vi "AcqControl.vi"(3 "Debug Mode?":bool, 4 "Digitizer Settings":T13={"Digitizer delay (us) "=0.0, "rf points per line"=2048, "lines per plane"=128, "Samp Rate (Hz)"=100000000.0, "Additional dig delay (us)"=0.0, "Voltage Scale"=0.4, "Pre-Looks"=0, "Offset delay (us)"=0.0, "bits A/D"=8, "Avg Num"=1, "DigTimeOut"=5.0, "Rel Dig Delay"=0.0, "Dig Ch"=0, "LeCroyCluster"={"LeCroy Channels"=[TRUE, FALSE, FALSE, FALSE], "LC read pt offset"=0.0, "Sweep Avg"=FALSE}, "Main Digitizer"=enum."NI Digitizer", "Dig Config"=enum."Single channel", "Digitizer ID Cluster"={"Acqiris/Alazar/SP ID"=[], "NI Instr Handles"=[], "LeCroy VISA"="", "GaGe Handle"={"Handle"=0, "Sample size"=0, "Resolution"=0, "Offset"=0, "Channels"=0, "Boards"=0}, "ATS Ref"="ATS9350", "Acqiris Address"=["PCI::INSTR0"], "ADQRef"=refnum, "adq_cu_ptr"=refnum}, "Trigger Settings"={"Trig Source"=1, "Trig Coupling"=0, "Trig Slope"=0, "Level (mV)"=1500.0}, "Bulk Acq"=FALSE, "Bulk Start Indexes"=[], "Data Ref RF"=refnum, "NI ID/Channel"=[], "Total Dig CH"=1, "Xtra Ann Trig delay (us)"=10.0, "Fix Z Delay?"=FALSE, "One Way Transmission?"=FALSE, "Data Ref Log"=refnum} {"Trigger Settings"."Trig Slope" items=["Positive", "Negative"]; "Trigger Settings"."Level (mV)" format="%.2f"; "Trigger Settings"."Trig Coupling" items=["DC 1 MOhm", "AC 1 MOhm", "DC 50 Ohm", "AC 50 Ohm"]; "Trigger Settings"."Trig Source" items=["Chan 1", "External"]; "Rel Dig Delay" format="%.2f"; "DigTimeOut" format="%.2f"; "Avg Num" min=1; "Offset delay (us)" format="%.2f"; "Additional dig delay (us)" format="%.2f"; "Digitizer delay (us)" format="%.2f"}, 5 "Motion Settings In":T10={"No Motion?"=FALSE, "Motion System"=enum."NI 735x", "Motion Bd ID"=1, "Motion Profile"="SMAC1", "# Axis"=1, "Reverse Z axis?"=TRUE, "SMAC Axis"=0, "scan pair"=enum."y-(x) scan", "RT fps"=6.0, "Steps per mm"=[1000, 1000, 1000, 1000], "Motor Parameters"={"velocity ct/s"=[10000.0, 10000.0, 10000.0, 50000.0], "accel ct/s^2"=[50000.0, 50000.0, 50000.0, 200000.0]}, "One Way Scan"=FALSE, "Reverse One Way Scan"=FALSE, "Global Position (mm)"=[], "Plane"=0, "Distance between\nscan lines (um)"=0.0, "Distance between\nscan planes (um)"=0.0, "number of scan planes"=1, "Total steps in line"=0, "Xtra plane\ndistance  (um)"=100, "Xtra planes "=1, "Add Axis"=FALSE, "overshoot cts"=200, "BKPT Shift"=0, "Scan Start Time (ms)"=0, "ESP VISA"="GPIB::1::INSTR", "3rd Axis"=1, "GL Ref Out"=refnum, "Galil Address"=""} {"3rd Axis" items=["x", "y", "z", "w"]; "Xtra planes" min=1; "Xtra plane\ndistance  (um)" min=0; "Distance between\nscan planes (um)" format="%.2f"; "Distance between\nscan lines (um)" format="%.2f"; "SMAC Axis" items=["None"=0, "Axis 1"=1, "Axis 2"=2, "Axis 3"=3, "Axis 4"=4, "Axis 5"=5, "Axis 6"=6, "Axis 7"=7, "Axis 8"=8, "Vector Space 1"=17, "Vector Space 2"=18, "Vector Space 3"=19, "Vector Space 4"=20]; "Motion Bd ID" min=1 max=32 step=1}) -> (1 "Digitizer Settings Out":T13={"Digitizer delay (us) "=0.0, "rf points per line"=2048, "lines per plane"=128, "Samp Rate (Hz)"=100000000.0, "Additional dig delay (us)"=0.0, "Voltage Scale"=0.4, "Pre-Looks"=0, "Offset delay (us)"=0.0, "bits A/D"=8, "Avg Num"=1, "DigTimeOut"=5.0, "Rel Dig Delay"=0.0, "Dig Ch"=0, "LeCroyCluster"={"LeCroy Channels"=[TRUE, FALSE, FALSE, FALSE], "LC read pt offset"=0.0, "Sweep Avg"=FALSE}, "Main Digitizer"=enum."NI Digitizer", "Dig Config"=enum."Single channel", "Digitizer ID Cluster"={"Acqiris/Alazar/SP ID"=[], "NI Instr Handles"=[], "LeCroy VISA"="", "GaGe Handle"={"Handle"=0, "Sample size"=0, "Resolution"=0, "Offset"=0, "Channels"=0, "Boards"=0}, "ATS Ref"="ATS9350", "Acqiris Address"=["PCI::INSTR0"], "ADQRef"=refnum, "adq_cu_ptr"=refnum}, "Trigger Settings"={"Trig Source"=1, "Trig Coupling"=0, "Trig Slope"=0, "Level (mV)"=1500.0}, "Bulk Acq"=FALSE, "Bulk Start Indexes"=[], "Data Ref RF"=refnum, "NI ID/Channel"=[], "Total Dig CH"=1, "Xtra Ann Trig delay (us)"=10.0, "Fix Z Delay?"=FALSE, "One Way Transmission?"=FALSE, "Data Ref Log"=refnum} {"Trigger Settings"."Trig Slope" items=["Positive", "Negative"]; "Trigger Settings"."Level (mV)" format="%.2f"; "Trigger Settings"."Trig Coupling" items=["DC 1 MOhm", "AC 1 MOhm", "DC 50 Ohm", "AC 50 Ohm"]; "Trigger Settings"."Trig Source" items=["Chan 1", "External"]; "Rel Dig Delay" format="%.2f"; "DigTimeOut" format="%.2f"; "Avg Num" min=1; "Offset delay (us)" format="%.2f"; "Additional dig delay (us)" format="%.2f"; "Digitizer delay (us)" format="%.2f"}, 2 "Motion Settings Out":T10={"No Motion?"=FALSE, "Motion System"=enum."NI 735x", "Motion Bd ID"=1, "Motion Profile"="SMAC1", "# Axis"=1, "Reverse Z axis?"=TRUE, "SMAC Axis"=0, "scan pair"=enum."y-(x) scan", "RT fps"=6.0, "Steps per mm"=[1000, 1000, 1000, 1000], "Motor Parameters"={"velocity ct/s"=[10000.0, 10000.0, 10000.0, 50000.0], "accel ct/s^2"=[50000.0, 50000.0, 50000.0, 200000.0]}, "One Way Scan"=FALSE, "Reverse One Way Scan"=FALSE, "Global Position (mm)"=[], "Plane"=0, "Distance between\nscan lines (um)"=0.0, "Distance between\nscan planes (um)"=0.0, "number of scan planes"=1, "Total steps in line"=0, "Xtra plane\ndistance  (um)"=100, "Xtra planes "=1, "Add Axis"=FALSE, "overshoot cts"=200, "BKPT Shift"=0, "Scan Start Time (ms)"=0, "ESP VISA"="GPIB::1::INSTR", "3rd Axis"=1, "GL Ref Out"=refnum, "Galil Address"=""} {"3rd Axis" items=["x", "y", "z", "w"]; "Xtra planes" min=1; "Xtra plane\ndistance  (um)" min=0; "Distance between\nscan planes (um)" format="%.2f"; "Distance between\nscan lines (um)" format="%.2f"; "SMAC Axis" items=["None"=0, "Axis 1"=1, "Axis 2"=2, "Axis 3"=3, "Axis 4"=4, "Axis 5"=5, "Axis 6"=6, "Axis 7"=7, "Axis 8"=8, "Vector Space 1"=17, "Vector Space 2"=18, "Vector Space 3"=19, "Vector Space 4"=20]; "Motion Bd ID" min=1 max=32 step=1})   [LabVIEW 2022 SP3]
uses:
  Controls/ScanType2.ctl
  Motion Controllers/-MotionRoutines/ScanAxis.ctl
  ViewData/-ReadEye/ScaleMethod.ctl
  ViewData/-ReadEye/TypeDefs/TypeofMean.ctl
  Digitizers/-DigitizerRoutines/DigitizerSettings.ctl
  Digitizers/-DigitizerRoutines/Digitizer.ctl
  Digitizers/-DigitizerRoutines/DigConfig.ctl
  Digitizers/-DigitizerRoutines/DigitizerID.ctl
  C:/Windows/System32/ADQAPI_dotNet_helper.dll
  Motion Controllers/NI_controller/-NI_MotionRoutines/MotionParameters.ctl
  Motion Controllers/NI_controller/-NI_MotionRoutines/MotionSys.ctl
  Motion Controllers/-MotionRoutines/3rdAxis.ctl
  Annular Array/-AnnularRoutines/TransGeometry.ctl
  Annular Array/-AnnularRoutines/ArrayGeometry.ctl
  Controls/HF_XDCRs.ctl
  TransducerCal/-CalTransducer/HydrophoneSettings.ctl
  TransducerCal/-CalTransducer/Hydros.ctl
  <vilib>/Utility/miscctls.llb/LVRectTypeDef.ctl
  Controls/location.ctl
  <vilib>/Analysis/baseanly.llb/Quick Scale 2D.vi
  Motion Controllers/-MotionRoutines/MotionGlobals.vi
  Switch Modules/SwitchGlobals.vi
  Annular Array/-AnnularRoutines/AnnularArrayGlobal.vi
  Pulsers/PulserGlobals.vi
  Digitizers/-DigitizerRoutines/DigitizerGlobals.vi
  <vilib>/DAQmx/create/channels.llb/DAQmx Create Channel (CO-Pulse Generation-Frequency).vi
  <vilib>/DAQmx/configure/timing.llb/DAQmx Timing (Implicit).vi
  <vilib>/Analysis/NI_AALBase.lvlib
  <vilib>/Platform/NI_3dgraph.lvlib
  <instrlib>/niSwitch/niSwitch.llb/niSwitch Connect Channels (Single).vi
panel:
  out "Length of\nall planes (mm) Temp":dbl=128.0 format="%.2f"
  out "Digitizer delay (us) (Temp)":dbl
  in  "Auto Vz Depth":dbl=0.04 format="%.2f"
  in  "Pulse":bool
  in  "Length of Z \nScan (mm)":dbl=4.0 format="%#_13g"
  in  "Distance between\nZ planes (um)":i32=50
  in  "DBSP2":sgl
  in  "DBSP1":sgl
  out "Scan Size":dbl[](array[numeric])
  in  "Attenuation Scan":bool
  in  "Parameter Selection":u16(ring) items=["Neg Peak (V)", "Pos Peak  (V)", "Peak to Peak  (V)", "RMS  (V)", "Neg Peak Pressure (MPa)", "p.3 (MPa)", "Ipa (W/cm^2)", "Ipa.3 (W/cm^2)", "Ita (W/cm^2)", "Ita.3 (W/cm^2)"]
  out "Scan data":T1 {"Pulse Parameters"."pos peak pressure (MPa)" format="%.2f"; "axis 2 ticks" format="%.2f"; "axis 1 ticks" format="%.2f"; "step size" format="%.2f"; "axis2o" format="%.2f"; "axis1o" format="%.2f"; "scan data" format="%.2f"}
  in  "Pressure Cal Parameters":T2={"Center Freq (MHz)"=0.0, "PRF (kHz)"=1.0, "Pulse window (us)"=0.0, "Hydrophone"=enum."PAL #1048", "booster amp?"=TRUE} {"Pulse window (us)" format="%.2f"; "PRF (kHz)" format="%.2f"; "Center Freq (MHz)" format="%.2f"}
  in  "Plot":enum32{"1-D", "2-D"}(tab)
  out "Hydrophopne Waveform Graph":T4(graph)
  in  "3D Surface":refnum<k7>(container)
  in  "3rd Axis":T5=1 items=["x", "y", "z", "w"]
  in  "Fill":bool
  in  "1-to-1":bool
  in  "Auto Vz?":bool=TRUE
  out "LC read pt offset temp":dbl
  out "rf points per line Temp":i32
  out "Additional dig delay (us) Temp":dbl
  in  "New Sample":bool
  in  "Next Scan":bool
  in  "HF XDCR":T6
  in  "Microscopy Scan Mode":T7(radio)
  in  "Take Webcam pic":bool
  in  "Save Scan Settings":bool
  in  "Load Scan Settings":bool
  in  "Flip Y":bool
  in  "Flip X":bool
  in  "Transpose":bool
  in  "Trans Geometry (mm)":T8={"Transducer"=0, "Geo Focus"=12.0, "a (radius)"=3.0, "# of rings"=5, "kerf space "=0.1, "Center Freq"=12.0} {"Transducer" items=["6D 12R 40 MHz"=0, "10D 31R 20 MHz"=1, "10D 23R 20 MHz"=2, "6D 23R 40 MHz"=3, "4.5D 10.7R 40 MHz"=4, "9D 23.5R 20 MHz"=5, "9D 25.8R 20MHz"=6, "Enter"=99]}
  out "error out":errorcluster
  in  "2nd Channel HZ Offset?":bool
  in  "Read HZ Offset?":bool
  in  "Reverse One \nWay Scan":bool
  in  "Skip Real Time Setup":bool
  in  "VISA session 2":refnum<visa-resource-name>
  out "Cross plane\nlength (mm)":dbl=128.0 format="%.2f"
  in  "Xtra planes":i32=1 min=1
  in  "Xtra plane\ndistance  (um)":i32=100 min=0
  out "File":string
  in  "Filter Prams":T17={"low cutoff"=25, "order"=81, "high cutoff"=55}
  in  "OPTIONS":T18(tab)=enum."Array Other"
  in  "View EYE":bool
  in  "CH2?":bool
  out "RT V":i32
  out "Trig (Hz)":dbl
  in  "Compress":bool
  in  "C MIP":bool
  in  "MIP Thresh":sgl=15.0
  in  "Multi Trig#":i32=1 min=1
  in  "Multi Trig":bool
  in  "Multi Time (us)":sgl=250.0 min=250
  in  "Resp Wait (ms)":u32=400
  in  "Dopp\nGate?":bool
  in  "Add Axis":bool
  in  "Resp Divide":i32=2 min=1
  in  "USB Gate\nPer Sample":bool
  in  "Transfer to FTP":bool
  in  "DAQ Range":cluster{"Max V":dbl, "Min V":dbl}={"Max V"=1.0, "Min V"=-1.0} {"Max V" format="%0.2f"; "Min V" format="%0.2f"}
  in  "LeCroy Channels":bool[](array[boolean])=[TRUE, FALSE, FALSE, FALSE]
  in  "CTR PRF?":bool=TRUE
  in  "Save Temp":bool
  in  "Sweep\nAvg":bool
  in  "c mm/mics":sgl=1.485
  in  "Bulk Acq":bool
  in  "Full Array Scan?":bool
  in  "BKPT Shift":i32
  in  "Xtra delay (us)":dbl=3.0
  in  "Sub Ap Excite?":bool
  in  "RT fps":sgl=12.0 min=0.001 max=30 format="%#_2f"
  in  "Xmt/Rcv":cluster{"XMIT":bool[], "RCV":bool[]}={"XMIT"=[TRUE, TRUE, TRUE, TRUE, TRUE], "RCV"=[TRUE, TRUE, TRUE, TRUE, TRUE]}
  in  "Save TIFF?":bool
  in  "GPU?":bool
  in  "DownFactor":i32=1 min=1
  in  "RCV 1CH":u16(ring) items=["All", "1", "2", "3", "4", "5"]
  in  "Set Spectrometer":bool
  in  "Overshoot":i32=200 min=0 max=10000
  in  "One Way Scan":bool
  in  "TimeOut (s)":sgl=5.0 min=0 format="%_2f"
  in  "scan pair":T12=enum."x-(y) scan"
  out "View path":path
  in  "Type of Mean":T19=enum."No mean"
  in  "Display mode":T20=enum."Log Grey Scale"
  in  "distance?":bool
  in  "ExitSendCmd":bool
  in  "Email":string
  in  "Drive Voltages":sgl[](array[numeric])=[100.0] format="%#_3g"
  in  "Burst Ct":i8[](array[numeric])=[10, 15, 20]
  in  "CA Threshold":i16=15
  in  "Focal Zones":i16=41
  in  "Fix Z Delay?":bool
  out "Estimated Line spacing":dbl=1.0
  in  "Man Cont":bool
  in  "Auto\nScale":bool=TRUE
  out "Waveform Graph":sgl[](graph)
  in  "SetDig":bool
  in  "Synth Foc?":bool
  in  "Avg Num":i32=1 min=-1
  in  "Transducer":u32 min=1 max=5 step=1
  in  "Pre-Looks":i32=50
  in  "Sector Angle":i32(slide)=360 min=0 max=360 step=45 scale=0.0..360.0
  in  "Rot lines per plane":u16(ring)=128 items=["50", "100", "200", "250", "400", "500", "1000"]
  out "Total Pts":bool=TRUE
  in  "Keep?":bool=TRUE
  in  "Show Thumbs":bool
  in  "Erase data":bool
  in  "Save Data":bool
  in  "Type of scan":T21=enum."M scan"
  in  "Therapy Parameters":T22={"Theraputic Freq (MHz)"=0.1, "Time on (s)"=1.0, "Therapy amplitude (mV)"=50.0, "Lines Before"=20, "Lines After"=80} {"Therapy amplitude (mV)" min=10.0 max=1000.0 format="%.2f"; "Time on (s)" format="%.1e"; "Theraputic Freq (MHz)" format="%.3f"}
  in  "Case temp":string
  in  "Case Name":string="Case"
  in  "Case to View":u16(ring) items=["Case"]
  in  "Length of\nall planes (mm)":dbl=128.0 format="%.2f"
  in  "Scan to View":u32
  out "Raw data":dbl[][](graph)
  out "Digitzer Error Message":string
  in  "Set Pulser":bool
  in  "lines per plane":u16=128 min=1
  in  "number of planes":u16=1
  out "Time between\n samples (ms)":dbl=1.0 format="%.3f"
  in  "prf (kHz)":dbl=1.0 min=0.001 format="%.3f"
  in  "start scan":bool
  in  "Distance between\nplanes (um)":sgl=100.0 min=0.1 step=0.1
  in  "Length of\none plane (mm)":dbl=8.0 format="%.2f"
  in  "Distance between\nscan lines (um)":sgl=100.0 min=0.1 step=0.1
  # "© 2000-2022 Weill Cornell"
  # "1-D and 2-D B scan settings"
  # "1-D and 2-D B scan settings"
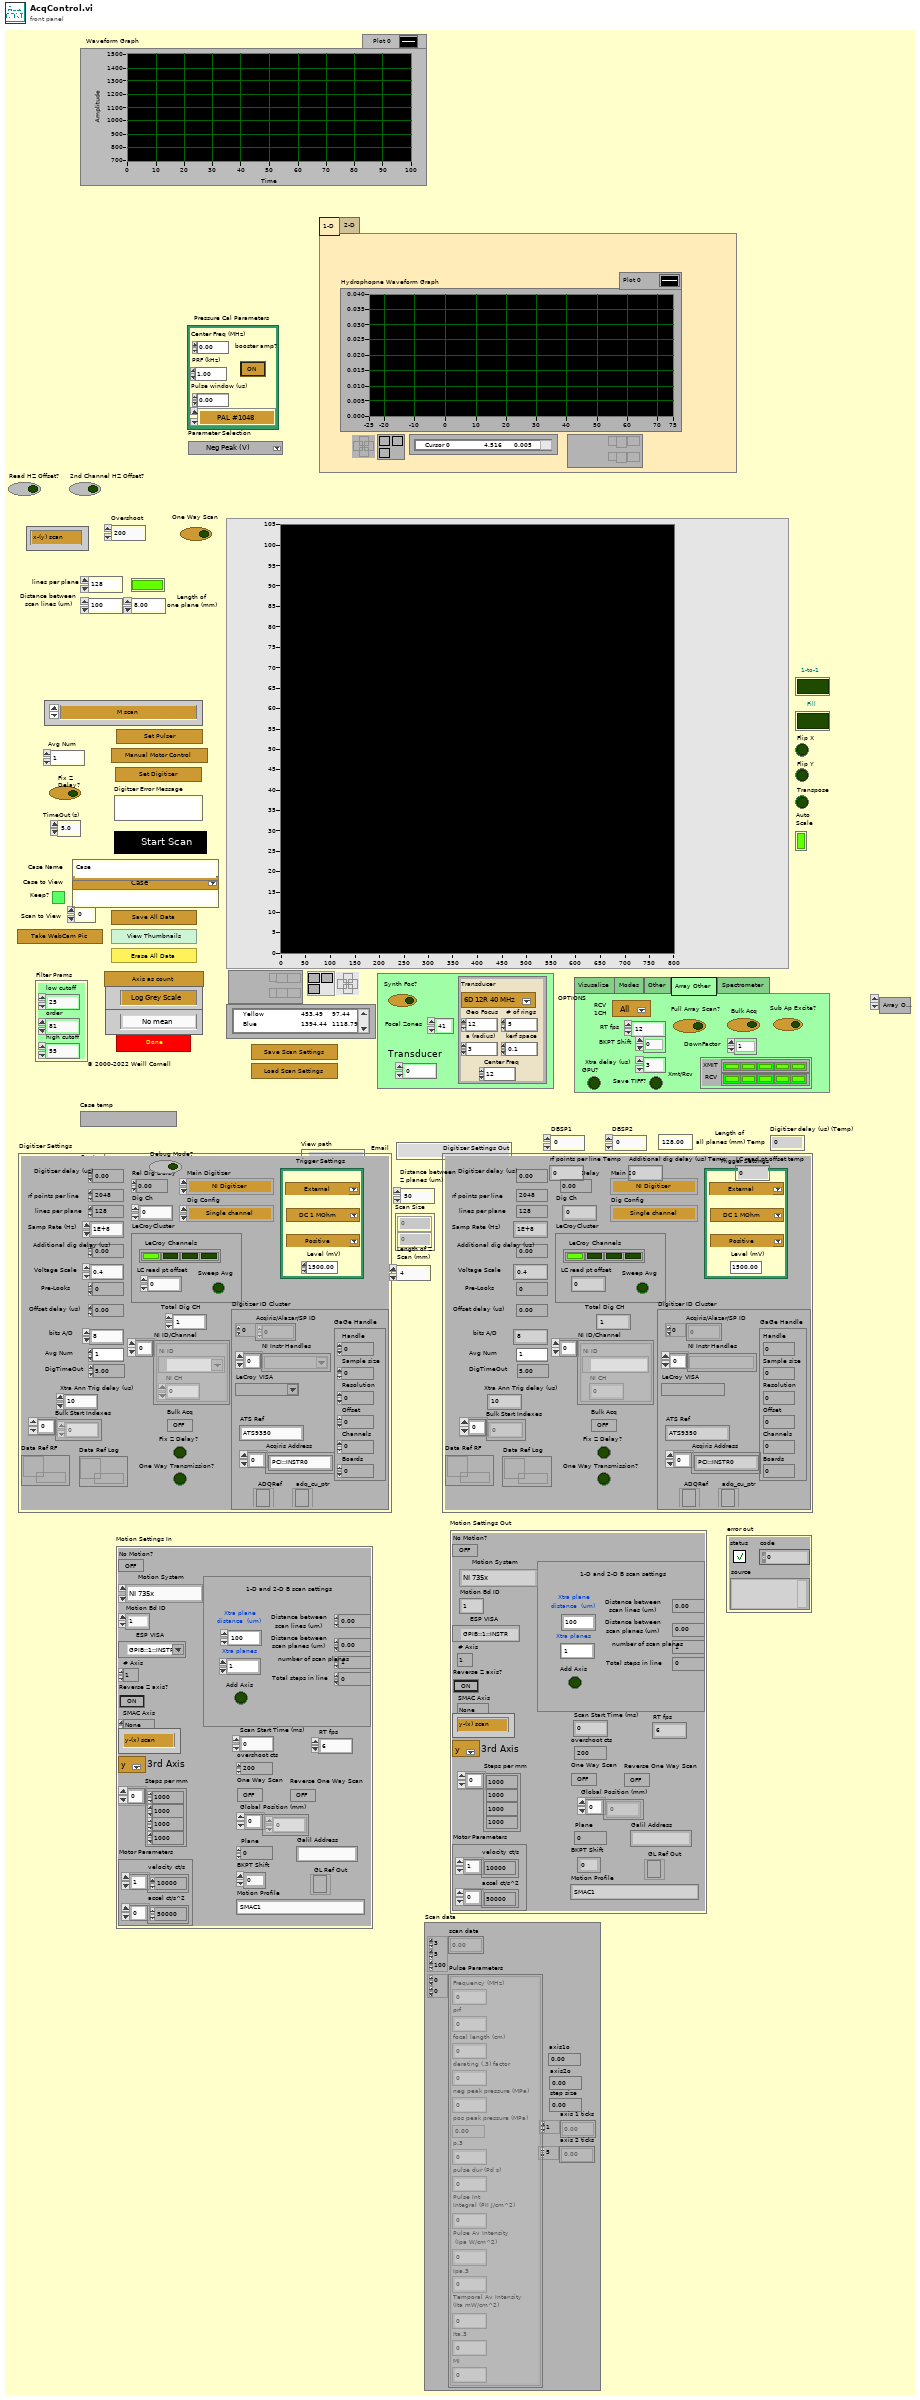
[diagram p1: front panel]
types:
  T1 = cluster{"scan data":dbl[][][], "Pulse Parameters":cluster{"Frequency (MHz)":dbl, "prf":dbl, "focal length (cm)":dbl, "derating (.3) factor":dbl, "neg peak pressure (MPa)":dbl, "pos peak pressure (MPa)":dbl, "p.3":dbl, "pulse dur (Pd s)":dbl, "Pulse Int \nIntegral (PII J/cm^2)":dbl, "Pulse Av Intensity\n (Ipa W/cm^2)":dbl, "Ipa.3":dbl, "Temporal Av Intensity \n(Ita mW/cm^2)":dbl, "Ita.3":dbl, "MI":dbl}[][], "axis1o":dbl, "axis2o":dbl, "step size":dbl, "axis 1 ticks":dbl[], "axis 2 ticks":dbl[]}
  T2 = typedef "HydrophoneSettings.ctl" = cluster{"Center Freq (MHz)":dbl, "PRF (kHz)":dbl, "Pulse window (us)":dbl, "Hydrophone":T3, "booster amp?":bool}
  T3 = typedef "Hydros.ctl" = enum16{"PAL #1048", "PAL #525", "PAL #430a", "PAL #192", "DEAD PAL # 1403", "LOST UHI Onda", "DEAD PAL #1818", "PAL #1974", "DEAD #2266 w/booster", "PAL #2524 w/booster", "PAL FP21-20T", "PAL FP160-13  ", "PAL FP141-20", "PAL FP158-08T"}
  T4 = cluster{"axis1o":dbl, "step size":dbl, "data out":dbl[]}
  T5 = typedef "3rdAxis.ctl" = u16
  T6 = typedef "HF_XDCRs.ctl" = enum16{"250 MHz", "500 MHz"}
  T7 = enum32{"Level X", "Level Y", "Overview Scan", "Detailed Scan", "V-Z Scan"}
  T8 = typedef "TransGeometry.ctl" = cluster{"Transducer":T9, "Geo Focus":dbl, "a (radius)":dbl, "# of rings":i32, "kerf space ":dbl, "Center Freq":dbl}
  T9 = typedef "ArrayGeometry.ctl" = u16
  T10 = typedef "MotionParameters.ctl" = cluster{"No Motion?":bool, "Motion System":T11, "Motion Bd ID":u8, "Motion Profile":string, "# Axis":i8, "Reverse Z axis?":bool, "SMAC Axis":u16, "scan pair":T12, "RT fps":sgl, "Steps per mm":i32[], "Motor Parameters":cluster{"velocity ct/s":dbl[], "accel ct/s^2":dbl[]}, "One Way Scan":bool, "Reverse One Way Scan":bool, "Global Position (mm)":dbl[], "Plane":i32, "Distance between\nscan lines (um)":sgl, "Distance between\nscan planes (um)":sgl, "number of scan planes":i32, "Total steps in line":i32, "Xtra plane\ndistance  (um)":i32, "Xtra planes ":i32, "Add Axis":bool, "overshoot cts":i32, "BKPT Shift":i32, "Scan Start Time (ms)":u32, "ESP VISA":refnum<visa-resource-name>, "3rd Axis":T5, "GL Ref Out":refnum<k7>, "Galil Address":string}
  T11 = typedef "MotionSys.ctl" = enum16{"MM3000", "NI 735x", "Newport ESP", "No Motion Card", "Galil"}
  T12 = typedef "ScanAxis.ctl" = enum16{"y-(x) scan", "x-(y) scan", "z-(x) scan", "z-(y) scan", "y-(z) scan", "x-(z) scan", "w-(x) scan", "w-(y) scan", "w-(z) scan", "x-(w) scan", "y-(w) scan", "z-(w) scan"}
  T13 = typedef "DigitizerSettings.ctl" = cluster{"Digitizer delay (us) ":dbl, "rf points per line":i32, "lines per plane":i32, "Samp Rate (Hz)":dbl, "Additional dig delay (us)":dbl, "Voltage Scale":dbl, "Pre-Looks":i32, "Offset delay (us)":dbl, "bits A/D":i8, "Avg Num":i32, "DigTimeOut":sgl, "Rel Dig Delay":sgl, "Dig Ch":i32, "LeCroyCluster":cluster{"LeCroy Channels":bool[], "LC read pt offset":dbl, "Sweep Avg":bool}, "Main Digitizer":T14, "Dig Config":T15, "Digitizer ID Cluster":T16, "Trigger Settings":cluster{"Trig Source":u16, "Trig Coupling":u16, "Trig Slope":u16, "Level (mV)":dbl}, "Bulk Acq":bool, "Bulk Start Indexes":i32[], "Data Ref RF":refnum<data-value>, "NI ID/Channel":cluster{"NI ID":refnum<k15>, "NI CH":i32}[], "Total Dig CH":i32, "Xtra Ann Trig delay (us)":dbl, "Fix Z Delay?":bool, "One Way Transmission?":bool, "Data Ref Log":refnum<data-value>}
  T14 = typedef "Digitizer.ctl" = enum16{"Acqiris Digitizer", "NI Digitizer", "LeCroy", "GaGe", "AlazarTech", "No Digitizer", "Teledyne"}
  T15 = typedef "DigConfig.ctl" = enum16{"Single channel", "2 Chans w/ 2 Acqiris", "2 Chans w/ 1 Acqiris", "5-CH Pulser New", "5-CH pulser w/ ann array", "5-pass style ann array", "Empty"}
  T16 = typedef "DigitizerID.ctl" = cluster{"Acqiris/Alazar/SP ID":u32[], "NI Instr Handles":refnum<k15>[], "LeCroy VISA":refnum<visa-resource-name>, "GaGe Handle":cluster{"Handle":u32, "Sample size":u32, "Resolution":i32, "Offset":i32, "Channels":u32, "Boards":u32}, "ATS Ref":string, "Acqiris Address":string[], "ADQRef":refnum<k24>, "adq_cu_ptr":refnum<k24>}
  T17 = cluster{"low cutoff":i32, "order":i32, "high cutoff":i32}
  T18 = enum32{"Visusalize", "Modes", "Other", "Array Other", "Spectrometer"}
  T19 = typedef "TypeofMean.ctl" = enum16{"Mean from lines", "Mean just lines", "Poly Mean", "No mean", "Filter"}
  T20 = typedef "ScaleMethod.ctl" = enum16{"Linear Abs Grey", "Log Grey Scale", "Linear Color Scale", "dB Scale", "Verasonics Doppler"}
  T21 = typedef "ScanType2.ctl" = enum16{"Therapy With Scan", "M scan", "M Scan With Therapy Burst", "1-D B Scan", "1-D B Scan With Therapy Burst", "2-D B Scan", "2-D B Scan With Therapy Burst", "Rotational Scan", "1-D B-Scan PRF", "2-D B-Scan PRF", "Real-Time Scan", "Contrast Agents", "1-D w/ Real-Time Set Up", "Dual Transducer", "Acoustic Microscopy", "Hydrophone Scanning"}
  T22 = cluster{"Theraputic Freq (MHz)":dbl, "Time on (s)":dbl, "Therapy amplitude (mV)":dbl, "Lines Before":i16, "Lines After":i16}
  T23 = typedef "LVRectTypeDef.ctl" = cluster{"Left":i16, "Top":i16, "Right":i16, "Bottom":i16}
  T24 = typedef "Dual XDCR Complete Settings.ctl" = cluster{"Scan Size":dbl[], "XDCR Offset":dbl[], "Found Home":bool, "XDCR Settings":T25[]}
  T25 = typedef "XDCRSettings.ctl" = cluster{"Transducer Name":string, "Motion Settings":cluster{"Distance between\nscan lines (um)":sgl, "Distance between\nscan planes (um)":sgl}, "Digitizer Settings":cluster{"RF data Sampling":cluster{"Sampling Rate":dbl, "Ref Delay (ms)":dbl, "rf points per line":i32}, "Time scale per Div":dbl, "Voltage Scale":dbl, "Additional dig delay (ms)":dbl}, "Filter Prams":cluster{"low cutoff":i32, "order":i32, "high cutoff":i32}, "XDCR Focal Length":dbl, "Data Vertical Center":dbl, "Image Vertical Offset":dbl, "Daxsonics Settings":T26, "Panametrics Settings":T27, "JSR Complete":T28, "UT340 Controls":T43}
  T26 = typedef "Dax_Control_Cluster.ctl" = cluster{"Freq (MHz) ":u16, "Voltage (V)":u16, "Gain (dB)":u16}
  T27 = typedef "Pana5900.ctl" = cluster{"ENERGY (uJ)":u16, "DAMPING (Ohm)":u16, "HP FILT (KHz) ":u16, "LP FILT (MHz)":u16, "MODE":u16, "PRF (KHz)":u16, "GAIN (db)":u16, "COARSE ATTENUATION":u16, "FINE ATTENUATION":u16}
  T28 = typedef "JSR Complete.ctl" = cluster{"JSR Pulse Settings":T29, "JSR Receive Settings":T34, "JSR Trigger Settings":T39}
  T29 = typedef "JSR Pulse.ctl" = cluster{"Damping":T30, "Pulse Energy Level":T31, "Pulser Impedance":T32, "Pulser Voltage (V)":T33}
  T30 = typedef "Damping.ctl" = i16
  T31 = typedef "Energy.ctl" = u16
  T32 = typedef "Z.ctl" = u16
  T33 = typedef "Volt.ctl" = i16
  T34 = typedef "JSR Recieve.ctl" = cluster{"Receiver Mode":T35, "High Pass Filter":T36, "Low Pass Filter":T37, "Gain (dB)":T38}
  T35 = typedef "Mode.ctl" = i8
  T36 = typedef "HPF.ctl" = u16
  T37 = typedef "LPF.ctl" = u16
  T38 = typedef "Gain.ctl" = i8
  T39 = typedef "JSR Trigger.ctl" = cluster{"External Trigger Limit":T40, "Trigger Source":T41, "PRF (Hz)":T42}
  T40 = typedef "Trig Limit.ctl" = i8
  T41 = typedef "Trig Source.ctl" = i8
  T42 = typedef "PRF.ctl" = dbl
  T43 = typedef "UTEX Controls.ctl" = cluster{"High Pass On":bool, "High Pass Filter (MHz)":i16, "Low Pass On":bool, "Low Pass Filter (MHz)":i16, "PE Gain (dB)":i16, "Voltage":i16, "Pulse Width (ns)":dbl, "Mode":bool, "PC Gain (dB)":i16, "Trig Source":bool, "Rep Rate (Hz)":i16, "PULSE":bool}
  T44 = typedef "location.ctl" = enum16{"Automatic", "WCM Main", "Hawaii", "Columbia MM3000", "Columbia  NI System", "NYU", "RRI 2", "UHI Allen", "CUMC RT", "Chiba", "Stony Brook", "WCM Microscopy", "WCM Aeoretch", "WCM Optics Lab", "WCM Main 2Axis", "WCM Rotation", "WCM SAM SMAC", "SERI GP"}
  T45 = enum8{"Enabled", "Disabled", "Disabled and Grayed Out"}
  T46 = cluster{"yo":dbl, "dx":dbl, "output array":dbl[]}
  T47 = enum16{"Transducer 1", "Transducer 2", "Dual XDCR", "Exit"}
  T48 = cluster{"File Name":string, "Keep?":bool, "Synth Foc?":bool, "Microscopy Scan Mode":enum32{"Level X", "Level Y", "Overview Scan", "Detailed Scan", "V-Z Scan"}}[]
  T49 = enum16{"Absolute Position", "Relative Position", "Velocity", "Relative to Cap Pos", "Modulus Position", "Absolute Contouring", "Relative Contouring"}
  T50 = typedef "AnnularArray.ctl" = cluster{"Synth Foc?":bool, "Focal Zones":i16, "Switch T/R":i16, "Trans Geometry (mm)":T8, "Sub Ap Excite?":bool, "Full Array Scan?":bool, "Xmt/Rcv":cluster{"XMIT":bool[], "RCV":bool[]}, "PulseSpacing (us)":sgl, "Xmit Ring":i32, "XMIT CHS":u8, "RCV CHS":u8, "GPU?":bool, "Save TIFF?":bool, "downfactor":i32, "RCV 1CH":u16}
  T51 = typedef "SwitchOption.ctl" = enum16{"Cytex", "Pickering", "NI Switch", "No Switch", "Riverside USB"}
  T52 = typedef "EKG_Mode.ctl" = u16
  T53 = typedef "pulser.ctl" = enum16{"Pan 5900", "Daxsonics", "Agilent 33xxx", "UTEX", "JSR", "WMC Mono-Cycle", "No Pulser", "NYU AVTECH", "Tabor W1281A", "Pan 5800", "Unlisted", "Tabor WX2182B"}
  T54 = typedef "eventvkey.ctl" = enum16{"ASCII", "Enter", "Return", "Shift", "Ctrl", "Alt", "Cmd", "Opt", "Caps", "NumLock", "Clear", "Break", "Up", "Down", "Left", "Right", "Insert", "Delete", "Home", "End", "PageUp", "PageDown", "Escape", "Help", "Pause", "ScrollLock", "F1", "F2", "F3", "F4", "F5", "F6", "F7", "F8", "F9", "F10", "F11", "F12", "F13", "F14", "F15", "F16", "F17", "F18", "F19", "F20", "F21", "F22", "F23", "F24", "Play", "VolumeUp", "VolumeDown", "Mute", "Two Byte Char"}
  T55 = typedef "ScanParams.ctl" = cluster{"File Name":string, "Keep?":bool, "Synth Foc?":bool, "Microscopy Scan Mode":enum32{"Level X", "Level Y", "Overview Scan", "Detailed Scan", "V-Z Scan"}}
  T56 = typedef "Bd Id Out" = u8
  T57 = cluster{"lines per plane":refnum<vi>, "Distance between\nscan lines (um)":refnum<vi>, "Length of\none plane (mm)":refnum<vi>, "number of planes":refnum<vi>, "Distance between\nplanes (um)":refnum<vi>, "Length of\nall planes (mm)":refnum<vi>}
  T58 = cluster{"Frequency (MHz)":dbl, "prf":dbl, "focal length (cm)":dbl, "derating (.3) factor":dbl, "neg peak pressure (MPa)":dbl, "pos peak pressure (MPa)":dbl, "p.3":dbl, "pulse dur (Pd s)":dbl, "Pulse Int \nIntegral (PII J/cm^2)":dbl, "Pulse Av Intensity\n (Ipa W/cm^2)":dbl, "Ipa.3":dbl, "Temporal Av Intensity \n(Ita mW/cm^2)":dbl, "Ita.3":dbl, "MI":dbl}[][]
  T59 = typedef "Header.ctl" = cluster{"header info":cluster{"Header":string, "Head length":i16}, "A/D info":cluster{"# rf points per line":u16, "# lines per scan":u16, "sample rate MHz":u16, "# A/D bits":i16, "# bytes per A/D":u16, "TGC Flag":u16, "A/D Type":string}, "Tranducer Info":cluster{"bandwidth":sgl, "center freq":sgl, "start freq":sgl, "ID":i32}, "Scan Info":cluster{"delay":sgl, "pivot distance":sgl, "sector scan angle":sgl, "operator":string, "Scan Mode":string, "location":string}, "Time/Date Info":cluster{"date":string, "time":string}, "RF Info":cluster{"RF file name":string, "RF file att":string, "RF cal file name":string, "RF cal file att":string}, "Patient Info":cluster{"ID":string, "extended ID":string, "age":u16, "sex":string, "previously\nscanned":string, "PSA":sgl, "LOS":u8, "Ethnicty 2":u8, "Race":u8}, "Tissue Type":cluster{"organ":i16, "disease type":i16, "disease location":i16, "IQ_pts":u16, "RcvBuffer":u8, "RcvFrame":u16, "IQBuff":u8, "IQFrame":u16, "IQPage":u8}, "Votage scaling":cluster{"Digitizer (dB)":sgl, "Gain (dB)":sgl, "Atten (dB)":sgl}, "Comment":string, "Misc Info":cluster{"avg num":u16, "c speed":i16, "Div By or SF zones":i16, "XMIT CHS":u8, "RCV CHS":u8, "Xmit angle":sgl}, "Therapy Parameters":cluster{"Theraputic Freq (MHz)":sgl, "Time on (s)":sgl, "Therapy amplitude (mV)":sgl, "Lines Before":u16, "Lines After":u16}, "Scan Settings":cluster{"Energy (uJ or V)":u8, "Damp (Ohm) or Fc":u8, "HP Filt (KHz)":u8, "LP Filt (MHz)":u8, "Gain (db)":u8, "prf (kHz)":sgl, "Distance between\nscan lines (um)":u16, "Distance between\nscan planes (um)":u16, "Scan line gap (um)":sgl, "Scan plane gap (um)":sgl}, "Compression Parameters":cluster{"F1 (MHz)":sgl, "F2 (MHz)":sgl, "% taper":sgl, "duration":sgl}, "Patient Info Xtra":cluster{"First Name":string, "Last Name":string, "Notes":string}, "ROI Box":u16[]}
  T60 = typedef "LVBoundsTypeDef.ctl" = cluster{"Width":u32, "Height":u32}
  T61 = typedef "SpectrometerType.ctl" = u16
  T62 = cluster{"velocity ct/s":dbl[], "accel ct/s^2":dbl[]}
  T63 = cluster{"LeCroy Channels":bool[], "LC read pt offset":dbl, "Sweep Avg":bool}
  T64 = enum16{"Left Button", "Center Button", "Right Button", "Window Close"}
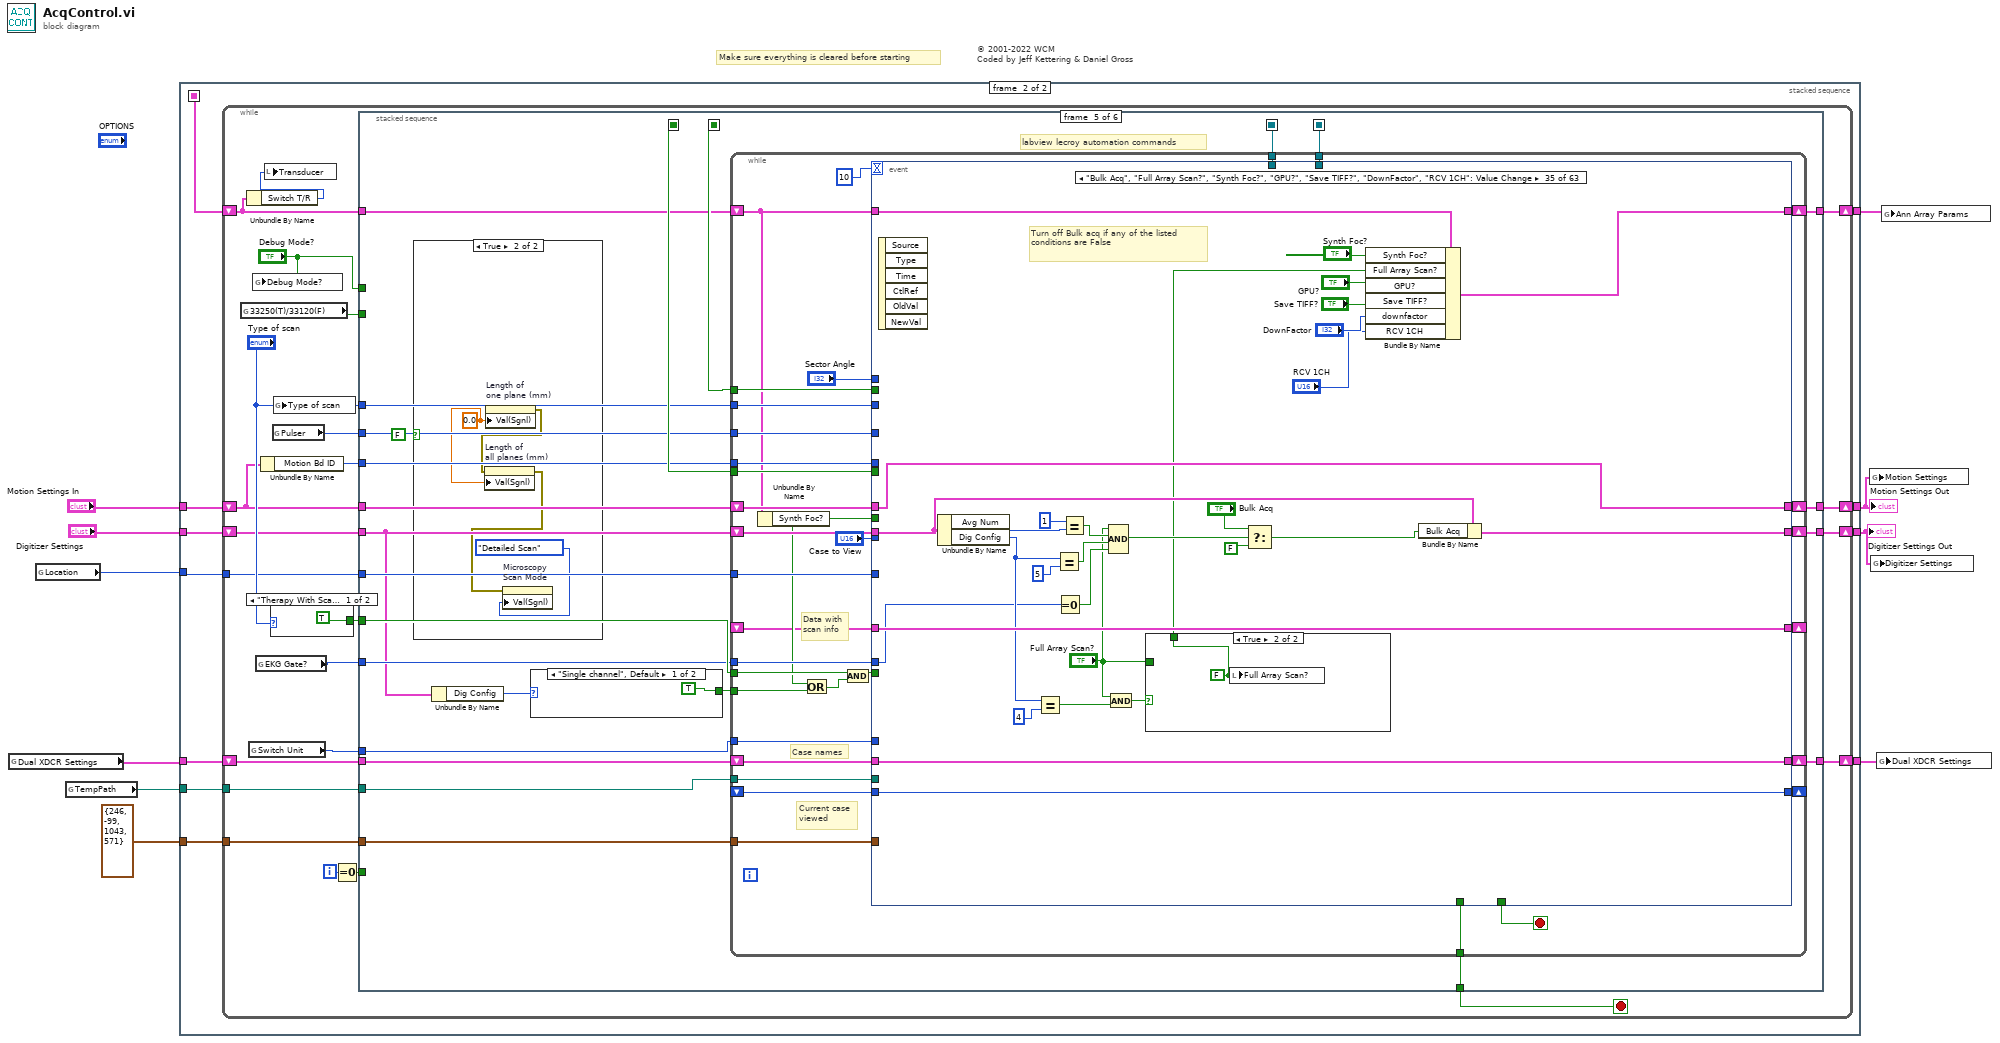
[diagram p0: block diagram]
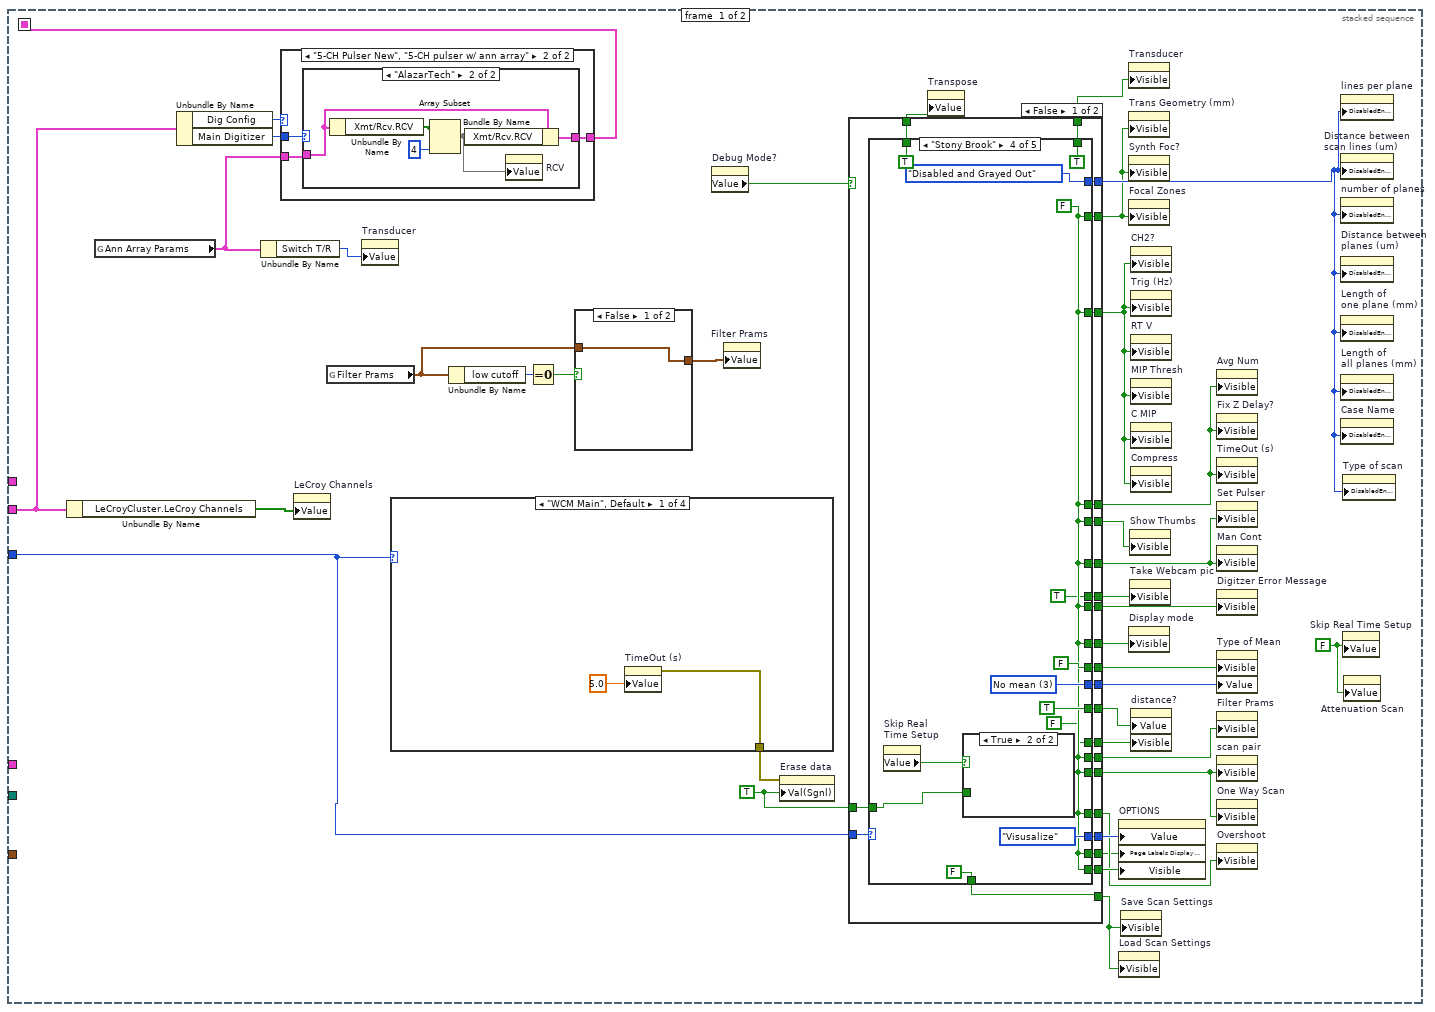
[diagram p2: hidden frame]
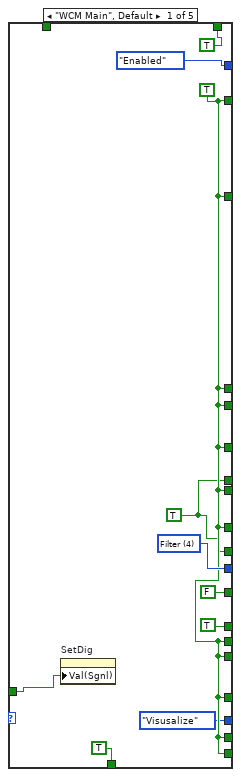
[diagram p5: hidden frame]
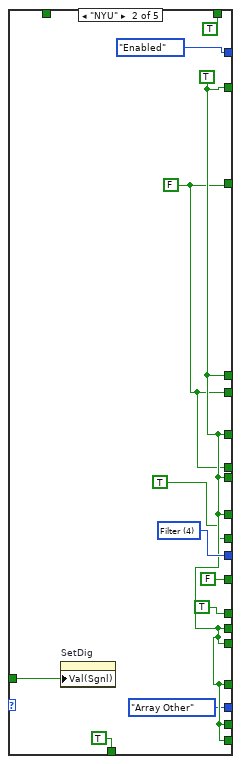
[diagram p6: hidden frame]
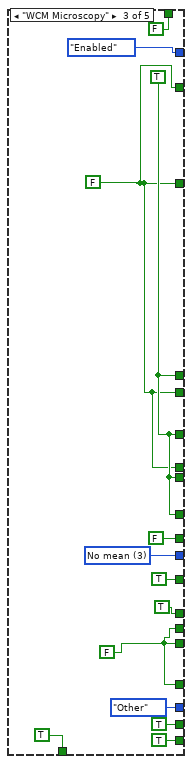
[diagram p7: hidden frame]
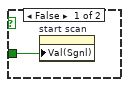
[diagram p8: hidden frame]
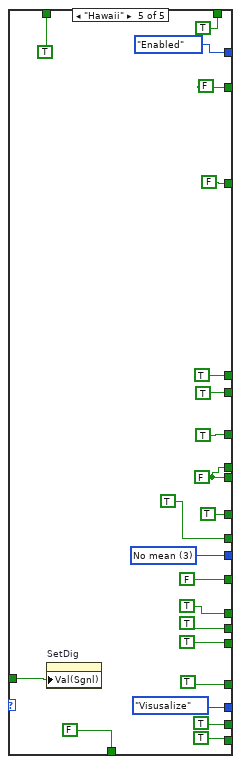
[diagram p9: hidden frame]
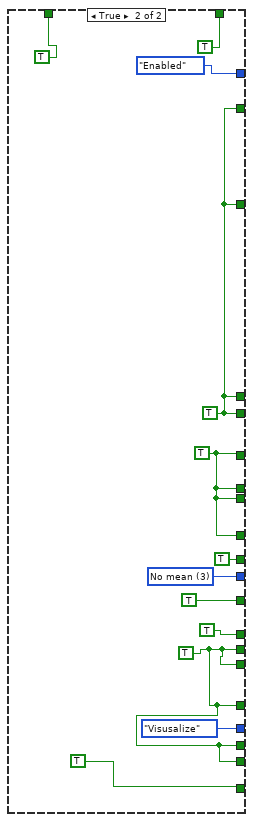
[diagram p10: hidden frame]
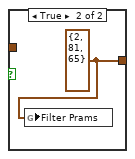
[diagram p11: hidden frame]
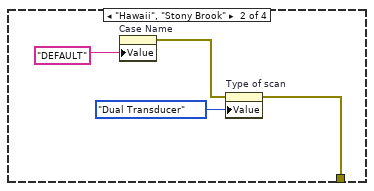
[diagram p12: hidden frame]
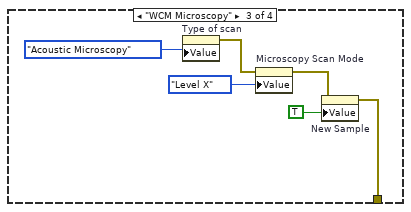
[diagram p13: hidden frame]
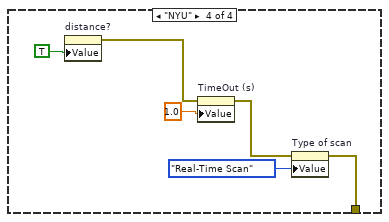
[diagram p14: hidden frame]
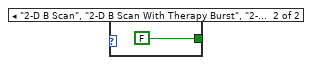
[diagram p15: hidden frame]
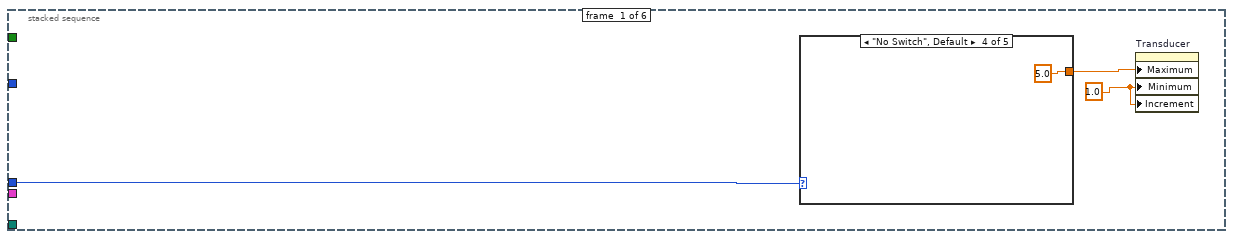
[diagram p16: hidden frame]
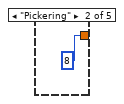
[diagram p18: hidden frame]
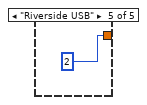
[diagram p20: hidden frame]
diagram:
  # "Make sure everything is cleared before starting"
  # "© 2001-2022 WCM\nCoded by Jeff Kettering & Daniel Gross"
  n1 = global read "SwitchGlobals.vi" "Dual XDCR Settings"() -> (w6:T24)
  n2 = global read "MotionGlobals.vi" "Location"() -> (w7:T44)
  n3 = global read "MotionGlobals.vi" "TempPath"() -> (w10:path)
  n4 = stacked-sequence {
    seq-local: [w11 _] -> [_ w185]
    tunnel: w10 -> [_ w195]
    tunnel: "Digitizer Settings" -> [w13 w194]
    tunnel: "Motion Settings In" -> [_ w193]
    tunnel: w7 -> [w48 w192]
    tunnel: w6 -> [_ w191]
    tunnel: [_ w190] -> w5
    tunnel: [_ w189] -> w4
    tunnel: [_ w188] -> w3
    tunnel: [_ w187] -> w2
    tunnel: T23 {"Left"=246, "Top"=-99, "Right"=1043, "Bottom"=571} ("Plot Area Bounds") -> [_ w186]
    frame #0 {
      w17 = FALSE
      w21 = TRUE ("Value (Signaling)")
      n5 = Unbundle By Name(w13) -> ("LeCroyCluster.LeCroy Channels"=w16:bool[])
      n6 = global read "AnnularArrayGlobal.vi" "Ann Array Params"() -> (w12:T50)
      n7 = Unbundle By Name(w13) -> ("Dig Config"=w15:T15, "Main Digitizer"=w14:T14)
      n8 = Unbundle By Name(w12) -> ("Switch T/R"=w39:i16)
      n9 = case shown="\"5-CH Pulser New\", \"5-CH pulser w/ ann array\"" w15 {
        tunnel: w12 -> [w49 w51]
        tunnel: w14 -> [_ w52]
        tunnel: [w49 w50] -> w11
        frame "Single channel", Default {
        }
        frame "5-CH Pulser New", "5-CH pulser w/ ann array" {
          n10 = case shown="\"AlazarTech\"" w52 {
            tunnel: w51 -> [w53 w56]
            tunnel: [w53 w55] -> w50
            frame "Acqiris Digitizer", Default {
            }
            frame "AlazarTech" {
              n11 = Unbundle By Name(w56) -> ("Xmt/Rcv.RCV"=w58:bool[])
              n12 = Array Subset(array=w58, length=4) -> (w54:bool[])  [unwired: 1 in]
              n13 = Bundle By Name(cluster=w56, "Xmt/Rcv.RCV"=w54) -> (w55:T50)
              n14 = property on="RCV" class="Arr (strict)"("Value"=w54) -> ()  [unwired: 2 in, 2 out]
            }
          }
        }
      }
      n15 = property on="LeCroy Channels" class="Arr (strict)"("Value"=w16) -> ()  [unwired: 2 in, 2 out]
      n16 = global read "MotionGlobals.vi" "Filter Prams"() -> (w40:T17)
      n17 = property on="Transducer" class="DigNum (strict)"("Value"=w39) -> ()  [unwired: 2 in, 2 out]
      n18 = case shown="\"WCM Main\", Default" w48 {
        tunnel: [w167 w171 w174 w183] -> w46
        frame "WCM Main", Default {
          n19 = property on="TimeOut (s)" class="DigNum (strict)"("Value"=sgl 5.0 ("Value (Signaling)")) -> (error out=w167:errorcluster)  [unwired: 2 in, 1 out]
        }
        frame "Hawaii", "Stony Brook" {
          n20 = property on="Case Name" class="Str"("Value"="DEFAULT" ("Case Name")) -> (error out=w169:errorcluster)  [unwired: 2 in, 1 out]
          n21 = property on="Type of scan" class="Enum (strict)"(error in=w169, "Value"=ScanType2."Dual Transducer" ("Value (Signaling)")) -> (error out=w171:errorcluster)  [unwired: 1 in, 1 out]
        }
        frame "WCM Microscopy" {
          n22 = property on="Type of scan" class="Enum (strict)"("Value"=ScanType2."Acoustic Microscopy" ("Type of scan")) -> (error out=w176:errorcluster)  [unwired: 2 in, 1 out]
          n23 = property on="Microscopy Scan Mode" class="RadioBtnsControl (strict)"(error in=w176, "Value"=T7."Level X" ("Value (Signaling)")) -> (error out=w175:errorcluster)  [unwired: 1 in, 1 out]
          n24 = property on="New Sample" class="Bool (strict)"(error in=w175, "Value"=TRUE ("Value (Signaling)")) -> (error out=w174:errorcluster)  [unwired: 1 in, 1 out]
        }
        frame "NYU" {
          n25 = property on="distance?" class="Bool (strict)"("Value"=TRUE ("Value (Signaling)")) -> (error out=w180:errorcluster)  [unwired: 2 in, 1 out]
          n26 = property on="TimeOut (s)" class="DigNum (strict)"(error in=w180, "Value"=sgl 1.0 ("TimeOut (s)")) -> (error out=w179:errorcluster)  [unwired: 1 in, 1 out]
          n27 = property on="Type of scan" class="Enum (strict)"(error in=w179, "Value"=ScanType2."Real-Time Scan" ("Value (Signaling)")) -> (error out=w183:errorcluster)  [unwired: 1 in, 1 out]
        }
      }
      n28 = Unbundle By Name(w40) -> ("low cutoff"=w43:i32)
      n29 = Equal To 0?(x=w43) -> (x = 0?=w42:bool)
      n30 = case shown="False" w42 {
        tunnel: [w165 w166] -> w41
        tunnel: w40 -> [w165 _]
        frame False {
        }
        frame True {
          w166 = T17 {"low cutoff"=2, "order"=81, "high cutoff"=65} ("Filter Prams")
          n31 = global write "MotionGlobals.vi" "Filter Prams"(w166) -> ()
        }
      }
      n32 = property on="Debug Mode?" class="Bool (strict)"() -> ("Value"=w47:bool)  [unwired: 2 in, 2 out]
      n33 = property on="Filter Prams" class="Clust (strict)"("Value"=w41) -> ()  [unwired: 2 in, 2 out]
      n34 = property on="Erase data" class="Bool (strict)"(error in=w46, "Val(Sgnl)"=w21) -> ()  [unwired: 1 in, 2 out]
      n35 = case shown="False" w47 {
        tunnel: w48 -> [w82 _]
        tunnel: [w81 w164] -> w45
        tunnel: [w80 T45."Enabled" ("Disabled")] -> w44
        tunnel: [w79 w160] -> w38
        tunnel: [w78 w160] -> w37
        tunnel: [w77 w160] -> w36
        tunnel: [w76 T18."Visusalize" ("OPTIONS")] -> w35
        tunnel: [w75 w159] -> w18
        tunnel: [w74 w159] -> w34
        tunnel: [w73 TRUE ("Value (Signaling)")] -> w33
        tunnel: [w72 w153] -> w32
        tunnel: [w71 w160] -> w31
        tunnel: [w70 w153] -> w30
        tunnel: [w69 w153] -> w29
        tunnel: [w68 w159] -> w28
        tunnel: [w67 w159] -> w27
        tunnel: [w66 w159] -> w26
        tunnel: [w65 TRUE] -> w25
        tunnel: [w64 TRUE] -> w24
        tunnel: [w63 TRUE ("Value (Signaling)")] -> w23
        tunnel: [w62 TRUE ("Tabs Visible?")] -> w22
        tunnel: w21 -> [w61 _]
        tunnel: [w60 TRUE] -> w20
        tunnel: [w59 w153] -> w19
        frame False {
          n36 = case shown="\"Stony Brook\"" w82 {
            tunnel: [w89 w100 w113 w123 TRUE] -> w69
            tunnel: [FALSE ("Value (Signaling)") FALSE ("Value (Signaling)") TRUE ("Value (Signaling)") TRUE ("Value (Signaling)") FALSE ("Value (Signaling)")] -> w73
            tunnel: [w92 w103 w116 w127 w150] -> w81
            tunnel: [T45."Enabled" ("Disabled") T45."Enabled" ("Disabled") T45."Enabled" ("Disabled") T45."Disabled and Grayed Out" ("Disabled") T45."Enabled" ("Disabled")] -> w80
            tunnel: [w89 w93 w104 w123 FALSE] -> w79
            tunnel: [w89 w100 w104 w123 FALSE] -> w78
            tunnel: [w89 w93 w104 w123 TRUE] -> w77
            tunnel: [T18."Visusalize" ("OPTIONS") T18."Array Other" ("OPTIONS") T18."Other" ("OPTIONS") T18."Visusalize" ("OPTIONS") T18."Visusalize" ("OPTIONS")] -> w76
            tunnel: [w89 w100 TRUE ("Tabs Visible?") w123 TRUE ("Tabs Visible?")] -> w75
            tunnel: [w89 w100 TRUE ("Tabs Visible?") w123 TRUE ("Tabs Visible?")] -> w74
            tunnel: [w89 w100 w113 w123 TRUE] -> w72
            tunnel: [w89 w100 w113 w123 TRUE] -> w71
            tunnel: [w89 w100 w113 w123 w132] -> w70
            tunnel: [w89 w100 w105 w123 TRUE] -> w66
            tunnel: [w89 w100 w105 w123 TRUE] -> w68
            tunnel: [w89 w100 w105 w123 TRUE] -> w67
            tunnel: [w83 TRUE FALSE FALSE TRUE] -> w65
            tunnel: [TRUE TRUE FALSE TRUE TRUE] -> w64
            tunnel: [TRUE ("Value (Signaling)") TRUE ("Value (Signaling)") TRUE ("Value (Signaling)") FALSE ("Value (Signaling)") TRUE ("Value (Signaling)")] -> w63
            tunnel: [TRUE ("Tabs Visible?") TRUE ("Tabs Visible?") TRUE ("Tabs Visible?") FALSE ("Tabs Visible?") FALSE ("Tabs Visible?")] -> w62
            tunnel: w61 -> [w84 w94 _ w119 w131]
            tunnel: [_ _ _ TRUE TRUE] -> w60
            tunnel: [w83 w93 w104 TRUE w132] -> w59
            frame "WCM Main", Default {
              w83 = TRUE
              w92 = u16 4 items=["Mean from lines", "Mean just lines", "Poly Mean", "No mean", "Filter"] ("Type of Mean")
              w89 = TRUE
              n37 = property on="SetDig" class="Bool (strict)"("Val(Sgnl)"=w84) -> ()  [unwired: 2 in, 2 out]
            }
            frame "NYU" {
              w93 = FALSE
              w103 = u16 4 items=["Mean from lines", "Mean just lines", "Poly Mean", "No mean", "Filter"] ("Type of Mean")
              w100 = TRUE
              n38 = property on="SetDig" class="Bool (strict)"("Val(Sgnl)"=w94) -> ()  [unwired: 2 in, 2 out]
            }
            frame "WCM Microscopy" {
              w105 = FALSE
              w104 = FALSE
              w116 = u16 3 items=["Mean from lines", "Mean just lines", "Poly Mean", "No mean", "Filter"] ("Type of Mean")
              w113 = TRUE
            }
            frame "Stony Brook" {
              w127 = u16 3 items=["Mean from lines", "Mean just lines", "Poly Mean", "No mean", "Filter"] ("Type of Mean")
              w123 = FALSE
              n39 = property on="Skip Real\nTime Setup" class="Bool (strict)"() -> ("Value"=w129:bool)  [unwired: 2 in, 2 out]
              n40 = case shown="True" w129 {
                tunnel: w119 -> [w130 _]
                frame False {
                  n41 = property on="start scan" class="Bool (strict)"("Val(Sgnl)"=w130) -> ()  [unwired: 2 in, 2 out]
                }
                frame True {
                }
              }
            }
            frame "Hawaii" {
              w132 = FALSE
              w150 = u16 3 items=["Mean from lines", "Mean just lines", "Poly Mean", "No mean", "Filter"] ("Type of Mean")
              n42 = property on="SetDig" class="Bool (strict)"("Val(Sgnl)"=w131) -> ()  [unwired: 2 in, 2 out]
            }
          }
        }
        frame True {
          w159 = TRUE
          w160 = TRUE
          w164 = u16 3 items=["Mean from lines", "Mean just lines", "Poly Mean", "No mean", "Filter"] ("Type of Mean")
          w153 = TRUE
        }
      }
      n43 = property on="Transpose" class="Bool (strict)"("Value"=w20) -> ()  [unwired: 2 in, 2 out]
      n44 = property on="OPTIONS" class="TabCtl (strict)"("Value"=w35, "Page Labels Display Visible?"=w18, "Visible"=w34) -> ()  [unwired: 2 in, 2 out]
      n45 = property on="Load Scan Settings" class="Bool"("Visible"=w22) -> ()  [unwired: 2 in, 2 out]
      n46 = property on="Save Scan Settings" class="Bool"("Visible"=w22) -> ()  [unwired: 2 in, 2 out]
      n47 = property on="Transducer" class="DigNum (strict)"("Visible"=w24) -> ()  [unwired: 2 in, 2 out]
      n48 = property on="Trans Geometry (mm)" class="Clust (strict)"("Visible"=w37) -> ()  [unwired: 2 in, 2 out]
      n49 = property on="Synth Foc?" class="Bool (strict)"("Visible"=w37) -> ()  [unwired: 2 in, 2 out]
      n50 = property on="Focal Zones" class="DigNum (strict)"("Visible"=w37) -> ()  [unwired: 2 in, 2 out]
      n51 = property on="Display mode" class="Enum (strict)"("Visible"=w32) -> ()  [unwired: 2 in, 2 out]
      n52 = property on="Show Thumbs" class="Bool"("Visible"=w36) -> ()  [unwired: 2 in, 2 out]
      n53 = property on="Take Webcam pic" class="Bool (strict)"("Visible"=w19) -> ()  [unwired: 2 in, 2 out]
      n54 = property on="CH2?" class="Bool (strict)"("Visible"=w38) -> ()  [unwired: 2 in, 2 out]
      n55 = property on="Trig (Hz)" class="DigNum (strict)"("Visible"=w38) -> ()  [unwired: 2 in, 2 out]
      n56 = property on="RT V" class="DigNum (strict)"("Visible"=w38) -> ()  [unwired: 2 in, 2 out]
      n57 = property on="MIP Thresh" class="DigNum (strict)"("Visible"=w38) -> ()  [unwired: 2 in, 2 out]
      n58 = property on="C MIP" class="Bool (strict)"("Visible"=w38) -> ()  [unwired: 2 in, 2 out]
      n59 = property on="Compress" class="Bool (strict)"("Visible"=w38) -> ()  [unwired: 2 in, 2 out]
      n60 = property on="distance?" class="Bool (strict)"("Value"=w33, "Visible"=w23) -> ()  [unwired: 2 in, 2 out]
      n61 = property on="Avg Num" class="DigNum (strict)"("Visible"=w31) -> ()  [unwired: 2 in, 2 out]
      n62 = property on="Fix Z Delay?" class="Bool (strict)"("Visible"=w31) -> ()  [unwired: 2 in, 2 out]
      n63 = property on="TimeOut (s)" class="DigNum (strict)"("Visible"=w31) -> ()  [unwired: 2 in, 2 out]
      n64 = property on="Set Pulser" class="Bool"("Visible"=w29) -> ()  [unwired: 2 in, 2 out]
      n65 = property on="Man Cont" class="Bool"("Visible"=w29) -> ()  [unwired: 2 in, 2 out]
      n66 = property on="Digitzer Error Message" class="Str"("Visible"=w30) -> ()  [unwired: 2 in, 2 out]
      n67 = property on="Type of Mean" class="Enum (strict)"("Visible"=w25, "Value"=w45) -> ()  [unwired: 2 in, 2 out]
      n68 = property on="Filter Prams" class="Clust (strict)"("Visible"=w28) -> ()  [unwired: 2 in, 2 out]
      n69 = property on="scan pair" class="Enum (strict)"("Visible"=w26) -> ()  [unwired: 2 in, 2 out]
      n70 = property on="One Way Scan" class="Bool (strict)"("Visible"=w26) -> ()  [unwired: 2 in, 2 out]
      n71 = property on="Overshoot" class="DigNum (strict)"("Visible"=w27) -> ()  [unwired: 2 in, 2 out]
      n72 = property on="lines per plane" class="DigNum (strict)"("DisabledEnum"=w44) -> ()  [unwired: 2 in, 2 out]
      n73 = property on="Distance between\nscan lines (um)" class="DigNum (strict)"("DisabledEnum"=w44) -> ()  [unwired: 2 in, 2 out]
      n74 = property on="number of planes" class="DigNum (strict)"("DisabledEnum"=w44) -> ()  [unwired: 2 in, 2 out]
      n75 = property on="Distance between\nplanes (um)" class="DigNum (strict)"("DisabledEnum"=w44) -> ()  [unwired: 2 in, 2 out]
      n76 = property on="Length of\none plane (mm)" class="DigNum (strict)"("DisabledEnum"=w44) -> ()  [unwired: 2 in, 2 out]
      n77 = property on="Length of\nall planes (mm)" class="DigNum (strict)"("DisabledEnum"=w44) -> ()  [unwired: 2 in, 2 out]
      n78 = property on="Case Name" class="Str"("DisabledEnum"=w44) -> ()  [unwired: 2 in, 2 out]
      n79 = property on="Type of scan" class="Enum (strict)"("DisabledEnum"=w44) -> ()  [unwired: 2 in, 2 out]
      n80 = property on="Skip Real Time Setup" class="Bool (strict)"("Value"=w17) -> ()  [unwired: 2 in, 2 out]
      n81 = property on="Attenuation Scan" class="Bool (strict)"("Value"=w17) -> ()  [unwired: 2 in, 2 out]
    }
    frame #1 {
      n82 = while {
        tunnel: w195 -> [w214]
        shift-right: [w212] -> w189
        shift-left: w194 -> [w213]
        shift-right: [w209] -> w188
        shift-left: w193 -> [w210]
        tunnel: w192 -> [w205]
        shift-right: [w204] -> w190
        shift-left: w191 -> [w207]
        shift-right: [w201] -> w187
        shift-left: w185 -> [w200]
        tunnel: w186 -> [w198]
        i -> [w208]
        stop <- w216 stop-if-true
        n83 = global read "MotionGlobals.vi" "33250(T)/33120(F)"() -> (w218:bool)
        n84 = Unbundle By Name(w200) -> ("Switch T/R"=w199:i16)
        n85 = global read "SwitchGlobals.vi" "Switch Unit"() -> (w203:T51)
        n86 = global write "MotionGlobals.vi" "Debug Mode?"("Debug Mode?") -> ()
        n87 = global read "MotionGlobals.vi" "EKG Gate?"() -> (w206:T52)
        n88 = Unbundle By Name(w210) -> ("Motion Bd ID"=w211:u8)
        n89 = local write "Transducer"(w199) -> ()
        n90 = case shown="\"Therapy With Scan\", Default" "Type of scan" {
          tunnel: [TRUE FALSE] -> w217
          frame "Therapy With Scan", Default {
          }
          frame "2-D B Scan", "2-D B Scan With Therapy Burst", "2-D B-Scan PRF", "Contrast Agents", "Acoustic Microscopy", "Hydrophone Scanning" {
          }
        }
        n91 = global read "PulserGlobals.vi" "Pulser"() -> (w202:T53)
        n92 = global write "MotionGlobals.vi" "Type of scan"("Type of scan") -> ()
        n93 = Equal To 0?(x=w208) -> (x = 0?=w196:bool)
        n94 = stacked-sequence {
          seq-local: [_ _ w438 _ _ _] -> [_ _ _ _ w514 w2638]
          seq-local: [_ w259 _ _ _ _] -> [_ _ _ _ w515 _]
          seq-local: [_ w260 _ _ _ _] -> [_ _ _ _ w516 _]
          seq-local: [_ _ w439 _ _ _] -> [_ _ _ _ w513 w2637]
          tunnel: "Type of scan" -> [_ w258 _ _ w512 _]
          tunnel: w218 -> [_ _ w436 _ _ w2633]
          tunnel: w205 -> [_ w233 w435 w466 w497 w2634]
          tunnel: w217 -> [_ _ _ _ w511 _]
          tunnel: w211 -> [_ _ _ _ w510 _]
          tunnel: [_ _ _ _ w509 _] -> w216
          tunnel: w214 -> [_ _ _ _ w508 _]
          tunnel: w213 -> [_ w230 _ w469 w492 _]
          tunnel: [_ _ _ _ w507 _] -> w212
          tunnel: w210 -> [_ _ w434 w480 w499 _]
          tunnel: [_ _ _ _ w506 _] -> w209
          tunnel: w196 -> [_ _ _ w464 _ _]
          tunnel: w203 -> [w221 _ _ _ w503 _]
          tunnel: w207 -> [_ w237 _ _ w502 _]
          tunnel: w202 -> [_ _ _ _ w501 _]
          tunnel: w206 -> [_ _ _ _ w500 _]
          tunnel: [_ _ _ _ w498 _] -> w204
          tunnel: w200 -> [_ _ _ _ w496 _]
          tunnel: [_ _ _ _ w495 _] -> w201
          tunnel: w198 -> [_ _ _ _ w494 _]
          tunnel: "Debug Mode?" -> [_ _ _ _ _ _]
          frame #0 {
            w222 = 1.0
            n95 = case shown="\"No Switch\", Default" w221 {
              tunnel: [_ 8 _ 5.0 2] -> w223
              frame "Cytex" {
              }
              frame "Pickering" {
              }
              frame "NI Switch" {
              }
              frame "No Switch", Default {
              }
              frame "Riverside USB" {
              }
            }
            n96 = property on="Transducer" class="DigNum (strict)"("Maximum"=w223, "Minimum"=w222, "Increment"=w222) -> ()  [unwired: 2 in, 2 out]
          }
          frame #1 {
            # "set up which controls are visible on front panel"
            # "Ascan ?"
            # "Therapy?"
            # "Make some initial settings"
            n97 = Unbundle By Name(w230) -> ("Main Digitizer"=w229:T14)
            n98 = Unbundle By Name(w237) -> ("XDCR Offset"=w235:dbl[])
            n99 = Equal?(x=Digitizer."LeCroy", y=w229) -> (x = y?=w231:bool)
            n100 = property on="Pulse" class="Bool (strict)"("Visible"=w231) -> ()  [unwired: 2 in, 2 out]
            n101 = Array Max & Min(array=w235) -> (max value=w236:dbl)  [unwired: 3 out]
            n102 = Search 1D Array(1D array=w235, element=w236) -> (index of element=w234:i32)  [unwired: 1 in]
            n103 = case shown="\"WCM Main\"" w233 {
              tunnel: [i32[] [-1] ("Disabled Items []") i32[] [0, 2, 4, 6, 7, 8, 9, 11, 14] ("Disabled Items []") i32[] [-1] ("Disabled Items []") i32[] [0, 2, 4, 6, 7, 8, 9, 11, 12, 13, 14] ("Disabled Items []") i32[] [-1] ("Disabled Items []") i32[] [0, 2, 4, 6, 7, 11, 12] ("Disabled Items []") i32[] [0, 2, 4, 6, 7, 11, 12] ("Disabled Items []") i32[] [0, 2, 4, 6, 7, 8, 9, 11, 12] ("Disabled Items []") i32[] [0, 2, 4, 6, 7, 8, 9, 11, 12, 13] ("Disabled Items []")] -> w242
              tunnel: [_ _ _ _ _ _ _ _ TRUE ("Visible")] -> w241
              frame "WCM Main" {
              }
              frame "Hawaii" {
                # "HI"
              }
              frame "Columbia MM3000", Default {
              }
              frame "NYU" {
              }
              frame "RRI 2" {
              }
              frame "UHI Allen" {
                # "John's HI ESP300 system."
              }
              frame "CUMC RT" {
                # "John's HI ESP300 system."
              }
              frame "Stony Brook" {
              }
              frame "Chiba" {
                # "Chiba system."
              }
            }
            n104 = case shown="\"1-D B-Scan PRF\"" w258 {
              tunnel: [FALSE FALSE TRUE FALSE TRUE FALSE FALSE FALSE TRUE FALSE FALSE FALSE FALSE TRUE FALSE] -> w259
              tunnel: [TRUE TRUE TRUE FALSE FALSE FALSE FALSE FALSE FALSE FALSE TRUE TRUE FALSE FALSE FALSE] -> w260
              tunnel: [w272 w281 w290 w301 w312 w321 w333 w348 w357 w368 w379 w390 w403 FALSE ("Write Attribute") w425] -> w255
              tunnel: [w272 w281 w290 w299 w310 w321 FALSE ("Write Attribute") w348 w357 w366 w377 w390 w400 w411 w423] -> w239
              tunnel: [w275 w284 w293 w304 w315 w324 w336 w351 w360 w370 FALSE ("Write Attribute") FALSE ("Write Attribute") w406 w417 w428] -> w252
              tunnel: [TRUE FALSE FALSE FALSE FALSE FALSE FALSE FALSE FALSE FALSE FALSE FALSE FALSE FALSE FALSE] -> w257
              tunnel: [FALSE ("Write Attribute") TRUE ("Write Attribute") TRUE ("Write Attribute") TRUE ("Write Attribute") TRUE ("Write Attribute") TRUE ("Write Attribute") TRUE ("Write Attribute") TRUE ("Write Attribute") TRUE ("Write Attribute") FALSE ("Write Attribute") TRUE ("Write Attribute") TRUE ("Write Attribute") TRUE ("Write Attribute") TRUE ("Write Attribute") TRUE ("Write Attribute")] -> w256
              tunnel: [FALSE ("Write Attribute") FALSE ("Write Attribute") FALSE ("Write Attribute") FALSE ("Write Attribute") FALSE ("Write Attribute") FALSE ("Write Attribute") FALSE ("Write Attribute") FALSE ("Write Attribute") FALSE ("Write Attribute") TRUE ("Write Attribute") FALSE ("Write Attribute") FALSE ("Write Attribute") FALSE ("Write Attribute") FALSE ("Write Attribute") FALSE ("Write Attribute")] -> w254
              tunnel: 1 -> [_ _ _ w303 w314 _ _ _ _ _ w381 _ w405 w416 w427]
              tunnel: [w275 w284 w293 w304 w315 w324 w336 w351 w360 w370 TRUE ("Write Attribute") TRUE ("Write Attribute") w406 w417 w428] -> w249
              tunnel: [w273 w282 w291 w300 w311 w322 FALSE ("Write Attribute") w349 w358 w367 TRUE ("Write Attribute") TRUE ("Write Attribute") w401 w412 w424] -> w251
              tunnel: [FALSE ("Write Attribute") FALSE ("Write Attribute") FALSE ("Write Attribute") FALSE ("Write Attribute") FALSE ("Write Attribute") FALSE ("Write Attribute") FALSE ("Write Attribute") FALSE ("Write Attribute") FALSE ("Write Attribute") FALSE ("Write Attribute") FALSE ("Write Attribute") FALSE ("Write Attribute") FALSE ("Write Attribute") TRUE ("Write Attribute") FALSE ("Write Attribute")] -> w243
              tunnel: [w272 w281 w290 w301 w312 w321 w333 w348 w357 w368 w379 w390 w403 FALSE ("Write Attribute") w425] -> w250
              tunnel: [_ _ _ _ _ _ _ w343 _ _ _ _ _ _ _] -> w232
              tunnel: [w273 w282 w291 w300 w311 w322 TRUE w349 w358 w367 FALSE ("Write Attribute") FALSE ("Write Attribute") w401 w412 w424] -> w227
              tunnel: [w272 w281 w290 w299 w310 w321 TRUE ("Write Attribute") w348 w357 w366 w377 w390 w400 w411 w423] -> w238
              tunnel: w234 -> [_ _ _ _ _ _ _ w347 _ _ _ _ _ _ _]
              tunnel: w233 -> [_ _ _ _ _ _ _ w342 _ _ _ _ _ _ _]
              frame "Therapy With Scan" {
                w273 = FALSE ("Write Attribute")
                w272 = FALSE ("Write Attribute")
                w275 = TRUE ("Write Attribute")
                # "Therapy w/scan"
                # "Panel for Ascan"
              }
              frame "M scan", Default {
                w282 = FALSE ("Write Attribute")
                w281 = FALSE ("Write Attribute")
                w284 = TRUE ("Write Attribute")
                # "M Scan"
                # "Panel for Ascan"
              }
              frame "M Scan With Therapy Burst" {
                w291 = FALSE ("Write Attribute")
                w290 = FALSE ("Write Attribute")
                w293 = TRUE ("Write Attribute")
                # "MScan with Ther"
                # "A scan with therapy"
              }
              frame "1-D B Scan" {
                w300 = FALSE ("Write Attribute")
                w301 = FALSE ("Write Attribute")
                w299 = TRUE ("Write Attribute")
                w304 = FALSE ("Write Attribute")
                # "1-D scan"
                # "b scan 1 -D"
                n105 = local write "number of planes"(w303) -> ()
              }
              frame "1-D B Scan With Therapy Burst" {
                w311 = FALSE ("Write Attribute")
                w312 = FALSE ("Write Attribute")
                w310 = TRUE ("Write Attribute")
                w315 = FALSE ("Write Attribute")
                # "1 D scan w/ ther"
                # "B scan 1-D w/ therapy"
                n106 = local write "number of planes"(w314) -> ()
              }
              frame "2-D B Scan", "Hydrophone Scanning" {
                w322 = FALSE ("Write Attribute")
                w321 = TRUE ("Write Attribute")
                w324 = FALSE ("Write Attribute")
                # "2-D scan"
                # "b scan 2-D"
              }
              frame "Acoustic Microscopy" {
                w333 = TRUE ("Write Attribute")
                w336 = FALSE ("Write Attribute")
                # "2-D scan"
                # "b scan 2-D"
              }
              frame "Dual Transducer" {
                w349 = FALSE ("Write Attribute")
                w348 = TRUE ("Write Attribute")
                w351 = FALSE ("Write Attribute")
                # "2-D scan"
                # "b scan 2-D"
                n107 = case shown="0, Default" w347 {
                  frame 0, Default {
                  }
                  frame 1 {
                  }
                }
                n108 = Equal?(x=w342, y=location."Hawaii") -> (x = y?=w345:bool)
                n109 = And(x=TRUE ("Write Attribute"), y=w345) -> (x .and. y?=w343:bool)
              }
              frame "2-D B Scan With Therapy Burst" {
                w358 = FALSE ("Write Attribute")
                w357 = TRUE ("Write Attribute")
                w360 = FALSE ("Write Attribute")
                # "2-D scan w/ ther"
                # "b scan 2-D w/therapy"
              }
              frame "Rotational Scan" {
                w367 = FALSE ("Write Attribute")
                w366 = FALSE ("Write Attribute")
                w368 = TRUE ("Write Attribute")
                w370 = FALSE ("Write Attribute")
                # "Rot scan"
                # "b scan 2-D w/therapy"
              }
              frame "1-D B-Scan PRF" {
                w377 = TRUE ("Write Attribute")
                w379 = FALSE ("Write Attribute")
                # "1-d Swept"
                # "b scan 2-D w/therapy"
                n110 = local write "number of planes"(w381) -> ()
              }
              frame "2-D B-Scan PRF" {
                w390 = TRUE ("Write Attribute")
                # "2-D  swept"
                # "b scan 2-D"
              }
              frame "Real-Time Scan" {
                w401 = FALSE ("Write Attribute")
                w403 = FALSE ("Write Attribute")
                w400 = TRUE ("Write Attribute")
                w406 = FALSE ("Write Attribute")
                # "real-time"
                # "b scan 1 -D"
                n111 = local write "number of planes"(w405) -> ()
              }
              frame "Contrast Agents" {
                w412 = FALSE ("Write Attribute")
                w411 = FALSE ("Write Attribute")
                w417 = TRUE ("Write Attribute")
                # "contrast"
                # "b scan 1 -D"
                n112 = local write "number of planes"(w416) -> ()
              }
              frame "1-D w/ Real-Time Set Up" {
                w424 = FALSE ("Write Attribute")
                w425 = FALSE ("Write Attribute")
                w423 = TRUE ("Write Attribute")
                w428 = FALSE ("Write Attribute")
                # "1-D scan +realtime"
                # "b scan 1 -D"
                n113 = local write "number of planes"(w427) -> ()
              }
            }
            n114 = global read "MotionGlobals.vi" "EKG Gate?"() -> (w247:T52)
            n115 = Not(x=w241) -> (.not. x?=w240:bool)
            n116 = property on="Microscopy Scan Mode" class="RadioBtnsControl (strict)"("Visible"=w227) -> ()  [unwired: 2 in, 2 out]
            n117 = property on="Auto Vz Depth" class="DigNum (strict)"("Visible"=w227) -> ()  [unwired: 2 in, 2 out]
            n118 = property on="HF XDCR" class="Enum (strict)"("Visible"=w227) -> ()  [unwired: 2 in, 2 out]
            n119 = property on="Auto Vz?" class="Bool (strict)"("Visible"=w227, "Val(Sgnl)"=w227) -> ()  [unwired: 2 in, 2 out]
            n120 = property on="RT fps" class="DigNum (strict)"("Visible"=w240) -> ()  [unwired: 2 in, 2 out]
            n121 = property on="Resp Divide" class="DigNum (strict)"("Visible"=w240) -> ()  [unwired: 2 in, 2 out]
            n122 = property on="Type of scan" class="Enum (strict)"("Disabled Items []"=w242) -> ()  [unwired: 2 in, 2 out]
            n123 = Not Equal To 0?(x=w247) -> (x != 0?=w246:bool)
            n124 = property on="Next Scan" class="Bool (strict)"("Visible"=w227) -> ()  [unwired: 2 in, 2 out]
            n125 = property on="New Sample" class="Bool (strict)"("Visible"=w227) -> ()  [unwired: 2 in, 2 out]
            n126 = Not(x=w246) -> (.not. x?=w245:bool)
            n127 = Or(x=w246, y=w249) -> (x .or. y?=w248:bool)
            n128 = And(x=w245, y=w238) -> (x .and. y?=w244:bool)
            n129 = property on="Estimated Line spacing" class="DigNum (strict)"("Visible"=w251) -> ()  [unwired: 2 in, 2 out]
            n130 = property on="prf (kHz)" class="DigNum (strict)"("Visible"=w248) -> ()  [unwired: 2 in, 2 out]
            n131 = property on="lines per plane" class="DigNum (strict)"("Visible"=w256) -> ()  [unwired: 2 in, 2 out]
            n132 = property on="Attenuation Scan" class="Bool (strict)"("Visible"=w232) -> ()  [unwired: 2 in, 2 out]
            n133 = property on="number of planes" class="DigNum (strict)"("Visible"=w250) -> ()  [unwired: 2 in, 2 out]
            n134 = property on="Skip Real Time Setup" class="Bool (strict)"("Visible"=w232) -> ()  [unwired: 2 in, 2 out]
            n135 = property on="Time between\n samples (ms)" class="DigNum (strict)"("Visible"=w252) -> ()  [unwired: 2 in, 2 out]
            n136 = property on="Therapy Parameters" class="Clust (strict)"("Visible"=w257) -> ()  [unwired: 2 in, 2 out]
            n137 = property on="Rot lines per plane" class="Ring (strict)"("Visible"=w254) -> ()  [unwired: 2 in, 2 out]
            n138 = property on="Sector Angle" class="Slide (strict)"("Visible"=w254) -> ()  [unwired: 2 in, 2 out]
            n139 = property on="Distance between\nplanes (um)" class="DigNum (strict)"("Visible"=w255) -> ()  [unwired: 2 in, 2 out]
            n140 = property on="Length of\none plane (mm)" class="DigNum (strict)"("Visible"=w244) -> ()  [unwired: 2 in, 2 out]
            n141 = property on="Drive Voltages" class="Arr (strict)"("Visible"=w243) -> ()  [unwired: 2 in, 2 out]
            n142 = property on="CA Threshold" class="DigNum (strict)"("Visible"=w243) -> ()  [unwired: 2 in, 2 out]
            n143 = property on="Burst Ct" class="Arr (strict)"("Visible"=w243) -> ()  [unwired: 2 in, 2 out]
            n144 = property on="Length of\nall planes (mm)" class="DigNum (strict)"("Visible"=w255) -> ()  [unwired: 2 in, 2 out]
            n145 = property on="Distance between\nscan lines (um)" class="DigNum (strict)"("Visible"=w244) -> ()  [unwired: 2 in, 2 out]
            n146 = case shown="\"WCM Main\", Default" w233 {
              tunnel: w239 -> [w261 _]
              frame "WCM Main", Default {
                n147 = property on="One Way Scan" class="Bool (strict)"("Visible"=w261) -> ()  [unwired: 2 in, 2 out]
                n148 = property on="Overshoot" class="DigNum (strict)"("Visible"=w261) -> ()  [unwired: 2 in, 2 out]
                n149 = property on="scan pair" class="Enum (strict)"("Visible"=w261) -> ()  [unwired: 2 in, 2 out]
              }
              frame "Stony Brook" {
              }
            }
          }
          frame #2 {
            n150 = global read "MotionGlobals.vi" "No GPIB?"() -> (w437:bool)
            n151 = case shown="\"Hawaii\", \"SERI GP\"" w435 {
              tunnel: w434 -> [_ w441]
              frame "WCM Main", Default {
              }
              frame "Hawaii", "SERI GP" {
                n152 = Unbundle By Name(w441) -> ("Motion System"=w440:T11)
                n153 = case shown="\"Galil\"" w440 {
                  tunnel: w441 -> [_ w443 w446]
                  frame "MM3000", Default {
                  }
                  frame "NI 735x" {
                    # "Load PRF program (3)"
                    n154 = Unbundle By Name(w443) -> ("Motion Bd ID"=w442:u8)
                    n155 = call "BrkPtPRF.vi"("Bd ID in"=w442) -> ()  [unwired: 2 in, 2 out]
                  }
                  frame "Galil" {
                    n156 = Unbundle By Name(w446) -> ("GL Ref Out"=w445:refnum<k7>)
                    n157 = call "GL_BrkPtPRF.vi"("GL Ref Out"=w445, "Program Name"="#PRF") -> ()  [unwired: 4 in, 2 out]
                  }
                }
              }
            }
            n158 = case shown="False" w437 {
              tunnel: [w455 "VISA session 2"] -> w439
              tunnel: [w450 "VISA session 2"] -> w438
              tunnel: w436 -> [w453 _]
              tunnel: w435 -> [w452 _]
              frame False {
                # "Set up other HP33120A for \nburst mode."
                n159 = case shown="True" w453 {
                  tunnel: ["TRIG:SOUR EXT;:SOUR:BM:STAT ON" ""] -> w454
                  frame False {
                  }
                  frame True {
                    (unwired) "BURS:STAT ON;:TRIG:SOUR EXT;:BURS:MODE GAT;:OUTP ON"
                  }
                }
                n160 = case shown="\"WCM Main\", Default" w452 {
                  tunnel: ["GPIB::11" ("instrument descripter") "GPIB0::3" ("instrument descripter")] -> w451
                  frame "WCM Main", Default {
                  }
                  frame "Columbia MM3000" {
                  }
                }
                n161 = VISA Open(VISA resource name="GPIB::10") -> (VISA resource name=w448:refnum<visa-resource-name>, error out=w447:errorcluster)  [unwired: 4 in]
                n162 = VISA Open(VISA resource name=w451) -> (VISA resource name=w450:refnum<visa-resource-name>)  [unwired: 4 in, 1 out]
                n163 = VISA Write(VISA resource name=w448, write buffer=w454, error in (no error)=w447) -> (VISA resource name out=w455:refnum<visa-resource-name>)  [unwired: 2 out]
              }
              frame True {
              }
            }
          }
          frame #3 {
            n164 = Unbundle By Name(w480) -> ("scan pair"=w472:T12, "Distance between\nscan lines (um)"=w482:sgl, "Distance between\nscan planes (um)"=w481:sgl)
            n165 = Unbundle By Name(w469) -> ("Dig Config"=w468:T15)
            n166 = Unbundle By Name(w480) -> ("number of scan planes"=w486:i32, "overshoot cts"=w485:i32, "One Way Scan"=w484:bool, "Add Axis"=w478:bool, "Reverse One Way Scan"=w476:bool)
            n167 = Unbundle By Name(w469) -> ("lines per plane"=w488:i32, "Avg Num"=w487:i32)
            n168 = global read "MotionGlobals.vi" "c mm/mics"() -> (w463:sgl)
            n169 = local read "Resp Divide"() -> (w461:i32)
            n170 = local read "Bulk Acq"() -> (w491:bool)
            n171 = local read "prf (kHz)"() -> (w483:dbl)
            n172 = Equal?(x=w468, y=4) -> (x = y?=w474:bool)
            n173 = Equal?(x=w466, y=location."WCM Main") -> (x = y?=w473:bool)
            n174 = Unbundle By Name(w480) -> ("RT fps"=w479:sgl)
            n175 = Compound Arithmetic op=AND(w474, w473, w464) -> (w475:bool)
            n176 = global write "MotionGlobals.vi" "Breath Divide"(w461) -> ()
            n177 = global write "MotionGlobals.vi" "DAQ Range"("DAQ Range") -> ()
            n178 = Select(t=ScanAxis."w-(x) scan", s=w475, f=w472) -> (s? t:f=w471:T12)
            n179 = property on="c mm/mics" class="DigNum (strict)"("Value"=w463) -> ()  [unwired: 2 in, 2 out]
            n180 = property on="Distance between\nscan lines (um)" class="DigNum (strict)"("Value"=w482) -> ()  [unwired: 2 in, 2 out]
            n181 = property on="Distance between\nplanes (um)" class="DigNum (strict)"("Value"=w481) -> ()  [unwired: 2 in, 2 out]
            n182 = property on="number of planes" class="DigNum (strict)"("Val(Sgnl)"=w486) -> ()  [unwired: 2 in, 2 out]
            n183 = property on="Overshoot" class="DigNum (strict)"("Val(Sgnl)"=w485) -> ()  [unwired: 2 in, 2 out]
            n184 = property on="One Way Scan" class="Bool (strict)"("Val(Sgnl)"=w484) -> ()  [unwired: 2 in, 2 out]
            n185 = property on="Add Axis" class="Bool (strict)"("Val(Sgnl)"=w478) -> ()  [unwired: 2 in, 2 out]
            n186 = property on="Reverse One \nWay Scan" class="Bool (strict)"("Value"=w476) -> ()  [unwired: 2 in, 2 out]
            n187 = property on="lines per plane" class="DigNum (strict)"("Val(Sgnl)"=w488) -> ()  [unwired: 2 in, 2 out]
            n188 = property on="RT fps" class="DigNum (strict)"("Value"=w479) -> ()  [unwired: 2 in, 2 out]
            n189 = property on="scan pair" class="Enum (strict)"("Value"=w471) -> ()  [unwired: 2 in, 2 out]
            n190 = property on="Avg Num" class="DigNum (strict)"("Value"=w487) -> ()  [unwired: 2 in, 2 out]
            n191 = property on="Bulk Acq" class="Bool (strict)"("Value"=w491) -> ()  [unwired: 2 in, 2 out]
            n192 = property on="Multi Trig" class="Bool (strict)"("Value"="Multi Trig") -> ()  [unwired: 2 in, 2 out]
            n193 = property on="DAQ Range" class="Clust (strict)"("Value"="DAQ Range") -> ()  [unwired: 2 in, 2 out]
            n194 = property on="Resp Divide" class="DigNum (strict)"("Value"=w461) -> ()  [unwired: 2 in, 2 out]
            n195 = property on="prf (kHz)" class="DigNum (strict)"("Value"=w483) -> ()  [unwired: 2 in, 2 out]
            n196 = property on="USB Gate\nPer Sample" class="Bool (strict)"("Value"="USB Gate\nPer Sample") -> ()  [unwired: 2 in, 2 out]
            n197 = local read "CTR PRF?"() -> (w489:bool)
            n198 = global write "MotionGlobals.vi" "CTR PRF?"(w489) -> ()
          }
          frame #4 {
            # "labview lecroy automation commands"
            n199 = case shown="True" FALSE {
              frame False {
              }
              frame True {
                w517 = 0.0 ("Value (Signaling)")
                n200 = property on="Length of\none plane (mm)" class="DigNum (strict)"("Val(Sgnl)"=w517) -> (error out=w519:errorcluster)  [unwired: 2 in, 1 out]
                n201 = property on="Length of\nall planes (mm)" class="DigNum (strict)"(error in=w519, "Val(Sgnl)"=w517) -> (error out=w520:errorcluster)  [unwired: 1 in, 1 out]
                n202 = property on="Microscopy \nScan Mode" class="RadioBtnsControl (strict)"(error in=w520, "Val(Sgnl)"=T7."Detailed Scan" ("Value (Signaling)")) -> ()  [unwired: 1 in, 2 out]
              }
            }
            n203 = Unbundle By Name(w492) -> ("Dig Config"=w505:T15)
            n204 = case shown="\"Single channel\", Default" w505 {
              tunnel: [TRUE _] -> w504
              frame "Single channel", Default {
              }
              frame "5-CH Pulser New".."5-pass style ann array" {
              }
            }
            n205 = while {
              tunnel: w511 -> [w548]
              shift-left: _ -> [w552]
              shift-right: [w545] -> _
              shift-left: _ -> [w522]
              shift-right: [w551] -> _
              tunnel: w513 -> [w553]
              tunnel: w514 -> [w540]
              tunnel: w512 -> [w541]
              tunnel: w515 -> [w554]
              tunnel: w516 -> [w555]
              tunnel: w504 -> [w546]
              tunnel: w510 -> [w542]
              tunnel: [w527] -> w509
              tunnel: w508 -> [w528]
              shift-right: [w537] -> w507
              shift-left: w492 -> [w538]
              shift-right: [w535] -> w506
              shift-left: w499 -> [w536]
              tunnel: w503 -> [w534]
              tunnel: w501 -> [w532]
              tunnel: w500 -> [w531]
              shift-right: [w530] -> w498
              shift-left: w502 -> [w533]
              tunnel: w497 -> [w529]
              shift-right: [w526] -> w495
              shift-left: w496 -> [w525]
              tunnel: w494 -> [w523]
              stop <- w539 stop-if-true
              # "Current case\nviewed"
              # "Data with\nscan info"
              # "Case names"
              n206 = Unbundle By Name(w525) -> ("Synth Foc?"=w524:bool)
              n207 = Or(x=w524, y=w546) -> (x .or. y?=w547:bool)
              n208 = And(x=w548, y=w547) -> (x .and. y?=w549:bool)
              n209 = event shown="[34] \"Bulk Acq\", \"Full Array Scan?\", \"Synth Foc?\", \"GPU?\", \"Save TIFF?\", \"DownFactor\", \"RCV 1CH\": Value Change" {
                selector: _ -> [_ _ _ _ _ _ _ _ _ _ _ _ _ _ _ _ _ _ _ _ _ _ _ _ _ _ _ _ _ _ _ _ _ _ _ _ _ _ _ _ _ _ _ _ _ _ _ _ _ _ _ _ _ _ _ _ _ _ _ _ _ _ _]
                dyn-events: _ -> [_ _ _ _ _ _ _ _ _ _ _ _ _ _ _ _ _ _ _ _ _ _ _ _ _ _ _ _ _ _ _ _ _ _ _ _ _ _ _ _ _ _ _ _ _ _ _ _ _ _ _ _ _ _ _ _ _ _ _ _ _ _ _]
                timeout: 10 -> [_ _ _ _ _ _ _ _ _ _ _ _ _ _ _ _ _ _ _ _ _ _ _ _ _ _ _ _ _ _ _ _ _ _ _ _ _ _ _ _ _ _ _ _ _ _ _ _ _ _ _ _ _ _ _ _ _ _ _ _ _ _ _]
                tunnel: [w560 w592 w644 w1129 w1149 w1188 w1246 w1280 w1314 w1338 w1361 w1413 w1420 w1423 w1467 w1511 w1518 w1525 w1574 w1599 w1638 w1652 T48 [] ("Array 2") w1683 w1700 w1749 w1826 w1848 w1866 w1871 w1893 w1901 w1909 w1927 w1953 w1971 w1988 w1997 w2006 w2016 w2022 w2032 w2040 w2047 w2056 w2064 w2070 w2079 w2085 w2092 w2099 w2108 w2124 w2125 w2372 w2383 w2405 w2433 w2450 w2459 w2510 w2562 w2604] -> w551
                tunnel: "Case to View" -> [_ _ _ _ _ _ _ _ _ _ _ _ _ _ _ _ _ _ _ _ _ _ _ _ _ _ _ _ _ w1873 _ _ _ _ _ _ _ _ _ _ _ _ _ _ _ _ _ _ _ _ _ _ _ _ _ _ _ _ _ _ _ _ _]
                tunnel: w522 -> [w560 w592 w649 w1129 w1149 w1188 w1246 w1280 w1314 w1338 w1361 w1413 w1420 w1423 w1467 w1511 w1518 w1525 w1574 w1599 w1637 w1652 _ w1683 w1700 w1749 w1826 w1848 w1866 w1874 w1893 w1901 w1909 w1927 w1953 w1971 w1988 w1997 w2006 w2016 w2022 w2032 w2040 w2047 w2056 w2064 w2070 w2079 w2085 w2092 w2099 w2108 w2124 w2125 w2372 w2383 w2405 w2433 w2450 w2459 w2510 w2562 w2605]
                tunnel: w549 -> [_ _ w648 _ _ _ _ _ _ _ _ _ _ _ _ _ _ _ _ _ _ _ _ _ _ _ _ _ _ _ _ _ _ _ _ _ _ _ _ _ _ _ _ _ _ _ _ _ _ _ _ _ _ _ _ _ _ _ _ _ _ _ _]
                tunnel: "Sector Angle" -> [_ _ _ _ _ w1181 _ _ _ _ _ _ _ _ _ _ _ _ _ _ _ _ _ _ _ _ _ _ _ _ _ _ _ _ _ _ _ _ _ _ _ _ _ _ _ _ _ _ _ _ _ _ _ _ _ _ _ _ _ _ _ _ _]
                tunnel: w553 -> [_ _ w645 _ _ _ _ _ _ _ w1363 _ _ _ _ _ _ _ _ _ _ _ _ _ _ _ _ _ _ _ _ _ _ _ _ _ _ _ _ _ _ _ _ _ _ _ _ _ _ _ _ _ _ _ _ _ _ _ _ _ _ _ _]
                tunnel: w540 -> [_ _ _ _ _ _ _ _ _ _ _ _ _ _ _ _ _ _ _ _ _ _ _ _ w1684 _ _ _ _ _ _ _ _ _ _ _ _ _ _ _ _ _ _ _ _ _ _ _ _ _ _ _ _ _ _ _ _ _ _ _ _ _ _]
                tunnel: w555 -> [_ _ _ _ _ w1180 _ _ _ _ _ _ _ _ _ _ _ _ _ _ _ _ _ _ w1702 _ _ _ _ _ _ _ _ _ _ _ _ _ _ _ _ _ _ _ _ _ _ _ _ _ _ _ _ _ _ _ _ _ _ _ _ _ _]
                tunnel: w524 -> [_ _ w652 _ _ _ _ _ _ _ _ _ _ _ _ _ _ _ _ _ _ _ _ _ _ _ _ _ _ _ _ _ _ _ _ _ _ _ _ _ _ _ _ _ _ _ _ _ _ _ _ _ _ _ _ _ _ _ _ _ _ _ _]
                tunnel: w554 -> [_ _ w651 _ _ _ _ _ _ _ w1362 _ _ _ _ _ _ _ _ _ _ _ _ _ w1703 _ _ _ _ _ _ _ _ _ _ _ _ _ _ _ _ _ _ _ _ _ _ _ _ _ _ _ _ _ _ _ _ _ _ _ _ _ _]
                tunnel: w541 -> [_ _ w650 _ _ w1182 w1236 _ _ _ w1342 _ _ _ _ _ _ _ _ w1597 w1634 _ _ _ _ _ _ _ _ _ _ _ _ _ _ _ _ _ _ _ _ _ _ _ _ _ _ _ _ _ _ _ _ w2129 _ _ _ _ _ _ _ w2555 w2603]
                tunnel: w552 -> [w564 w598 w647 w1128 w1148 w1187 w1247 w1281 w1313 w1341 w1360 w1412 w1421 w1429 w1464 w1510 w1517 w1524 w1573 w1598 w1644 w1654 _ w1682 w1701 w1748 w1825 w1847 w1865 w1875 w1894 w1902 w1918 w1928 w1958 w1973 w1987 w1998 w2005 w2017 w2024 w2034 w2042 w2049 w2057 w2065 w2072 w2080 w2087 w2094 w2101 w2109 w2123 w2148 w2379 w2389 w2404 w2432 w2449 w2476 w2515 w2561 w2610]
                tunnel: [w564 w598 w646 w1128 w1148 w1187 w1247 w1281 w1313 w1341 w1360 w1412 w1421 w1429 w1464 w1510 w1517 w1524 w1573 w1598 w1644 w1654 0 w1682 w1701 w1748 w1825 w1847 w1865 w1875 w1894 w1902 w1918 w1928 w1958 w1973 w1987 w1998 w2005 w2017 w2024 w2034 w2042 w2049 w2057 w2065 w2072 w2080 w2087 w2094 w2101 w2109 w2123 w2148 w2379 w2389 w2404 w2432 w2449 w2476 w2515 w2561 w2610] -> w545
                tunnel: w542 -> [_ _ w643 _ _ _ _ _ _ _ w1359 _ _ _ _ _ _ _ _ _ _ _ _ _ _ _ _ _ _ _ _ _ _ _ _ _ _ _ _ _ _ _ _ _ _ _ _ _ _ _ _ _ _ _ _ _ _ _ _ _ _ _ _]
                tunnel: [_ _ _ _ _ _ _ _ _ _ _ _ _ _ _ _ _ _ _ _ _ _ _ _ _ _ _ _ _ _ _ _ _ _ _ _ _ _ _ _ _ TRUE TRUE _ _ _ _ _ _ _ _ _ _ _ _ _ _ _ _ _ _ _ w2600] -> w539
                tunnel: w538 -> [w559 w597 w642 w1118 w1143 w1154 w1241 w1276 w1312 w1337 w1357 w1411 w1419 w1428 w1437 w1509 w1516 w1520 w1572 w1592 w1643 w1648 w1660 w1681 w1694 w1746 w1824 w1846 w1864 w1870 w1888 w1900 w1908 w1926 w1945 w1968 w1986 w1996 w2004 w2013 w2021 w2028 w2039 w2046 w2055 w2063 w2069 w2075 w2084 w2091 w2098 w2107 w2122 w2143 w2376 w2388 w2391 w2431 w2448 w2454 w2513 w2537 w2609]
                tunnel: [w559 w597 w639 w1118 w1142 w1171 w1241 w1276 w1312 w1337 w1346 w1411 w1419 w1428 w1437 w1509 w1516 w1520 w1572 w1592 w1643 w1648 w1660 w1681 w1694 w1745 w1824 w1846 w1864 w1870 w1888 w1899 w1908 w1926 w1944 w1969 w1986 w1996 w2004 w2013 w2021 w2028 w2039 w2046 w2054 w2062 w2069 w2074 w2084 w2091 w2098 w2107 w2122 w2132 w2366 w2388 w2393 w2431 w2448 w2454 w2513 w2535 w2609] -> w537
                tunnel: w536 -> [w558 w596 w636 w1123 w1145 w1151 w1245 w1279 w1311 w1336 w1353 w1410 w1418 w1427 w1443 w1508 w1515 w1523 w1571 w1591 w1642 w1647 w1659 w1680 w1685 w1747 w1820 w1845 w1863 w1869 w1886 w1897 w1907 w1925 w1946 w1965 w1985 w1995 w2003 w2011 w2020 w2027 w2038 w2045 w2052 w2060 w2068 w2078 w2083 w2090 w2097 w2106 w2118 w2147 w2378 w2387 w2390 w2427 w2447 w2460 w2512 w2552 w2608]
                tunnel: [w558 w596 w640 w1123 w1145 w1155 w1242 w1277 w1311 w1335 w1356 w1410 w1418 w1427 w1443 w1508 w1515 w1523 w1571 w1591 w1642 w1647 w1659 w1680 w1685 w1744 w1822 w1845 w1863 w1869 w1884 w1897 w1907 w1924 w1946 w1964 w1985 w1994 w2001 w2011 w2020 w2027 w2038 w2045 w2052 w2060 w2068 w2078 w2083 w2090 w2097 w2105 w2117 w2137 w2371 w2387 w2390 w2427 w2447 w2460 w2512 w2536 w2608] -> w535
                tunnel: w534 -> [_ _ w641 _ _ w1170 w1240 w1275 _ _ _ _ _ _ _ _ _ _ _ _ _ _ _ _ _ w1741 _ w1844 _ _ _ _ _ _ _ _ _ _ _ _ _ _ _ _ _ _ _ _ _ _ _ _ _ _ _ _ _ _ _ _ _ _ _]
                tunnel: w533 -> [w557 w595 w631 w1127 w1147 w1167 w1239 w1274 w1296 w1332 w1343 w1409 w1417 w1426 w1438 w1507 w1514 w1522 w1570 w1590 w1641 w1646 w1658 w1679 w1697 w1742 w1821 w1843 w1862 w1868 w1881 w1896 w1906 w1921 w1938 w1962 w1984 w1993 w2002 w2010 w2019 w2026 w2037 w2044 w2051 w2059 w2067 w2077 w2082 w2089 w2096 w2104 w2121 w2128 w2363 w2386 w2403 w2430 w2446 w2457 w2511 w2517 w2607]
                tunnel: w532 -> [_ _ w632 _ _ _ _ _ _ _ _ _ _ _ _ _ _ _ _ _ _ _ _ _ _ w1736 _ w1841 _ _ _ _ _ _ _ _ _ _ _ _ _ _ _ _ _ _ _ _ _ _ _ _ _ _ _ _ _ _ _ _ _ w2527 _]
                tunnel: w531 -> [_ _ _ _ _ _ _ _ _ _ _ _ _ _ _ _ _ _ _ _ _ _ _ _ _ _ _ _ _ _ _ _ _ _ w1939 _ _ _ _ _ _ _ _ _ _ _ _ _ _ _ _ _ _ _ _ _ _ _ _ _ _ _ _]
                tunnel: [w557 w595 w638 w1127 w1147 w1168 w1238 w1273 w1296 w1332 w1354 w1409 w1417 w1426 w1438 w1507 w1514 w1522 w1570 w1590 w1641 w1646 w1658 w1679 w1697 w1742 w1821 w1842 w1862 w1868 w1881 w1896 w1906 w1921 w1938 w1962 w1984 w1993 w2002 w2010 w2019 w2026 w2037 w2044 w2051 w2059 w2067 w2077 w2082 w2089 w2096 w2104 w2121 w2127 w2362 w2386 w2403 w2430 w2446 w2457 w2511 w2517 w2607] -> w530
                tunnel: w529 -> [_ w591 w637 _ _ _ _ _ _ _ w1351 _ _ _ _ _ _ _ _ _ w1635 _ _ _ w1686 _ w1818 _ _ _ _ _ _ _ _ _ _ _ _ _ _ _ _ _ _ _ _ _ _ _ _ _ _ _ _ _ _ w2426 _ _ _ _ w2599]
                tunnel: w528 -> [_ _ _ _ _ _ _ _ _ _ _ _ _ _ _ _ _ _ _ _ _ _ _ _ _ _ _ _ _ _ _ _ w1904 _ _ _ _ _ _ _ _ _ _ _ _ _ _ _ _ _ _ _ _ _ _ _ _ _ _ w2456 _ _ _]
                tunnel: [_ _ _ _ _ _ _ _ _ _ _ _ _ _ _ _ _ _ _ _ _ _ _ _ _ _ _ _ _ _ _ _ _ _ _ _ _ _ _ _ _ _ _ _ _ _ _ _ _ _ _ _ _ _ _ _ _ _ _ _ _ _ w2600] -> w527
                tunnel: w525 -> [w556 w590 w635 w1126 w1146 w1166 w1237 w1272 w1310 w1330 w1349 w1408 w1416 w1422 w1434 w1506 w1513 w1521 w1569 w1584 w1639 w1645 w1656 w1678 w1695 w1740 w1816 w1840 w1858 w1867 w1880 w1895 w1903 w1920 w1937 w1961 w1983 w1989 w1999 w2007 w2018 w2025 w2036 w2043 w2050 w2058 w2066 w2076 w2081 w2088 w2095 w2103 w2120 w2146 w2377 w2385 w2402 w2429 w2445 w2455 w2509 w2516 w2606]
                tunnel: [w556 w590 w634 w1126 w1146 w1166 w1237 w1272 w1310 w1330 w1348 w1408 w1415 w1422 w1434 w1506 w1513 w1521 w1569 w1584 w1639 w1645 w1656 w1678 w1695 w1738 w1816 w1840 w1856 w1867 w1880 w1895 w1903 w1920 w1936 w1961 w1983 w1989 w1999 w2007 w2018 w2025 w2036 w2043 w2050 w2058 w2066 w2076 w2081 w2088 w2095 w2103 w2120 w2146 w2377 w2385 w2402 w2429 w2445 w2455 w2509 w2516 w2606] -> w526
                tunnel: w523 -> [_ _ _ _ _ _ _ _ _ _ _ _ _ _ _ _ _ w1519 w1568 _ _ _ _ _ _ _ _ _ _ _ _ _ _ _ _ _ _ _ _ _ _ _ _ _ _ _ _ _ _ _ _ _ _ _ _ _ _ _ _ _ _ _ _]
                event Timeout {
                  n210 = event-data() -> ()  [unwired: 3 out]
                  n211 = property class="VI"() -> (reference out=w563:refnum<vi>, error out=w561:errorcluster, "Front Panel.IsFrontmost"=w562:bool)  [unwired: 2 in]
                  n212 = case shown="True" w562 {
                    tunnel: w563 -> [w567 _]
                    tunnel: w561 -> [w565 _]
                    frame False {
                      n213 = property class="VI"(reference=w567, error in=w565, "Front Panel.IsFrontmost"=TRUE) -> ()  [unwired: 2 out]
                    }
                    frame True {
                    }
                  }
                }
                event Key Down {
                  n214 = event-data() -> ("VKey"=w594:T54, "Char"=w593:i16)  [unwired: 1 out]
                  n215 = property on="Scan to View" class="DigNum (strict)"() -> ("Key Focus"=w570:bool)  [unwired: 2 in, 2 out]
                  n216 = property on="Filter Prams" class="Clust (strict)"() -> ("Key Focus"=w575:bool)  [unwired: 2 in, 2 out]
                  n217 = property on="Case to View" class="Ring (strict)"() -> ("Key Focus"=w569:bool)  [unwired: 2 in, 2 out]
                  n218 = property on="Transducer" class="DigNum (strict)"() -> ("Key Focus"=w581:bool)  [unwired: 2 in, 2 out]
                  n219 = property on="OPTIONS" class="TabCtl (strict)"() -> ("Key Focus"=w577:bool)  [unwired: 2 in, 2 out]
                  n220 = property on="TimeOut (s)" class="DigNum (strict)"() -> ("Key Focus"=w568:bool)  [unwired: 2 in, 2 out]
                  n221 = property on="Case Name" class="Str"() -> ("Key Focus"=w589:bool)  [unwired: 2 in, 2 out]
                  n222 = property on="lines per plane" class="DigNum (strict)"() -> ("Key Focus"=w588:bool)  [unwired: 2 in, 2 out]
                  n223 = property on="Trans Geometry (mm)" class="Clust (strict)"() -> ("Key Focus"=w578:bool)  [unwired: 2 in, 2 out]
                  n224 = property on="low cutoff" class="DigNum (strict)"() -> ("Key Focus"=w574:bool)  [unwired: 2 in, 2 out]
                  n225 = property on="Distance between\nscan lines (um)" class="DigNum (strict)"() -> ("Key Focus"=w587:bool)  [unwired: 2 in, 2 out]
                  n226 = property on="Length of\none plane (mm)" class="DigNum (strict)"() -> ("Key Focus"=w586:bool)  [unwired: 2 in, 2 out]
                  n227 = property on="Focal Zones" class="DigNum (strict)"() -> ("Key Focus"=w579:bool)  [unwired: 2 in, 2 out]
                  n228 = property on="order" class="DigNum (strict)"() -> ("Key Focus"=w573:bool)  [unwired: 2 in, 2 out]
                  n229 = property on="high cutoff" class="DigNum (strict)"() -> ("Key Focus"=w572:bool)  [unwired: 2 in, 2 out]
                  n230 = property on="number of planes" class="DigNum (strict)"() -> ("Key Focus"=w585:bool)  [unwired: 2 in, 2 out]
                  n231 = property on="Avg Num" class="DigNum (strict)"() -> ("Key Focus"=w584:bool)  [unwired: 2 in, 2 out]
                  n232 = property on="Overshoot" class="DigNum (strict)"() -> ("Key Focus"=w580:bool)  [unwired: 2 in, 2 out]
                  n233 = property on="Transducer" class="DigNum (strict)"() -> ("Key Focus"=w571:bool)  [unwired: 2 in, 2 out]
                  n234 = property on="Length of\nall planes (mm)" class="DigNum (strict)"() -> ("Key Focus"=w582:bool)  [unwired: 2 in, 2 out]
                  n235 = property on="Distance between\nplanes (um)" class="DigNum (strict)"() -> ("Key Focus"=w583:bool)  [unwired: 2 in, 2 out]
                  n236 = Compound Arithmetic op=OR(w568, w569, w570, w589, w588, w587, w586, w585, w584, w583, w582, w581, w580, w579, w578, w577, w575, w574, w573, w572, w571) -> (w576:bool)
                  n237 = case shown="False" w576 {
                    tunnel: w594 -> [w605 _]
                    tunnel: w593 -> [w602 _]
                    tunnel: w591 -> [w599 _]
                    frame False {
                      n238 = property on="Case to View" class="Ring (strict)"() -> ("Strings []"=w600:string[], "Value"=w603:u16)  [unwired: 2 in, 2 out]
                      n239 = property on="Scan to View" class="DigNum (strict)"() -> ("Value"=w604:u32)  [unwired: 2 in, 2 out]
                      n240 = Array Size(array=w600) -> (size(s)=w601:i32)
                      n241 = case shown="\"Down\"" w605 {
                        tunnel: w604 -> [_ _ _ _ w625 w626]
                        tunnel: w603 -> [_ w616 w621 _ _ _]
                        tunnel: w602 -> [w606 _ _ _ _ _]
                        tunnel: w601 -> [_ w612 w617 _ _ _]
                        tunnel: w599 -> [_ _ _ w622 _ _]
                        frame "ASCII", Default {
                          n242 = case shown="80, 112" w606 {
                            frame Default {
                            }
                            frame 88, 120 {
                              n243 = property on="Raw data" class="IntGraph (strict)"("XScale.ScaleFit"=u8 1 ("X Scale.Scale Fit")) -> ()  [unwired: 2 in, 2 out]
                            }
                            frame 83, 115 {
                              n244 = property on="Save Data" class="Bool (strict)"("Val(Sgnl)"=TRUE ("Value (Signaling)")) -> ()  [unwired: 2 in, 2 out]
                            }
                            frame 80, 112 {
                              n245 = property on="Take Webcam pic" class="Bool (strict)"("Val(Sgnl)"=TRUE ("Value (Signaling)")) -> ()  [unwired: 2 in, 2 out]
                            }
                            frame 89, 121 {
                              n246 = property on="Raw data" class="IntGraph (strict)"("YScale.ScaleFit"=u8 1 ("X Scale.Scale Fit")) -> ()  [unwired: 2 in, 2 out]
                            }
                          }
                        }
                        frame "Left" {
                          n247 = Decrement(x=w612) -> (x-1=w611:i32)
                          n248 = Decrement(x=w616) -> (x-1=w613:u16)
                          n249 = In Range and Coerce(upper limit=w611, x=w613, lower limit=u16 0) -> (coerced(x)=w614:i32)  [unwired: 1 out]
                          n250 = property on="Case to View" class="Ring (strict)"("Val(Sgnl)"=w614) -> ()  [unwired: 2 in, 2 out]
                        }
                        frame "Right" {
                          n251 = Increment(x=w621) -> (x+1=w620:u16)
                          n252 = In Range and Coerce(upper limit=w617, x=w620, lower limit=u16 0) -> (coerced(x)=w619:i32)  [unwired: 1 out]
                          n253 = property on="Case to View" class="Ring (strict)"("Val(Sgnl)"=w619) -> ()  [unwired: 2 in, 2 out]
                        }
                        frame "Enter" {
                          n254 = case shown="\"Automatic\", Default" w622 {
                            frame "Automatic", Default {
                            }
                            frame "Stony Brook" {
                              n255 = property on="start scan" class="Bool (strict)"("Val(Sgnl)"=TRUE ("Value (Signaling)")) -> ()  [unwired: 2 in, 2 out]
                            }
                          }
                        }
                        frame "Up" {
                          n256 = Increment(x=w625) -> (x+1=w624:u32)
                          n257 = property on="Scan to View" class="DigNum (strict)"("Val(Sgnl)"=w624) -> ()  [unwired: 2 in, 2 out]
                        }
                        frame "Down" {
                          n258 = case shown="Default" w626 {
                            selector: w626 -> [w628 w629]
                            tunnel: [w628 w630] -> w627
                            frame 0 {
                            }
                            frame Default {
                              n259 = Decrement(x=w629) -> (x-1=w630:u32)
                            }
                          }
                          n260 = property on="Scan to View" class="DigNum (strict)"("Val(Sgnl)"=w627) -> ()  [unwired: 2 in, 2 out]
                        }
                      }
                    }
                    frame True {
                    }
                  }
                }
                event "start scan": Value Change {
                  n261 = event-data() -> ()  [unwired: 2 out]
                  n262 = stacked-sequence {
                    seq-local: [_ _ w732 _ _ _] -> [_ _ _ _ w1075 _]
                    seq-local: [_ _ w733 _ _ _] -> [_ _ _ _ w1074 _]
                    seq-local: [_ _ w734 _ _ _] -> [_ _ _ w1058 _ _]
                    seq-local: [_ w711 _ _ _ _] -> [_ _ w731 _ _ _]
                    seq-local: [_ _ w730 _ _ _] -> [_ _ _ w1054 _ _]
                    seq-local: [w662 _ _ _ _ _] -> [_ _ _ w1049 _ _]
                    tunnel: w652 -> [_ _ w726 _ _ _]
                    tunnel: w651 -> [_ _ w751 _ _ _]
                    tunnel: w650 -> [w657 _ w750 w1052 _ _]
                    tunnel: w649 -> [w663 _ _ _ _ _]
                    tunnel: w648 -> [_ _ w749 _ _ _]
                    tunnel: w647 -> [_ _ w748 _ _ _]
                    tunnel: [_ _ w747 _ _ _] -> w646
                    tunnel: w645 -> [_ _ w746 _ _ _]
                    tunnel: [_ _ _ w1057 _ _] -> w644
                    tunnel: w643 -> [_ _ _ _ _ _]
                    tunnel: w642 -> [_ _ w745 _ _ _]
                    tunnel: w641 -> [_ _ w744 _ _ _]
                    tunnel: [_ _ w732 _ _ _] -> w640
                    tunnel: [_ _ w733 _ _ _] -> w639
                    tunnel: [_ _ w718 _ _ _] -> w638
                    tunnel: w637 -> [w656 _ w725 _ _ _]
                    tunnel: w636 -> [w655 _ w728 _ _ _]
                    tunnel: w635 -> [_ _ w724 _ _ _]
                    tunnel: [_ _ w723 _ _ _] -> w634
                    tunnel: w632 -> [_ _ w722 _ _ _]
                    tunnel: w631 -> [_ _ w719 _ _ _]
                    frame #0 {
                      n263 = global write "DigitizerGlobals.vi" "2nd Channel HZ Offset?"("2nd Channel HZ Offset?") -> ()
                      n264 = global write "DigitizerGlobals.vi" "Read HZ Offset?"("Read HZ Offset?") -> ()
                      n265 = global write "MotionGlobals.vi" "Preview Configed?"(FALSE ("Popped Up Before?")) -> ()
                      n266 = global write "MotionGlobals.vi" "Limit Warned?"(FALSE ("Popped Up Before?")) -> ()
                      n267 = case shown="\"M scan\", Default" w657 {
                        selector: w657 -> [_ w681 _]
                        tunnel: w663 -> [w678 w683 w705]
                        tunnel: [w678 w682 w705] -> w662
                        tunnel: w655 -> [w677 w680 w703]
                        tunnel: w656 -> [_ w679 w702]
                        tunnel: [w677 w680 w701] -> w653
                        frame "M scan", Default {
                        }
                        frame "Dual Transducer" {
                          n268 = Index Array(array=w683) -> (element=w685:T55)  [unwired: 1 in]
                          n269 = Unbundle By Name(w685) -> ("Keep?"=w684:bool)
                          n270 = case shown="True" w684 {
                            tunnel: w683 -> [w686 w690]
                            tunnel: [w686 w689] -> w682
                            tunnel: w681 -> [_ w688]
                            tunnel: w679 -> [_ w687]
                            frame False {
                            }
                            frame True {
                              n271 = Two Button Dialog(message="Unsaved Data Exists", 1:"Continue" ("F button name (\"Cancel\")"), 2:"Save Now" ("T button name (\"OK\")")) -> (T button?=w691:bool)
                              n272 = case shown="True" w691 {
                                tunnel: w690 -> [w695 w698]
                                tunnel: [w695 w696] -> w689
                                tunnel: w688 -> [_ w700]
                                tunnel: w687 -> [_ w699]
                                frame False {
                                }
                                frame True {
                                n273 = control-ref of="Erase data"() -> (w697:refnum<vi>)
                                n274 = call "SaveDataAcqCont.vi"("Boolean in"=w697, "Array in"=w698, "Location"=w699, "Type of scan"=w700) -> ("Array out"=w696:T55[])  [unwired: 6 in, 1 out]
                                }
                              }
                            }
                          }
                        }
                        frame "Acoustic Microscopy" {
                          n275 = property on="Pulse" class="Bool (strict)"() -> ("Value"=w704:bool)  [unwired: 2 in, 2 out]
                          n276 = case shown="True" w704 {
                            tunnel: w703 -> [w706 w710]
                            tunnel: w702 -> [_ w709]
                            tunnel: [w706 w708] -> w701
                            frame False {
                            }
                            frame True {
                              n277 = call "PRF_Off.vi"("Location"=w709, "Motion Settings In"=w710) -> ("Motion Settings Out"=w708:T10)  [unwired: 9 in]
                              n278 = Wait (ms)(milliseconds to wait=u32 500) -> ()  [unwired: 1 out]
                            }
                          }
                        }
                      }
                      n279 = Unbundle By Name(w653) -> ("Motion System"=w659:T11)
                      n280 = case shown="\"Galil\"" w659 {
                        tunnel: w653 -> [_ w664 _]
                        frame "MM3000", Default {
                        }
                        frame "NI 735x" {
                          n281 = disable-structure shown="Disabled" {
                            disable-tunnel: w664 -> [w666 _]
                            frame Disabled {
                              n282 = Unbundle By Name(w666) -> ("Motion Bd ID"=w665:u8)
                              n283 = while {
                                tunnel: w665 -> [w675]
                                i -> [w668]
                                stop <- w671 stop-if-true
                                n284 = call <vilib>:"Flush Return Data Buffer.flx"("Board ID"=w675) -> ("error out"=w674:errorcluster, "Bd ID Out"=w676:T56)  [unwired: 6 in]
                                n285 = call <vilib>:"Clear Faults.vi"("error in (no error)"=w674, "board in"=w676) -> ("error out"=w673:errorcluster)  [unwired: 8 in, 1 out]
                                "error out" <- w673
                                n286 = Unbundle(w673) -> ("status"=w672:bool)  [unwired: 2 out]
                                n287 = Not(x=w672) -> (.not. x?=w669:bool)
                                n288 = Greater?(x=w668, y=5 ("x")) -> (0:w670:bool)
                                n289 = Or(x=w669, y=w670) -> (x .or. y?=w671:bool)
                              }
                            }
                            frame Enabled {
                            }
                          }
                        }
                        frame "Galil" {
                        }
                      }
                    }
                    frame #1 {
                      n290 = control-ref of="lines per plane"() -> (w717:refnum<vi>)
                      n291 = control-ref of="Distance between\nscan lines (um)"() -> (w716:refnum<vi>)
                      n292 = control-ref of="Length of\none plane (mm)"() -> (w715:refnum<vi>)
                      n293 = control-ref of="number of planes"() -> (w714:refnum<vi>)
                      n294 = control-ref of="Distance between\nplanes (um)"() -> (w713:refnum<vi>)
                      n295 = control-ref of="Length of\nall planes (mm)"() -> (w712:refnum<vi>)
                      n296 = Bundle("lines per plane"=w717, "Distance between\nscan lines (um)"=w716, "Length of\none plane (mm)"=w715, "number of planes"=w714, "Distance between\nplanes (um)"=w713, "Length of\nall planes (mm)"=w712) -> (w711:T57)  [unwired: 1 in]
                    }
                    frame #2 {
                      # "take data, move motors etc."
                      n297 = control-ref of="Case temp"() -> (w739:refnum<vi>)
                      n298 = call "MotionProfileChange.vi"("Motion Mode"=enum16{"Move Mode", "Scan Mode"}."Scan Mode", "Location"=w725, "Motion Settings In in"=w728) -> ("Motion Settings In out"=w729:T10)  [unwired: 8 in]
                      n299 = case shown="\"M scan\", Default" w750 {
                        selector: w750 -> [w752 w773 w801 w865 w903 w999 w1007]
                        tunnel: w751 -> [_ w794 _ _ _ _ w1031]
                        tunnel: [w768 w793 _ w888 w924 _ w1030] -> w743
                        tunnel: [w765 w787 w805 w883 w921 w1003 w1024] -> w734
                        tunnel: w746 -> [w769 _ _ _ _ _ _]
                        tunnel: w726 -> [_ _ _ _ _ _ _]
                        tunnel: "Resp Divide" -> [_ w791 _ _ _ _ w1028]
                        tunnel: "Email" -> [_ w790 _ _ _ _ w1027]
                        tunnel: w745 -> [w767 w789 w826 w892 w928 w1005 w1022]
                        tunnel: [w767 w789 w804 w889 w925 w1005 w1026] -> w733
                        tunnel: w729 -> [w766 w788 w825 w893 w927 w1004 w1025]
                        tunnel: [w766 w788 w808 w890 w922 w1004 w1023] -> w732
                        tunnel: w744 -> [_ _ _ _ w923 _ _]
                        tunnel: "Add Axis" -> [w759 w780 w821 w872 w920 w1000 w1016]
                        tunnel: w739 -> [w762 w783 w822 w870 w914 w993 w1018]
                        tunnel: w749 -> [w761 w782 w823 w871 w919 w998 w1017]
                        tunnel: "Case temp" -> [w757 w779 w819 w866 w918 w995 w1015]
                        tunnel: w748 -> [w763 w784 w820 w869 w916 w997 w1019]
                        tunnel: [w758 w785 w824 w868 w915 w996 w1020] -> w747
                        tunnel: "Case Name" -> [w760 w781 w799 w875 w917 w1001 w1012]
                        tunnel: [w756 w778 w818 w867 w912 w994 w1014] -> w737
                        tunnel: "Skip Real Time Setup" -> [_ _ _ _ w911 _ _]
                        tunnel: w731 -> [_ _ _ _ w908 _ _]
                        tunnel: [w755 w777 w806 w882 w907 w992 w1013] -> w730
                        tunnel: w725 -> [_ _ w816 _ _ _ _]
                        tunnel: w724 -> [w754 w775 w811 w877 w900 w991 w1009]
                        tunnel: [w754 w775 w802 w877 w904 w989 w1008] -> w723
                        tunnel: w722 -> [_ _ _ _ w902 _ _]
                        tunnel: variant ("Value") -> [_ _ _ w863 _ _ _]
                        tunnel: T46 {"yo"=0.0, "dx"=0.0, "output array"=[]} ("Waveform Graph") -> [_ _ _ w864 _ _ _]
                        tunnel: w719 -> [w753 w772 w800 w862 w897 w988 w1006]
                        tunnel: [w753 w772 w800 w862 w896 w988 w1006] -> w718
                        frame "Therapy With Scan" {
                          # "Fire therapy in middle of A scan"
                          n300 = call "FileNameGenerator.vi"("Type of scan"=w752, "Case temp"=w757, "Add Axis"=w759, "Current Plane in"=w763, "String in"=w762, "Boolean"=w761, "Case Name in"=w760) -> ("Current Plane out"=w758:i32, "Root Case Name"=w756:string, "Case Name out"=w764:string)  [unwired: 2 in]
                          n301 = call "Therapy&Scan.vi"("VISA session in"=w769, "File Name In"=w764, "Motion Settings"=w766, "Therapy Parameters"="Therapy Parameters", "Digitizer Settings"=w767) -> ("Error Message"=w768:string, "Scan Params"=w771:T55)  [unwired: 3 in, 2 out]
                          n302 = Build Array(w771) -> (w765:T55[])
                          n303 = Build Array(w764) -> (w755:string[])
                        }
                        frame "M scan", Default {
                          n304 = Unbundle By Name(w775) -> ("Full Array Scan?"=w776:bool)
                          n305 = case shown="\"Acoustic Microscopy\"" w773 {
                            tunnel: [T7."Level X" ("Value") w796] -> w774
                            frame "Therapy With Scan", Default {
                            }
                            frame "Acoustic Microscopy" {
                              n306 = property on="Microscopy Scan Mode" class="RadioBtnsControl (strict)"() -> ("Value"=w796:T7)  [unwired: 2 in, 2 out]
                            }
                          }
                          n307 = call "FileNameGenerator.vi"("Type of scan"=w773, "Case temp"=w779, "Add Axis"=w780, "Current Plane in"=w784, "String in"=w783, "Boolean"=w782, "Case Name in"=w781) -> ("Current Plane out"=w785:i32, "Root Case Name"=w778:string, "Case Name out"=w786:string)  [unwired: 2 in]
                          n308 = call "DigData.vi"("Type of scan"=w773, "Digitizer Settings"=w789, "File Name In"=w786, "Therapy (T)"=w794, "Ann Array Params"=w775, "Motion Settings In"=w788, "recipient"=w790, "Microscopy Scan Mode"=w774, "Breath Divide"=w791) -> ("Scan Params"=w792:T55, "Error Message"=w793:string)  [unwired: 6 in, 11 out]
                          n309 = Build Array(w786) -> (w777:string[])
                          n310 = case shown="False" w776 {
                            frame False {
                            }
                            frame True {
                              n311 = property on="Transducer" class="DigNum (strict)"("Val(Sgnl)"=u32 1 ("Value (Signaling)")) -> ()  [unwired: 2 in, 2 out]
                            }
                          }
                          n312 = Build Array(w792) -> (w787:T55[])
                        }
                        frame "Real-Time Scan" {
                          # "Real time scan"
                          n313 = Unbundle By Name(w811) -> ("Synth Foc?"=w812:bool)
                          n314 = Equal?(x=w816, y=location."NYU") -> (x = y?=w814:bool)
                          n315 = Or(x=w812, y=w814) -> (x .or. y?=w813:bool)
                          n316 = case shown="True" w813 {
                            tunnel: w826 -> [w851 w861]
                            tunnel: [w850 w858] -> w809
                            tunnel: w825 -> [w849 w860]
                            tunnel: [w842 w859] -> w798
                            tunnel: w799 -> [w848 w857]
                            tunnel: [w847 w857] -> w817
                            tunnel: w811 -> [w846 w856]
                            tunnel: [w843 w854] -> w803
                            tunnel: [w845 T47."Exit" ("Dual XDCR Mode")] -> w810
                            tunnel: w801 -> [w844 _]
                            frame False {
                              n317 = call "RealTimeSingle.vi"("Digitizer Settings"=w851, "File Name"=w848, "Motion Settings"=w849, "Type of scan"=w844, "Ann Array Params"=w846, "return to start"=TRUE) -> ("Ann Array Params Out"=w843:T50, "Dual XDCR Mode"=w845:T47, "Digitizer Settings Out"=w850:T13, "File Name Out"=w847:string, "Motion Settings Out"=w842:T10)  [unwired: 7 in, 2 out]
                            }
                            frame True {
                              n318 = call "Real Time_Master.vi"("File Name"=w857, "Ann Array Params"=w856, "Motion Settings"=w860, "Digitizer Settings"=w861) -> ("Ann Array\nParams Out"=w854:T50, "Motion Settings Out"=w859:T10, "Digitizer Settings Out"=w858:T13)  [unwired: 5 in]
                              n319 = Unbundle By Name(w854) -> ("Trans Geometry (mm)"=w853:T8)
                              n320 = local write "Trans Geometry (mm)"(w853) -> ()
                            }
                          }
                          n321 = call "FileNameGenerator.vi"("Type of scan"=w801, "Case temp"=w819, "Add Axis"=w821, "Current Plane in"=w820, "String in"=w822, "Boolean"=w823, "Case Name in"=w817) -> ("Current Plane out"=w824:i32, "Root Case Name"=w818:string, "Case Name out"=w807:string)  [unwired: 2 in]
                          n322 = case shown="\"Exit\", Default" w810 {
                            selector: w810 -> [w836 _]
                            tunnel: w798 -> [w835 w838]
                            tunnel: w809 -> [w834 w839]
                            tunnel: [w833 w838] -> w808
                            tunnel: w807 -> [w832 w841]
                            tunnel: [w831 w840] -> w806
                            tunnel: [w830 _] -> w805
                            tunnel: [w829 w839] -> w804
                            tunnel: w803 -> [w828 w837]
                            tunnel: [w827 w837] -> w802
                            frame "Transducer 1" {
                              n323 = call "Dual XDCR Scan.vi"("Digitizer Settings In"=w834, "Dual XDCR Mode"=w836, "Motion Settings In"=w835, "Ann Array Params"=w828, "Case Name"=w832) -> ("Ann Array Params"=w827:T50, "Case Names"=w831:string[], "Digitizer Settings"=w829:T13, "Motion Settings"=w833:T10, "Scan Params Array"=w830:T55[])  [unwired: 8 in, 2 out]
                            }
                            frame "Exit", Default {
                              n324 = Build Array(w841) -> (w840:string[])
                            }
                          }
                        }
                        frame "Hydrophone Scanning" {
                          w878 = u16 3 items=["Therapy With Scan", "M scan", "M Scan With Therapy Burst", "1-D B Scan", "1-D B Scan With Therapy Burst", "2-D B Scan", "2-D B Scan With Therapy Burst", "Rotational Scan", "1-D B-Scan PRF", "2-D B-Scan PRF", "Real-Time Scan", "Contrast Agents", "1-D w/ Real-Time Set Up", "Amplifier blah blah"] ("Type of scan")
                          w879 = u16 5 items=["Therapy With Scan", "M scan", "M Scan With Therapy Burst", "1-D B Scan", "1-D B Scan With Therapy Burst", "2-D B Scan", "2-D B Scan With Therapy Burst", "Rotational Scan", "1-D B-Scan PRF", "2-D B-Scan PRF", "Real-Time Scan", "Contrast Agents", "1-D w/ Real-Time Set Up", "Amplifier blah blah"] ("Type of scan")
                          n325 = property on="Hydrophopne Waveform Graph" class="WFGraph (strict)"("Value"=w864) -> ()  [unwired: 2 in, 2 out]
                          n326 = property on="3D Surface" class="AXCont"("Value"=w863) -> ()  [unwired: 2 in, 2 out]
                          n327 = property on="Length of\none plane (mm)" class="DigNum (strict)"() -> ("Value"=w887:dbl)  [unwired: 2 in, 2 out]
                          n328 = property on="Length of\nall planes (mm)" class="DigNum (strict)"() -> ("Value"=w881:dbl)  [unwired: 2 in, 2 out]
                          n329 = property on="number of planes" class="DigNum (strict)"() -> ("Value"=w886:u16)  [unwired: 2 in, 2 out]
                          n330 = call "FileNameGenerator.vi"("Type of scan"=w865, "Case temp"=w866, "Add Axis"=w872, "Current Plane in"=w869, "String in"=w870, "Boolean"=w871, "Case Name in"=w875) -> ("Current Plane out"=w868:i32, "Root Case Name"=w867:string, "Case Name out"=w874:string)  [unwired: 2 in]
                          n331 = flat-sequence {
                            tunnel: w876 -> [w894]
                            frame #0 {
                              "Scan data" <- w894
                            }
                            frame #1 {
                              n332 = property on="Parameter Selection" class="Ring (strict)"() -> ("Value"=w895:u16)  [unwired: 2 in, 2 out]
                              n333 = property on="Parameter Selection" class="Ring (strict)"("Val(Sgnl)"=w895) -> ()  [unwired: 2 in, 2 out]
                            }
                          }
                          n334 = Not Equal To 0?(x=w881) -> (x != 0?=w880:bool)
                          n335 = Select(t=w879, s=w880, f=w878) -> (s? t:f=w873:u16)
                          n336 = call "RapidScan.vi"("File Name?"=w874, "Scan Length (mm)"=w887, "Scan Len (mm) Ax2"=w881, "Number of pts\nAx 2"=w886, "Pressure Cal Parameters"="Pressure Cal Parameters", "Type of scan"=w873, "Therapy"=FALSE, "Digitizer Settings"=w892, "Motion Settings"=w893) -> ("Scan data"=w876:T1, "Digitizer Settings Out"=w889:T13, "Scan Params"=w884:T55, "Motion Settings Out"=w890:T10, "Error Message"=w888:string)  [unwired: 6 in]
                          n337 = property on="Plot" class="TabCtl (strict)"("Val(Sgnl)"=w873) -> ()  [unwired: 2 in, 2 out]
                          n338 = Build Array(w884) -> (w883:T55[])
                          n339 = Build Array(w874) -> (w882:string[])
                        }
                        frame "Dual Transducer" {
                          n340 = Unbundle By Name(w900) -> ("Switch T/R"=w899:i16)
                          n341 = property on="Attenuation Scan" class="Bool (strict)"() -> ("Value"=w901:bool)  [unwired: 2 in, 2 out]
                          n342 = Decrement(x=w899) -> (x-1=w898:i16)
                          n343 = case shown="True" w911 {
                            tunnel: w928 -> [w941 w953]
                            tunnel: w927 -> [w940 w950]
                            tunnel: [w939 w952] -> w926
                            tunnel: [w938 w951] -> w909
                            tunnel: w917 -> [w936 w949]
                            tunnel: [w933 w948] -> w906
                            tunnel: [w935 w954] -> w913
                            tunnel: [w934 w947] -> w905
                            tunnel: w900 -> [w932 w947]
                            tunnel: w903 -> [w931 _]
                            tunnel: w902 -> [_ w946]
                            tunnel: w901 -> [_ w945]
                            tunnel: w898 -> [_ w944]
                            tunnel: w897 -> [w930 w943]
                            tunnel: [w929 w942] -> w896
                            frame False {
                              n344 = call "RealTimeSingle.vi"("Digitizer Settings"=w941, "File Name"=w936, "Motion Settings"=w940, "Type of scan"=w931, "Ann Array Params"=w932, "return to start"=TRUE, "Dual XDCR Settings"=w930) -> ("Dual XDCR Settings Out"=w929:T24, "Ann Array Params Out"=w934:T50, "Dual XDCR Mode"=w935:T47, "Digitizer Settings Out"=w939:T13, "File Name Out"=w933:string, "Motion Settings Out"=w938:T10)  [unwired: 6 in, 1 out]
                              n345 = property on="Case Name" class="Str"("Value"=w933) -> ()  [unwired: 2 in, 2 out]
                            }
                            frame True {
                              n346 = case shown="False" w945 {
                                tunnel: [w965 w969] -> w954
                                tunnel: w953 -> [w964 w971]
                                tunnel: [w963 w971] -> w952
                                tunnel: [w962 w970] -> w951
                                tunnel: w950 -> [w961 w970]
                                tunnel: w949 -> [w960 w972]
                                tunnel: [w959 w972] -> w948
                                tunnel: w946 -> [w958 _]
                                tunnel: w944 -> [w957 w968]
                                tunnel: w943 -> [w956 w966]
                                tunnel: [w955 w966] -> w942
                                frame False {
                                n347 = call "DualXDCRFastSetup.vi"("Dual XDCR Settings"=w956, "Pulser"=w958, "Switch T/R In"=w957, "Motion Settings in"=w961, "File Name In"=w960, "Digitizer Settings in"=w964) -> ("Dual XDCR Mode Out"=w965:T47, "System Motion Settings"=w962:T10, "File Name Out"=w959:string, "System Digitizer Settings"=w963:T13, "Dual XDCR Settings Out"=w955:T24)  [unwired: 1 in]
                                }
                                frame True {
                                n348 = call "DualXDCRUserPrompt.vi"("Dual XDCR Settings"=w966, "Current XDCR"=w968, "Auto Dual?"=FALSE) -> ("Dual XDCR Mode"=w969:T47)  [unwired: 7 in, 1 out]
                                }
                              }
                            }
                          }
                          n349 = case shown="Default" w913 {
                            tunnel: [w973 w984] -> w910
                            tunnel: w920 -> [_ w983]
                            tunnel: w919 -> [_ w982]
                            tunnel: w918 -> [_ w977]
                            tunnel: w916 -> [w974 w981]
                            tunnel: [w974 w980] -> w915
                            tunnel: w906 -> [w973 w976]
                            tunnel: w903 -> [_ w979]
                            tunnel: w914 -> [_ w978]
                            tunnel: [w973 w975] -> w912
                            frame "Exit" {
                            }
                            frame Default {
                              n350 = call "FileNameGenerator.vi"("Type of scan"=w979, "Case temp"=w977, "Add Axis"=w983, "Current Plane in"=w981, "String in"=w978, "Boolean"=w982, "Case Name in"=w976) -> ("Current Plane out"=w980:i32, "Root Case Name"=w975:string, "Case Name out"=w984:string)  [unwired: 2 in]
                            }
                          }
                          n351 = call "Dual XDCR Scan.vi"("Digitizer Settings In"=w926, "Dual XDCR Mode"=w913, "Motion Settings In"=w909, "Switch Unit"=w923, "Ann Array Params"=w905, "Case Name"=w910, "Scan Parameters  Cluster"=w908, "Dual XDCR Settings"=w896) -> ("Ann Array Params"=w904:T50, "Case Names"=w907:string[], "Digitizer Settings"=w925:T13, "Error Message"=w924:string, "Motion Settings"=w922:T10, "Scan Params Array"=w921:T55[])  [unwired: 5 in, 1 out]
                        }
                        frame "Contrast Agents" {
                          n352 = Bundle By Name(cluster=w991, "Focal Zones"="CA Threshold") -> (w989:T50)
                          n353 = call "FileNameGenerator.vi"("Type of scan"=w999, "Case temp"=w995, "Add Axis"=w1000, "Current Plane in"=w997, "String in"=w993, "Boolean"=w998, "Case Name in"=w1001) -> ("Current Plane out"=w996:i32, "Root Case Name"=w994:string, "Case Name out"=w1002:string)  [unwired: 2 in]
                          n354 = call "Contrast.vi"("Burst Ct"="Burst Ct", "CA Threshold"="CA Threshold", "File Name In"=w1002, "Voltage Steps"="Drive Voltages", "Motion Settings"=w1004, "Digitizer Settings"=w1005) -> ("Scan Params"=w987:T55)  [unwired: 1 in, 4 out]
                          n355 = Build Array(w987) -> (w1003:T55[])
                          n356 = Build Array(w1002) -> (w992:string[])
                        }
                        frame "1-D w/ Real-Time Set Up" {
                          n357 = Unbundle By Name(w1009) -> ("Synth Foc?"=w1010:bool)
                          n358 = case shown="False" w1010 {
                            tunnel: w1022 -> [w1040 w1048]
                            tunnel: [w1039 w1047] -> w1026
                            tunnel: w1025 -> [w1038 w1046]
                            tunnel: [w1037 w1045] -> w1023
                            tunnel: w1012 -> [w1036 w1044]
                            tunnel: [w1035 w1044] -> w1011
                            tunnel: w1009 -> [w1034 w1043]
                            tunnel: [w1033 w1042] -> w1008
                            tunnel: w1007 -> [w1032 _]
                            frame False {
                              n359 = call "RealTimeSingle.vi"("Digitizer Settings"=w1040, "File Name"=w1036, "Motion Settings"=w1038, "Type of scan"=w1032, "Ann Array Params"=w1034, "return to start"=TRUE) -> ("Ann Array Params Out"=w1033:T50, "Digitizer Settings Out"=w1039:T13, "File Name Out"=w1035:string, "Motion Settings Out"=w1037:T10)  [unwired: 7 in, 3 out]
                            }
                            frame True {
                              n360 = call "Real Time_Master.vi"("File Name"=w1044, "Ann Array Params"=w1043, "Motion Settings"=w1046, "Digitizer Settings"=w1048) -> ("Ann Array\nParams Out"=w1042:T50, "Motion Settings Out"=w1045:T10, "Digitizer Settings Out"=w1047:T13)  [unwired: 5 in]
                            }
                          }
                          n361 = call "FileNameGenerator.vi"("Type of scan"=w1007, "Case temp"=w1015, "Add Axis"=w1016, "Current Plane in"=w1019, "String in"=w1018, "Boolean"=w1017, "Case Name in"=w1011) -> ("Current Plane out"=w1020:i32, "Root Case Name"=w1014:string, "Case Name out"=w1021:string)  [unwired: 2 in]
                          n362 = Build Array(w1021) -> (w1013:string[])
                          n363 = call "DigData.vi"("Type of scan"=w1007, "Digitizer Settings"=w1026, "File Name In"=w1021, "Therapy (T)"=w1031, "Ann Array Params"=w1008, "Motion Settings In"=w1023, "recipient"=w1027, "Breath Divide"=w1028) -> ("Scan Params"=w1029:T55, "Error Message"=w1030:string)  [unwired: 7 in, 11 out]
                          n364 = Build Array(w1029) -> (w1024:T55[])
                        }
                      }
                      "Digitzer Error Message" <- w743
                      n365 = property on="Case Name" class="Str"("Value"=w737) -> ()  [unwired: 2 in, 2 out]
                    }
                    frame #3 {
                      # "Update parameters that may have changed. Changs would be in the real time style parts"
                      n366 = Array Size(array=w1049) -> (size(s)=w1051:i32)
                      n367 = case shown="\"Therapy With Scan\", Default" w1052 {
                        tunnel: w1058 -> [w1064 w1067 _]
                        tunnel: w1049 -> [w1063 w1071 w1073]
                        tunnel: [w1062 w1070 w1073] -> w1057
                        tunnel: [w1061 w1066 w1072] -> w1050
                        tunnel: w1051 -> [w1061 w1065 w1072]
                        frame "Therapy With Scan", Default {
                          n368 = Build Array (concatenate)(w1063, w1064) -> (w1062:T55[])
                        }
                        frame "Dual Transducer" {
                          n369 = Array Size(array=w1067) -> (size(s)=w1069:i32)
                          n370 = Decrement(x=w1069) -> (x-1=w1068:i32)
                          n371 = Build Array (concatenate)(w1071, w1067) -> (w1070:T55[])
                          n372 = Add(x=w1068, y=w1065) -> (x+y=w1066:i32)
                        }
                        frame "Real-Time Scan" {
                        }
                      }
                      n373 = local read "distance?"() -> (w1060:bool)
                      n374 = property on="Case to View" class="Ring (strict)"() -> ("Strings []"=w1056:string[])  [unwired: 2 in, 2 out]
                      n375 = property on="distance?" class="Bool (strict)"("Value (Signaling)"=w1060) -> ()  [unwired: 2 in, 2 out]
                      n376 = property on="start scan" class="Bool (strict)"("Value"=FALSE ("start scan")) -> ()  [unwired: 2 in, 2 out]
                      n377 = call "CheckForEmpty.vi"("Strings [] in"=w1056) -> ("Strings [] out"=w1055:string[])  [unwired: 10 in]
                      n378 = Build Array (concatenate)(w1055, w1054) -> (w1053:string[])
                      n379 = property on="Case to View" class="Ring (strict)"("Strings []"=w1053, "Val(Sgnl)"=w1050) -> ()  [unwired: 2 in, 2 out]
                    }
                    frame #4 {
                      # "Update parameters that may have changed. Changs would be in the real time style parts"
                      n380 = Unbundle By Name(w1075) -> ("RT fps"=w1081:sgl, "BKPT Shift"=w1080:i32, "overshoot cts"=w1079:i32, "Distance between\nscan lines (um)"=w1076:sgl, "number of scan planes"=w1078:i32, "Distance between\nscan planes (um)"=w1077:sgl)
                      n381 = flat-sequence {
                        tunnel: w1074 -> [w1083]
                        tunnel: w1076 -> [_]
                        frame #0 {
                          n382 = Unbundle By Name(w1083) -> ("lines per plane"=w1082:i32)
                          n383 = property on="lines per plane" class="DigNum (strict)"("Val(Sgnl)"=w1082) -> ()  [unwired: 2 in, 2 out]
                        }
                      }
                      n384 = property on="Distance between\nscan lines (um)" class="DigNum (strict)"("Value"=w1076) -> ()  [unwired: 2 in, 2 out]
                      n385 = property on="number of planes" class="DigNum (strict)"("Value"=w1078) -> ()  [unwired: 2 in, 2 out]
                      n386 = local write "RT fps"(w1081) -> ()
                      n387 = local write "BKPT Shift"(w1080) -> ()
                      n388 = local write "Overshoot"(w1079) -> ()
                      n389 = property on="Distance between\nplanes (um)" class="DigNum (strict)"("Val(Sgnl)"=w1077) -> ()  [unwired: 2 in, 2 out]
                    }
                    frame #5 {
                      n390 = property on="Microscopy Scan Mode" class="RadioBtnsControl (strict)"() -> ("Value"=w1091:T7)  [unwired: 2 in, 2 out]
                      n391 = property on="Type of scan" class="Enum (strict)"() -> ("Value"=w1090:T21)  [unwired: 2 in, 2 out]
                      n392 = property on="Auto Vz?" class="Bool (strict)"() -> ("Value"=w1085:bool)  [unwired: 2 in, 2 out]
                      n393 = Equal?(x=w1091, y=T7."Detailed Scan") -> (x = y?=w1087:bool)
                      n394 = Equal?(x=w1090, y=ScanType2."Acoustic Microscopy") -> (x = y?=w1086:bool)
                      n395 = Compound Arithmetic op=AND(w1085, w1087, w1086) -> (w1084:bool)
                      n396 = case shown="True" w1084 {
                        frame False {
                        }
                        frame True {
                          n397 = property on="Microscopy\nScan Mode" class="RadioBtnsControl (strict)"("Val(Sgnl)"=T7."V-Z Scan" ("Value (Signaling)")) -> (error out=w1093:errorcluster)  [unwired: 2 in, 1 out]
                          n398 = while {
                            tunnel: [w1115] -> _
                            tunnel: w1093 -> [w1098]
                            tunnel: [w1096] -> w1092
                            stop <- w1097 continue-if-true
                            w1104 = 5.0 ("Time Target (s)")
                            n399 = call "Elapsed Time"("Time Target (s)"=w1104) -> ("Elapsed Time (s)"=w1103:dbl, "Time has Elapsed"=w1107:bool)  [unwired: 11 in, 6 out]
                            n400 = Subtract(x=w1104, y=w1103) -> (x-y=w1102:dbl)
                            n401 = Number To Decimal String(number=w1102) -> (decimal integer string=w1101:string)  [unwired: 1 in]
                            n402 = Concatenate Strings("Vz-Scan will start in " ("Message"), w1101, " seconds" ("string")) -> (w1106:string)
                            n403 = call "Message Popup.vi"("error in"=w1098, "Message"=w1106) -> ("error out"=w1112:errorcluster, "Cancel Button out"=w1096:bool, "OK Button out"=w1099:bool)  [unwired: 7 in]
                            n404 = Compound Arithmetic op=OR(w1107, w1099, w1096) -> (w1100:bool)
                            n405 = Open VI Reference(vi path=path "Message Popup.vi", error in (no error)=w1112) -> (vi reference=w1110:refnum<vi>, error out=w1111:errorcluster)  [unwired: 4 in]
                            n406 = Not(x=w1100) -> (.not. x?=w1097:bool)
                            n407 = property class="VI"(reference=w1110, error in=w1111, "Front Panel.Open"=w1097, "Front Panel.IsFrontmost"=w1097) -> (reference out=w1108:refnum<vi>, error out=w1109:errorcluster)
                            n408 = Close Reference(reference=w1108, error in (no error)=w1109) -> (error out=w1115:errorcluster)
                          }
                          n409 = case shown="False" w1092 {
                            frame False {
                              n410 = property on="start scan" class="Bool (strict)"("Val(Sgnl)"=TRUE ("Value (Signaling)")) -> ()  [unwired: 2 in, 2 out]
                            }
                            frame True {
                            }
                          }
                        }
                      }
                    }
                  }
                  n411 = Unbundle By Name(w634) -> ("Switch T/R"=w633:i16)
                  n412 = property on="Transducer" class="DigNum (strict)"("Value"=w633) -> ()  [unwired: 2 in, 2 out]
                }
                event "Parameter Selection": Value Change {
                  n413 = event-data() -> ()  [unwired: 7 out]
                  n414 = property on="Scan data" class="Clust (strict)"() -> ("Value"=w1117:T1)  [unwired: 2 in, 2 out]
                  n415 = property on="Pressure Cal Parameters" class="Clust (strict)"() -> ("Value"=w1120:T2)  [unwired: 2 in, 2 out]
                  n416 = Unbundle By Name(w1117) -> ("scan data"=w1119:dbl[][][])
                  n417 = call "CalcPulsePrams.vi"("Digitizer Settings"=w1118, "Array"=w1119, "Pressure Cal Parameters"=w1120) -> ("Data"=w1121:T58)  [unwired: 8 in]
                  n418 = Bundle By Name(cluster=w1117, "Pulse Parameters"=w1121) -> (w1116:T1)
                  n419 = call "ChoosePram.vi"("Parameter Selection"="Parameter Selection", "Scan data"=w1116) -> ("data out"=w1124:dbl[][])  [unwired: 2 in, 7 out]
                  n420 = case shown="\"2-D\"" "Plot" {
                    tunnel: w1116 -> [w1135 w1141]
                    tunnel: w1124 -> [w1134 w1137]
                    frame "1-D", Default {
                      n421 = Unbundle By Name(w1135) -> ("axis1o"=w1131:dbl, "step size"=w1130:dbl)
                      n422 = Index Array(array=w1134, index (col)=0 ("Index")) -> (element=w1136:dbl[])  [unwired: 1 in]
                      n423 = Bundle("axis1o"=w1131, "step size"=w1130, "data out"=w1136) -> (→"Hydrophopne Waveform Graph":T4)  [unwired: 1 out]
                    }
                    frame "2-D" {
                      n424 = Unbundle By Name(w1141) -> ("axis 1 ticks"=w1139:dbl[], "axis 2 ticks"=w1138:dbl[])
                      n425 = call <vilib>:"3D Surface.vi"("z matrix"=w1137, "y vector"=w1138, "x vector"=w1139, "3D graph"="3D Surface") -> ()  [unwired: 1 in, 7 out]
                    }
                  }
                }
                event "Fix Z Delay?": Value Change {
                  n426 = event-data() -> ("NewVal"=w1144:bool)  [unwired: 1 out]
                  n427 = Bundle By Name(cluster=w1143, "Fix Z Delay?"=w1144) -> (w1142:T13)
                }
                event "Rot lines per plane", "Pre-Looks", "Distance between\nscan lines (um)", "lines per plane": Value Change {
                  # "Update scan propeties"
                  # "Make sure prf case updates"
                  # "This is micrometers"
                  n428 = event-data() -> ()  [unwired: 2 out]
                  n429 = Unbundle By Name(w1154) -> ("Avg Num"=w1153:i32)
                  n430 = case shown="\"Acoustic Microscopy\"" w1182 {
                    tunnel: [w1205 w1208 w1223 w1230] -> _
                    tunnel: "lines per plane" -> [w1205 _ w1221 _]
                    tunnel: [TRUE TRUE TRUE w1229] -> w1172
                    tunnel: [w1204 w1210 w1220 w1231] -> w1157
                    tunnel: "Distance between\nscan lines (um)" -> [w1204 w1210 w1220 _]
                    tunnel: w1181 -> [_ _ _ w1227]
                    tunnel: [w1205 w1208 w1221 w1230] -> w1176
                    tunnel: [w1203 w1214 w1217 w1228] -> w1174
                    tunnel: w1154 -> [w1203 w1214 w1218 w1228]
                    frame "Therapy With Scan", Default {
                    }
                    frame "Acoustic Microscopy" {
                      n431 = To Double Precision Float(number=w1210) -> (double precision float=w1211:dbl)
                      n432 = property on="Length of\none plane (mm)" class="DigNum (strict)"() -> ("Value"=w1209:dbl)  [unwired: 2 in, 2 out]
                      n433 = expression code="x*1e-3"(w1211) -> (w1212:dbl)
                      n434 = Divide(x=w1209, y=w1212) -> (x/y=w1213:dbl)
                      n435 = Round To Nearest(number=w1213) -> (nearest integer value=w1207:dbl)
                      n436 = call "Force Odd or Even.vi"("input"=w1207) -> ("output"=w1208:i32)  [unwired: 1 in]
                      n437 = property on="lines per plane" class="DigNum (strict)"("Value"=w1208) -> ()  [unwired: 2 in, 2 out]
                    }
                    frame "M Scan With Therapy Burst" {
                      # "Account for pre-look lines that get thrown out when computing total points captured. Default is up to 50 pre-looks before extra data is deleted."
                      n438 = global read "PulserGlobals.vi" "Divide prf by"() -> (w1216:i32)
                      n439 = Less?(x=w1216, y="Pre-Looks") -> (x < y?=w1226:bool)
                      n440 = Bundle By Name(cluster=w1218, "Pre-Looks"="Pre-Looks") -> (w1217:T13)
                      n441 = Subtract(x=w1216, y="Pre-Looks") -> (x-y=w1225:i32)
                      n442 = Add(x=w1221, y=w1225) -> (x+y=w1224:i32)
                      n443 = Select(t=w1221, s=w1226, f=w1224) -> (s? t:f=w1223:i32)
                    }
                    frame "Rotational Scan" {
                      n444 = call "RotStageParams.vi"("Rot lines per plane"="Rot lines per plane", "Sector Angle"=w1227) -> ("Valid combo"=w1229:bool, "Number of scan lines"=w1230:i32, "distance between scans"=w1231:i32)
                    }
                  }
                  n445 = local read "Bulk Acq"() -> (w1173:bool)
                  n446 = Bundle By Name(cluster=w1151, "scan pair"="scan pair") -> (w1150:T10)
                  n447 = property on="Bulk Acq" class="Bool (strict)"("Val(Sgnl)"=w1173) -> ()  [unwired: 2 in, 2 out]
                  n448 = local read "prf (kHz)"() -> (w1179:dbl)
                  n449 = Decrement(x=w1176) -> (x-1=w1156:i32)
                  n450 = property on="prf (kHz)" class="DigNum (strict)"("Val(Sgnl)"=w1179) -> ()  [unwired: 2 in, 2 out]
                  n451 = Bundle By Name(cluster=w1174, "lines per plane"=w1176) -> (w1171:T13)
                  n452 = Multiply(x=w1157, y=w1156) -> (x*y=w1185:sgl)
                  n453 = Divide(x=w1185, y=1000 ("x")) -> (x/y=w1165:sgl)
                  n454 = Select(t=1, s=w1180, f=w1185) -> (s? t:f=w1158:sgl)
                  n455 = case shown="1" w1153 {
                    tunnel: w1150 -> [w1190 w1197 w1202]
                    tunnel: w1158 -> [w1194 w1200 _]
                    tunnel: w1157 -> [w1192 w1199 _]
                    tunnel: [w1191 w1201 w1202] -> w1155
                    frame 0, Default {
                      n456 = call "OvershootCalc.vi"("Motion Settings In in"=w1190, "Num of trigs to overshoot (2.5)"=sgl 2.0 ("value"), "Distance between\nscan lines (um)"=w1192, "rmax overshoot"=sgl 200.0, "Total Length of Scan (mm)"=w1194) -> ("Overshoot Count"=w1195:sgl, "Motion Settings out"=w1191:T10)  [unwired: 2 out]
                      n457 = property on="Overshoot" class="DigNum (strict)"("Value"=w1195) -> ()  [unwired: 2 in, 2 out]
                    }
                    frame 1 {
                      n458 = Unbundle By Name(w1197) -> ("overshoot cts"=w1196:i32)
                      n459 = call "OvershootCalc.vi"("Motion Settings In in"=w1197, "Num of trigs to overshoot (2.5)"=sgl 0.0, "Distance between\nscan lines (um)"=w1199, "rmax overshoot"=w1196, "Total Length of Scan (mm)"=w1200) -> ("Motion Settings out"=w1201:T10)  [unwired: 3 out]
                    }
                    frame -1 {
                    }
                  }
                  n460 = property on="Length of\none plane (mm)" class="DigNum (strict)"("Value"=w1165) -> ()  [unwired: 2 in, 2 out]
                  n461 = local read "Multi Trig"() -> (w1178:bool)
                  n462 = call "CheckTotalSamples.vi"("Digitizer Settings"=w1171, "Multi Trig"=w1178, "Multi Trig#"="Multi Trig#", "Valid combo"=w1172, "Bulk Acq"=w1173) -> ("Total Pts"=→"Total Pts":bool)  [unwired: 10 in]
                  n463 = call "GetScanAxis.vi"("scan pair"="scan pair") -> ("Axis 1"=w1161:i32, "Axis 2"=w1160:i32, "Axis 3"=w1159:i32)  [unwired: 1 in]
                  n464 = local read "Transducer"() -> (w1169:u32)
                  n465 = Build Array(w1161, w1160) -> (w1164:i32[])
                  n466 = Decrement(x=w1164) -> (x-1=w1163:i32[])
                  n467 = property on="3rd Axis" class="Ring (strict)"("Value"=w1159, "Disabled Items []"=w1163) -> ()  [unwired: 2 in, 2 out]
                  n468 = call "UpdateDualXDCRSettings.vi"("Digitizer Settings in"=w1171, "Motion Settings in"=w1155, "Switch T/R"=w1169, "Dual XDCR Settings In"=w1167, "Switch Unit"=w1170) -> ("Dual XDCR Settings"=w1168:T24)  [unwired: 3 in]
                }
                event "Distance between\nplanes (um)": Value Change {
                  n469 = event-data() -> ()  [unwired: 5 out]
                  n470 = property on="Attenuation Scan" class="Bool (strict)"() -> ("Value"=w1234:bool)  [unwired: 2 in, 2 out]
                  n471 = case shown="True" w1234 {
                    tunnel: "Distance between\nplanes (um)" -> [_ w1248]
                    frame False {
                    }
                    frame True {
                      n472 = property on="Distance between\nZ planes (um)" class="DigNum (strict)"("Value"=w1248) -> ()  [unwired: 2 in, 2 out]
                    }
                  }
                  n473 = case shown="\"Acoustic Microscopy\"" w1236 {
                    tunnel: "Distance between\nplanes (um)" -> [w1252 w1259]
                    tunnel: "number of planes" -> [_ w1257]
                    tunnel: [w1249 w1257] -> w1235
                    frame "Acoustic Microscopy" {
                      n474 = To Double Precision Float(number=w1252) -> (double precision float=w1254:dbl)
                      n475 = expression code="x*1e-3"(w1254) -> (w1255:dbl)
                      n476 = property on="Length of\nall planes (mm)" class="DigNum (strict)"() -> ("Value"=w1251:dbl)  [unwired: 2 in, 2 out]
                      n477 = Divide(x=w1251, y=w1255) -> (x/y=w1256:dbl)
                      n478 = Round To Nearest(number=w1256) -> (nearest integer value=w1253:dbl)
                      n479 = Increment(x=w1253) -> (x+1=w1250:dbl)
                      n480 = call "Force Odd or Even.vi"("input"=w1250) -> ("output"=w1249:i32)  [unwired: 1 in]
                      n481 = property on="number of planes" class="DigNum (strict)"("Value"=w1249) -> ()  [unwired: 2 in, 2 out]
                    }
                    frame "M scan", Default {
                      n482 = Decrement(x=w1257) -> (x-1=w1261:u16)
                      n483 = Multiply(x=w1261, y=w1259) -> (x*y=w1260:sgl)
                      n484 = Divide(x=w1260, y=1000 ("x")) -> (x/y=w1258:sgl)
                      n485 = property on="Length of\nall planes (mm)" class="DigNum (strict)"("Value"=w1258) -> ()  [unwired: 2 in, 2 out]
                    }
                  }
                  n486 = local read "Transducer"() -> (w1243:u32)
                  n487 = Bundle By Name(cluster=w1245, "Distance between\nscan planes (um)"="Distance between\nplanes (um)", "number of scan planes"=w1235) -> (w1242:T10)
                  n488 = call "UpdateDualXDCRSettings.vi"("Digitizer Settings in"=w1241, "Motion Settings in"=w1242, "Switch T/R"=w1243, "Dual XDCR Settings In"=w1239, "Switch Unit"=w1240) -> ("Dual XDCR Settings"=w1238:T24)  [unwired: 3 in]
                }
                event "number of planes": Value Change {
                  n489 = event-data() -> ()  [unwired: 5 out]
                  n490 = property on="Microscopy Scan Mode" class="RadioBtnsControl (strict)"() -> ("Value"=w1269:T7)  [unwired: 2 in, 2 out]
                  n491 = property on="Type of scan" class="Enum (strict)"() -> ("Value"=w1266:T21)  [unwired: 2 in, 2 out]
                  n492 = property on="number of planes" class="DigNum (strict)"() -> ("Value"=w1270:u16)  [unwired: 2 in, 2 out]
                  n493 = Equal?(x=w1269, y=T7."Overview Scan") -> (x = y?=w1268:bool)
                  n494 = Equal?(x=w1266, y=ScanType2."Acoustic Microscopy") -> (x = y?=w1265:bool)
                  n495 = And(x=w1268, y=w1265) -> (x .and. y?=w1263:bool)
                  n496 = case shown="True" w1263 {
                    tunnel: [w1283 w1288] -> w1271
                    tunnel: w1270 -> [w1282 w1293]
                    frame False {
                      n497 = property on="Distance between\nplanes (um)" class="DigNum (strict)"() -> ("Value"=w1283:sgl)  [unwired: 2 in, 2 out]
                      n498 = Decrement(x=w1282) -> (x-1=w1286:u16)
                      n499 = Multiply(x=w1286, y=w1283) -> (x*y=w1285:sgl)
                      n500 = Divide(x=w1285, y=1000 ("x")) -> (x/y=w1284:sgl)
                      n501 = property on="Length of\nall planes (mm)" class="DigNum (strict)"("Value"=w1284) -> ()  [unwired: 2 in, 2 out]
                    }
                    frame True {
                      n502 = property on="Length of\nall planes (mm)" class="DigNum (strict)"() -> ("Value"=w1292:dbl)  [unwired: 2 in, 2 out]
                      n503 = Decrement(x=w1293) -> (x-1=w1289:u16)
                      n504 = Multiply(x=w1292, y=1000 ("x")) -> (x*y=w1290:dbl)
                      n505 = Divide(x=w1290, y=w1289) -> (x/y=w1288:dbl)
                      n506 = property on="Distance between\nplanes (um)" class="DigNum (strict)"("Value"=w1288) -> ()  [unwired: 2 in, 2 out]
                    }
                  }
                  n507 = local read "Transducer"() -> (w1278:u32)
                  n508 = Bundle By Name(cluster=w1279, "Distance between\nscan planes (um)"=w1271, "number of scan planes"=w1270) -> (w1277:T10)
                  n509 = call "UpdateDualXDCRSettings.vi"("Digitizer Settings in"=w1276, "Motion Settings in"=w1277, "Switch T/R"=w1278, "Dual XDCR Settings In"=w1274, "Switch Unit"=w1275) -> ("Dual XDCR Settings"=w1273:T24)  [unwired: 3 in]
                }
                event "Length of\none plane (mm)", "Length of\nall planes (mm)": Value Change {
                  n510 = event-data() -> ()  [unwired: 5 out]
                  n511 = property on="Microscopy Scan Mode" class="RadioBtnsControl (strict)"() -> ("Value"=w1305:T7)  [unwired: 2 in, 2 out]
                  n512 = property on="Type of scan" class="Enum (strict)"() -> ("Value"=w1301:T21)  [unwired: 2 in, 2 out]
                  n513 = Equal?(x=w1305, y=T7."Overview Scan") -> (x = y?=w1304:bool)
                  n514 = Equal?(x=w1301, y=ScanType2."Acoustic Microscopy") -> (x = y?=w1300:bool)
                  n515 = property on="Attenuation Scan" class="Bool (strict)"() -> ("Value"=w1295:bool)  [unwired: 2 in, 2 out]
                  n516 = And(x=w1304, y=w1300) -> (x .and. y?=w1302:bool)
                  n517 = case shown="True" w1302 {
                    tunnel: "Length of\nall planes (mm)" -> [w1321 w1328]
                    frame False {
                      n518 = property on="Distance between\nplanes (um)" class="DigNum (strict)"() -> ("Value"=w1320:sgl)  [unwired: 2 in, 2 out]
                      n519 = To Double Precision Float(number=w1320) -> (double precision float=w1318:dbl)
                      n520 = expression code="x*1e-3"(w1318) -> (w1319:dbl)
                      n521 = Divide(x=w1321, y=w1319) -> (x/y=w1322:dbl)
                      n522 = Round To Nearest(number=w1322) -> (nearest integer value=w1323:dbl)
                      n523 = Increment(x=w1323) -> (x+1=w1317:dbl)
                      n524 = call "Force Odd or Even.vi"("input"=w1317) -> ("output"=w1316:i32)  [unwired: 1 in]
                      n525 = property on="number of planes" class="DigNum (strict)"("Val(Sgnl)"=w1316) -> ()  [unwired: 2 in, 2 out]
                    }
                    frame True {
                      n526 = property on="number of planes" class="DigNum (strict)"() -> ("Value"=w1324:u16)  [unwired: 2 in, 2 out]
                      n527 = To Double Precision Float(number=w1328) -> (double precision float=w1329:dbl)
                      n528 = expression code="x*1e3"(w1329) -> (w1327:dbl)
                      n529 = Decrement(x=w1324) -> (x-1=w1326:u16)
                      n530 = Divide(x=w1327, y=w1326) -> (x/y=w1325:dbl)
                      n531 = property on="Distance between\nplanes (um)" class="DigNum (strict)"("Val(Sgnl)"=w1325) -> ()  [unwired: 2 in, 2 out]
                    }
                  }
                  n532 = property on="Distance between\nscan lines (um)" class="DigNum (strict)"() -> ("Value"=w1306:sgl)  [unwired: 2 in, 2 out]
                  n533 = case shown="True" w1295 {
                    tunnel: "Length of\nall planes (mm)" -> [_ w1315]
                    frame False {
                    }
                    frame True {
                      n534 = property on="Length of Z \nScan (mm)" class="DigNum (strict)"("Val(Sgnl)"=w1315) -> ()  [unwired: 2 in, 2 out]
                    }
                  }
                  n535 = expression code="x*1e-3"(w1306) -> (w1307:sgl)
                  n536 = Divide(x="Length of\none plane (mm)", y=w1307) -> (x/y=w1309:dbl)
                  n537 = Round To Nearest(number=w1309) -> (nearest integer value=w1298:dbl)
                  n538 = call "Force Odd or Even.vi"("input"=w1298) -> ("output"=w1297:i32)  [unwired: 1 in]
                  n539 = property on="lines per plane" class="DigNum (strict)"("Val(Sgnl)"=w1297) -> ()  [unwired: 2 in, 2 out]
                }
                event "Xtra plane\ndistance  (um)", "Xtra planes": Value Change {
                  n540 = event-data() -> ()  [unwired: 6 out]
                  n541 = Decrement(x="Xtra planes") -> (x-1=w1340:i32)
                  n542 = Compound Arithmetic op=MULTIPLY(w1340, "Xtra plane\ndistance  (um)", sgl 0.001 ("value")) -> (→"Cross plane\nlength (mm)":sgl)
                  n543 = Bundle By Name(cluster=w1336, "Xtra planes"="Xtra planes", "Xtra plane\ndistance  (um)"="Xtra plane\ndistance  (um)") -> (w1335:T10)
                }
                event "SetDig": Value Change {
                  # "Need to use DC 1 M Ohm\nfor ttl pulses coming from switch box.\nFor some reason"
                  n544 = event-data() -> ()  [unwired: 3 out]
                  n545 = flat-sequence {
                    tunnel: w1363 -> [w1376]
                    tunnel: w1362 -> [w1375]
                    tunnel: w1359 -> [w1374]
                    tunnel: w1357 -> [w1370]
                    tunnel: [w1373] -> w1346
                    tunnel: w1352 -> [w1372]
                    tunnel: [w1371] -> w1355
                    tunnel: w1349 -> [w1368]
                    tunnel: [w1367] -> w1348
                    tunnel: [w1367] -> w1347
                    tunnel: [w1366] -> w1344
                    tunnel: w1343 -> [w1365]
                    tunnel: w1342 -> [w1364]
                    tunnel: w1355 -> [w1405]
                    tunnel: [w1402] -> w1356
                    tunnel: [w1400] -> w1354
                    tunnel: w1347 -> [w1404]
                    tunnel: w1344 -> [w1400]
                    frame #0 {
                      n546 = Unbundle By Name(w1370) -> ("Main Digitizer"=w1369:T14)
                      n547 = case shown="\"Acqiris Digitizer\", Default" w1369 {
                        tunnel: w1376 -> [w1387 _ _]
                        tunnel: w1375 -> [w1386 w1395 _]
                        tunnel: w1374 -> [_ _ _]
                        tunnel: w1370 -> [w1385 w1394 w1398]
                        tunnel: [w1383 w1393 w1398] -> w1373
                        tunnel: w1372 -> [w1384 w1392 w1399]
                        tunnel: [w1381 w1391 w1399] -> w1371
                        tunnel: w1368 -> [w1382 w1389 w1397]
                        tunnel: [w1380 w1388 w1397] -> w1367
                        tunnel: [w1379 w1390 w1396] -> w1366
                        tunnel: w1365 -> [w1378 w1390 w1396]
                        tunnel: w1364 -> [w1377 _ _]
                        frame "Acqiris Digitizer", Default {
                          n548 = call "SetUpDigi.vi"("Digitizer Settings"=w1385, "Motion Settings In"=w1384, "Ann Array Params"=w1382, "Type of scan"=w1377, "Therapy VISA session"=w1387, "Therapy (T)"=w1386, "Dual XDCR Settings"=w1378) -> ("Dual XDCR Settings Out"=w1379:T24, "Digitizer Settings Out"=w1383:T13, "Motion Settings Out"=w1381:T10, "Ann Array Params out"=w1380:T50)  [unwired: 6 in, 3 out]
                        }
                        frame "LeCroy" {
                          n549 = call "SetUpLeCroy.vi"("Therapy (T)"=w1395, "Ann Array Params"=w1389, "Motion Settings In"=w1392, "Digitizer Settings"=w1394) -> ("Motion Settings Out"=w1391:T10, "Ann Array Params out"=w1388:T50, "Digitizer Settings Out"=w1393:T13)  [unwired: 3 in, 2 out]
                        }
                        frame "No Digitizer" {
                        }
                      }
                    }
                    frame #1 {
                      n550 = Unbundle By Name(w1404) -> ("Switch T/R"=w1403:i16)
                      n551 = call "FindLocation.vi"("Motion Settings"=w1405) -> ("Motion Settings Out"=w1402:T10)  [unwired: 2 in, 3 out]
                      n552 = Unbundle By Name(w1402) -> ("Distance between\nscan lines (um)"=w1401:sgl)
                      n553 = local read "CTR PRF?"() -> (w1406:bool)
                      n554 = property on="Distance between\nscan lines (um)" class="DigNum (strict)"("Val(Sgnl)"=w1401) -> ()  [unwired: 2 in, 2 out]
                      n555 = local write "Transducer"(w1403) -> ()
                      n556 = property on="CTR PRF?" class="Bool (strict)"("Val(Sgnl)"=w1406) -> ()  [unwired: 2 in, 2 out]
                    }
                  }
                  n557 = call "MotionProfileChange.vi"("Motion Mode"=enum16{"Move Mode", "Scan Mode"}."Move Mode", "Location"=w1351, "Motion Settings In in"=w1353) -> ("Motion Settings In out"=w1352:T10)  [unwired: 8 in]
                  n558 = Unbundle By Name(w1346) -> ("lines per plane"=w1345:i32)
                  n559 = local write "SetDig"(FALSE ("SetDig")) -> ()
                  n560 = property on="lines per plane" class="DigNum (strict)"("Val(Sgnl)"=w1345) -> ()  [unwired: 2 in, 2 out]
                }
                event "Take Webcam pic": Value Change {
                  n561 = event-data() -> ()  [unwired: 4 out]
                  n562 = property on="Take Webcam pic" class="Bool (strict)"("Value"=FALSE ("Take Webcam pic")) -> ()  [unwired: 2 in, 2 out]
                  n563 = call "LymphNodeSimpleSnap.vi"() -> ()  [unwired: 12 in]
                }
                event "Sub Ap Excite?": Value Change {
                  n564 = event-data() -> ("NewVal"=w1414:bool)  [unwired: 2 out]
                  n565 = Bundle By Name(cluster=w1416, "Sub Ap Excite?"=w1414) -> (w1415:T50)
                }
                event "Transfer to FTP": Value Change {
                  n566 = event-data() -> ()  [unwired: 7 out]
                  n567 = global read "MotionGlobals.vi" "Root Save Path"() -> (w1425:path)
                  n568 = Move(source path=w1425, 10:path "ftp:/ftp.rri-usa.org/biomed/suny/Data" ("target path (use dialog)")) -> ()  [unwired: 3 in, 3 out]
                }
                event "Case to View", "Scan to View", "CH2?", "Filter Prams", "Transpose": Value Change {
                  # "view data selected case and scan number. If case is saved, choose header specs and then save data in .eye files. For 2-D scan, need to modify file name before saving."
                  # "Display plot"
                  # "Display file if new scan to view"
                  n569 = event-data() -> ()  [unwired: 2 out]
                  n570 = Unbundle By Name(w1443) -> ("Add Axis"=w1441:bool, "number of scan planes"=w1442:i32)
                  n571 = Unbundle By Name(w1434) -> ("Full Array Scan?"=w1433:bool)
                  n572 = Unbundle By Name(w1437) -> ("Dig Config"=w1444:T15, "Total Dig CH"=w1435:i32)
                  n573 = local read "Case to View"() -> (w1465:u16)
                  n574 = Index Array(array=w1467, index=w1465) -> (element=w1460:T55)
                  n575 = Unbundle By Name(w1460) -> ("File Name"=w1451:string, "Keep?"=w1468:bool, "Synth Foc?"=w1452:bool)
                  n576 = case shown="False" "CH2?" {
                    tunnel: w1451 -> [w1472 w1474]
                    tunnel: [w1472 w1473] -> w1450
                    frame False {
                    }
                    frame True {
                      n577 = Concatenate Strings("CH2", w1474) -> (w1473:string)
                    }
                  }
                  n578 = local write "Keep?"(w1468) -> ()
                  n579 = call "ScanNumToFilePath.vi"("# Elements"=w1435, "Additional Axis?"=w1441, "Dig Config"=w1444, "Full Array Scan?"=w1433, "Scan to View"="Scan to View", "number of scan planes"=w1442, "Synth App?"=w1452, "Root File Name"=w1450) -> ("error out"=w1455:errorcluster, "appended path"=w1448:path)  [unwired: 1 in, 1 out]
                  "View path" <- w1448
                  n580 = property on="distance?" class="Bool (strict)"("Value (Signaling)"="distance?") -> ()  [unwired: 2 in, 2 out]
                  n581 = case shown="No Error" w1455 {
                    tunnel: [w1478 _] -> w1456
                    tunnel: w1448 -> [w1477 _]
                    tunnel: [w1476 _] -> w1440
                    frame No Error {
                      n582 = call "ReadEyeFileFast.vi"("new file path"=w1477) -> ("2-D data array"=w1478:sgl[][], "Header In"=w1476:T59)  [unwired: 2 in, 15 out]
                    }
                    frame Error {
                    }
                  }
                  n583 = Strip Path(path=w1448) -> (name=→"File":string)  [unwired: 1 out]
                  n584 = Unbundle By Name(w1440) -> ("A/D info.# A/D bits"=w1430:i16, "A/D info.sample rate MHz"=w1439:u16)
                  n585 = call "SubMean.vi"("Bit Depth"=w1430, "Scan Data In"=w1456, "Samp Rate (MHz)"=w1439, "Filter Prams"="Filter Prams", "Type of Mean"="Type of Mean") -> ("Array"=w1458:dbl[][], "Filter Params"=w1436:T17)  [unwired: 1 in, 1 out]
                  n586 = global write "MotionGlobals.vi" "Filter Prams"(w1436) -> ()
                  n587 = property on="Filter Prams" class="Clust (strict)"("Value"=w1436) -> ()  [unwired: 2 in, 2 out]
                  n588 = case shown="True" "Compress" {
                    tunnel: w1458 -> [w1480 w1487]
                    tunnel: [w1480 w1483] -> w1454
                    tunnel: w1437 -> [_ w1482]
                    tunnel: w1440 -> [_ _]
                    tunnel: [w1479 w1481] -> w1431
                    tunnel: w1430 -> [w1479 _]
                    frame False {
                    }
                    frame True {
                      w1481 = 16
                      n589 = call "ChirpComp.vi"("Digitizer Settings"=w1482, "Data In"=w1487) -> ("Data Out"=w1486:dbl[][])  [unwired: 9 out]
                      n590 = call-poly <vilib>:"Quick Scale.vi"("X"=w1486) -> ("Yij=Xij/Max|X|"=w1485:dbl[][])  [unwired: 2 out]
                      n591 = expression code="2.0**(x-1)"(w1481) -> (w1484:i32)
                      n592 = Multiply(x=w1485, y=w1484) -> (x*y=w1483:dbl[][])
                    }
                  }
                  n593 = case shown="True" w1452 {
                    tunnel: w1456 -> [_ w1491]
                    frame False {
                    }
                    frame True {
                      n594 = for {
                        tunnel: w1491 -> [w1495] mode=indexing
                        tunnel: [w1494] -> w1492 mode=indexing
                        n595 = Absolute Value(x=w1495) -> (abs(x)=w1493:sgl[])
                        n596 = Array Max & Min(array=w1493) -> (max value=w1494:sgl)  [unwired: 3 out]
                      }
                      "Waveform Graph" <- w1492
                    }
                  }
                  n597 = case shown="True" "Auto\nScale" {
                    tunnel: w1431 -> [_ w1489]
                    tunnel: "Display mode" -> [_ w1488]
                    frame False {
                    }
                    frame True {
                      n598 = call "SetScale.vi"("# A/D bits"=w1489, "Display mode"=w1488) -> ("Array"=w1490:cluster{dbl, u32}[])
                      n599 = property on="Raw data" class="IntGraph (strict)"("Z Scale.Marker Values[]"=w1490) -> ()  [unwired: 2 in, 2 out]
                    }
                  }
                  n600 = case shown="\"Log Grey Scale\"" "Display mode" {
                    tunnel: w1454 -> [w1497 w1500 w1501 w1504]
                    tunnel: [w1496 w1499 w1501 w1503] -> w1463
                    tunnel: w1431 -> [_ w1498 _ w1502]
                    frame "Linear Abs Grey", Default {
                      n601 = Absolute Value(x=w1497) -> (abs(x)=w1496:dbl[][])
                    }
                    frame "Log Grey Scale" {
                      n602 = call "LogScaleImage.vi"("A/D bits"=w1498, "input array"=w1500) -> ("log scale image"=w1499:dbl[][])  [unwired: 1 out]
                    }
                    frame "Linear Color Scale" {
                    }
                    frame "dB Scale" {
                      n603 = call "dBScale.vi"("Bit Depth"=w1502, "Data In"=w1504) -> ("Data Out"=w1503:dbl[][])  [unwired: 3 in]
                    }
                  }
                  n604 = case shown="False" "Transpose" {
                    tunnel: w1463 -> [w1470 w1471]
                    tunnel: [w1469 w1471] -> w1453
                    frame False {
                      n605 = Transpose 2D Array(2D array=w1470) -> (transposed array=w1469:dbl[][])
                    }
                    frame True {
                    }
                  }
                  "Raw data" <- w1453
                }
                event "Flip X": Value Change {
                  n606 = event-data() -> ()  [unwired: 4 out]
                  n607 = property on="Raw data" class="IntGraph (strict)"("XScale.Flipped"="Flip X") -> ()  [unwired: 2 in, 2 out]
                }
                event "Flip Y": Value Change {
                  n608 = event-data() -> ()  [unwired: 4 out]
                  n609 = property on="Raw data" class="IntGraph (strict)"("YScale.Flipped"="Flip Y") -> ()  [unwired: 2 in, 2 out]
                }
                event "1-to-1": Value Change {
                  n610 = event-data() -> ()  [unwired: 7 out]
                  n611 = stacked-sequence {
                    tunnel: w1520 -> [_ w1533]
                    tunnel: w1519 -> [w1528 _]
                    frame #0 {
                      w1529 = u8 1 ("Y Scale.Scale Fit")
                      n612 = property on="distance?" class="Bool (strict)"() -> ("Value"=w1526:bool)  [unwired: 2 in, 2 out]
                      n613 = case shown="False" w1526 {
                        tunnel: [w1532 _] -> w1527
                        frame False {
                          n614 = Wait (ms)(milliseconds to wait=u32 25) -> ()  [unwired: 1 out]
                          n615 = property on="distance?" class="Bool (strict)"("Val(Sgnl)"=TRUE ("Value (Signaling)")) -> (error out=w1532:errorcluster)  [unwired: 2 in, 1 out]
                        }
                        frame True {
                        }
                      }
                      n616 = property on="Raw data" class="IntGraph (strict)"(error in=w1527, "Plot Bounds"=w1528, "YScale.ScaleFit"=w1529, "XScale.ScaleFit"=w1529) -> ()  [unwired: 1 in, 2 out]
                    }
                    frame #1 {
                      n617 = Unbundle By Name(w1533) -> ("lines per plane"=w1538:i32, "rf points per line"=w1537:i32)
                      n618 = property on="Raw data" class="IntGraph (strict)"() -> ("X Scale.Offset and Multiplier:Multiplier"=w1553:dbl, "Y Scale.Offset and Multiplier:Multiplier"=w1552:dbl, "Plot Bounds"=w1541:T23, "Plot Area Size"=w1540:T60)  [unwired: 2 in, 2 out]
                      n619 = property on="Transpose" class="Bool (strict)"() -> ("Value"=w1539:bool)  [unwired: 2 in, 2 out]
                      n620 = Not(x=w1539) -> (.not. x?=w1534:bool)
                      n621 = Swap Values(12:w1538, 13:w1534, 14:w1537) -> (1:w1536:i32, 3:w1535:i32)
                      n622 = Multiply(x=w1536, y=w1553) -> (x*y=w1551:dbl)
                      n623 = Multiply(x=w1552, y=w1535) -> (x*y=w1550:dbl)
                      n624 = Unbundle(w1540) -> ("Width"=w1545:u32, "Height"=w1543:u32)
                      n625 = Divide(x=w1545, y=w1551) -> (x/y=w1549:dbl)
                      n626 = Divide(x=w1543, y=w1550) -> (x/y=w1548:dbl)
                      n627 = Divide(x=w1549, y=w1548) -> (x/y=w1544:dbl)
                      n628 = Greater?(x=w1544, y=1.0) -> (0:w1547:bool)
                      n629 = case shown="True" w1547 {
                        tunnel: w1545 -> [_ w1567]
                        tunnel: w1544 -> [w1560 w1566]
                        tunnel: w1543 -> [w1559 _]
                        tunnel: w1541 -> [w1554 w1565]
                        tunnel: [w1555 w1561] -> w1542
                        frame False {
                          n630 = Unbundle By Name(w1554) -> ("Top"=w1558:i16)
                          n631 = Multiply(x=w1559, y=w1560) -> (x*y=w1556:dbl)
                          n632 = Add(x=w1558, y=w1556) -> (x+y=w1557:dbl)
                          n633 = Bundle By Name(cluster=w1554, "Bottom"=w1557) -> (w1555:T23)
                        }
                        frame True {
                          n634 = Unbundle By Name(w1565) -> ("Left"=w1563:i16)
                          n635 = Divide(x=w1567, y=w1566) -> (x/y=w1564:dbl)
                          n636 = Add(x=w1563, y=w1564) -> (x+y=w1562:dbl)
                          n637 = Bundle By Name(cluster=w1565, "Right"=w1562) -> (w1561:T23)
                        }
                      }
                      n638 = property on="Raw data" class="IntGraph (strict)"("Plot Bounds"=w1542) -> ()  [unwired: 2 in, 2 out]
                    }
                  }
                }
                event "Fill": Value Change {
                  n639 = event-data() -> ()  [unwired: 7 out]
                  n640 = property on="Raw data" class="IntGraph (strict)"("Plot Bounds"=w1568) -> ()  [unwired: 2 in, 2 out]
                }
                event "distance?": Value Change {
                  n641 = event-data() -> ("NewVal"=w1600:bool)  [unwired: 1 out]
                  n642 = local read "View path"() -> (w1596:path)
                  n643 = File/Directory Info(path=w1596) -> (path out=w1595:path, error out=w1593:errorcluster)  [unwired: 1 in, 5 out]
                  n644 = case shown="No Error" w1593 {
                    tunnel: w1595 -> [w1609 _]
                    tunnel: [w1611 _] -> w1594
                    frame No Error {
                      n645 = call "ReadHeadFast.vi"("new file path"=w1609) -> ("refnum out"=w1610:refnum<file>, "Header In"=w1611:T59)  [unwired: 7 in, 2 out]
                      n646 = Close File(refnum=w1610) -> ()  [unwired: 1 in, 2 out]
                    }
                    frame Error {
                    }
                  }
                  n647 = case shown="True" w1600 {
                    tunnel: [w1612 w1616] -> w1589
                    tunnel: [w1613 w1632] -> w1588
                    tunnel: [w1613 w1628] -> w1587
                    tunnel: w1597 -> [_ w1626]
                    tunnel: [w1612 w1622] -> w1586
                    tunnel: w1594 -> [_ w1615]
                    frame False {
                      w1613 = 1
                      w1612 = 0
                    }
                    frame True {
                      n648 = Unbundle By Name(w1615) -> ("A/D info.sample rate MHz"=w1619:u16, "A/D info.# lines per scan"=w1620:u16)
                      n649 = Unbundle By Name(w1615) -> ("Scan Info.delay"=w1616:sgl, "Misc Info.c speed"=w1614:i16)
                      n650 = Unbundle By Name(w1615) -> ("Scan Settings.Distance between\nscan lines (um)"=w1621:u16)
                      n651 = To Double Precision Float(number=w1614) -> (double precision float=w1618:dbl)
                      n652 = Greater Or Equal?(x=w1626, y=3) -> (x >= y?=w1630:bool)
                      n653 = Divide(x=w1620, y=-2) -> (x/y=w1623:dbl)
                      n654 = Multiply(x=0.001, y=w1621) -> (x*y=w1624:dbl)
                      n655 = expression code="x/2000"(w1618) -> (w1617:dbl)
                      n656 = Reciprocal(x=w1619) -> (1/x=w1633:dbl)
                      n657 = Select(t=w1624, s=w1630, f=1) -> (s? t:f=w1628:dbl)
                      n658 = Multiply(x=w1624, y=w1623) -> (x*y=w1622:dbl)
                      n659 = Multiply(x=w1617, y=w1633) -> (x*y=w1632:dbl)
                    }
                  }
                  n660 = local read "Transpose"() -> (w1575:bool)
                  n661 = Build Array(w1589, w1588, w1587, w1586) -> (w1585:dbl[])
                  n662 = Index Array(array=w1585) -> (element #1=w1583:dbl, element #2=w1582:dbl, element #3=w1580:dbl, element #4=w1581:dbl)  [unwired: 4 in]
                  n663 = case shown="False" w1575 {
                    tunnel: [w1604 w1607] -> w1576
                    tunnel: w1583 -> [w1604 w1608]
                    tunnel: [w1603 w1605] -> w1577
                    tunnel: w1582 -> [w1603 w1606]
                    tunnel: [w1602 w1608] -> w1579
                    tunnel: w1581 -> [w1602 w1607]
                    tunnel: [w1601 w1606] -> w1578
                    tunnel: w1580 -> [w1601 w1605]
                    frame False {
                    }
                    frame True {
                    }
                  }
                  n664 = property on="Raw data" class="IntGraph (strict)"("X Scale.Offset and Multiplier:Offset"=w1576, "X Scale.Offset and Multiplier:Multiplier"=w1577, "Y Scale.Offset and Multiplier:Multiplier"=w1578, "Y Scale.Offset and Multiplier:Offset"=w1579) -> ()  [unwired: 2 in, 2 out]
                }
                event "Save Data": Value Change {
                  n665 = event-data() -> ()  [unwired: 2 out]
                  n666 = control-ref of="Erase data"() -> (w1636:refnum<vi>)
                  n667 = property on="Save Data" class="Bool (strict)"("Value"=FALSE ("Save Data")) -> ()  [unwired: 2 in, 2 out]
                  n668 = call "SaveDataAcqCont.vi"("Boolean in"=w1636, "Array in"=w1637, "Location"=w1635, "Type of scan"=w1634) -> ("Array out"=w1638:T55[])  [unwired: 6 in, 1 out]
                }
                event "Show Thumbs": Value Change {
                  w1650 = i16 90 ("pixels in y")
                  w1651 = i16 100 ("pixels in x")
                  # "Thumbnails are generated each time this is called. It is not at all efficient than computing as data is acquired."
                  n669 = event-data() -> ()  [unwired: 2 out]
                  n670 = call "Thumbnails.vi"("Digitizer Settings"=w1648, "pixels in y"=w1650, "pixels in x"=w1651) -> ("Thumbs out"=w1653:picture[])  [unwired: 2 in, 6 out]
                  n671 = call "ShowThumbs.vi"("pixels in y"=w1650, "pixels in x"=w1651, "columns in display"=i16 5, "Thumbnails In"=w1653) -> ()  [unwired: 3 out]
                }
                event "Erase data": Value Change {
                  w1664 = FALSE  # Data taken?
                  # "Delete local temp files"
                  # "Erase All Data"
                  n672 = event-data() -> ()  [unwired: 2 out]
                  n673 = global read "MotionGlobals.vi" "TempPath"() -> (w1657:path)
                  n674 = List Folder(path=w1657) -> (path out=w1662:path, filenames=w1661:string[], error out=w1663:errorcluster)  [unwired: 1 in, 3 out]
                  n675 = local write "Raw data"(sgl[][] [] ("Raw data")) -> ()
                  n676 = case shown="No Error" w1663 {
                    tunnel: w1662 -> [w1669 _]
                    tunnel: w1661 -> [w1668 _]
                    frame No Error {
                      n677 = for {
                        tunnel: w1669 -> [w1671]
                        tunnel: w1668 -> [w1670] mode=indexing
                        n678 = Build Path(base path=w1671, name or relative path=w1670) -> (appended path=w1672:path)
                        n679 = Delete(path (use dialog)=w1672) -> ()  [unwired: 1 in, 6 out]
                      }
                    }
                    frame Error {
                    }
                  }
                  n680 = local write "Erase data"(w1664) -> ()
                  n681 = local write "Keep?"(w1664) -> ()
                  n682 = property on="Case\nto View" class="Ring (strict)"("Strings []"=string[] [] ("Array Constant")) -> ()  [unwired: 2 in, 2 out]
                }
                event "View EYE": Value Change {
                  n683 = event-data() -> ()  [unwired: 7 out]
                  n684 = global read "MotionGlobals.vi" "SavePath"() -> (w1677:path)
                  n685 = List Folder(path=w1677, pattern="*.eye") -> (filenames=w1674:string[])  [unwired: 1 in, 4 out]
                  n686 = Index Array(array=w1674) -> (element=w1673:string)  [unwired: 1 in]
                  n687 = Build Path(base path=w1677, name or relative path=w1673) -> (appended path=w1675:path)
                  n688 = call "ViewEye.vi"("new file path"=w1675) -> ()  [unwired: 5 in]
                }
                event "prf (kHz)": Value Change {
                  # "Set up counters for one of two configurations. Select true or false manually. Will likely use external PRF version. Internal PRF uses slightly different wiring. External PRF gets set up in SetUpDigi.vi. Would be nice to use internal PRF if we get a timing board. Just need to make sure PRF ouput can be turned off so it won't interfere with a pulse train coming from the motor."
                  n689 = event-data() -> ()  [unwired: 3 out]
                  n690 = global write "PulserGlobals.vi" "prf (kHz)"("prf (kHz)") -> ()
                  n691 = Reciprocal(x="prf (kHz)") -> (1/x=w1699:dbl)
                  "Time between\n samples (ms)" <- w1699
                  n692 = case shown="False" "CTR PRF?" {
                    tunnel: w1702 -> [_ w1721]
                    tunnel: w1703 -> [_ w1720]
                    tunnel: "prf (kHz)" -> [w1707 w1719]
                    tunnel: w1684 -> [w1706 _]
                    tunnel: w1686 -> [w1705 _]
                    tunnel: w1685 -> [w1704 _]
                    frame False {
                      n693 = case shown="\"WCM Main\", Default" w1705 {
                        tunnel: w1707 -> [w1708 w1715]
                        tunnel: w1706 -> [_ w1714]
                        tunnel: w1704 -> [w1710 _]
                        frame "SERI GP" {
                          n694 = Unbundle By Name(w1710) -> ("GL Ref Out"=w1712:refnum<k7>)
                          n695 = Reciprocal(x=w1708) -> (1/x=w1709:dbl)
                          n696 = call "GL_BrkPtPRF.vi"("GL Ref Out"=w1712, "Program Name"="#PRF", "PRF (1 ms)"=w1709) -> ()  [unwired: 3 in, 2 out]
                        }
                        frame "WCM Main", Default {
                          # "These commands only valid if using a HP 33120A"
                          n697 = global read "MotionGlobals.vi" "No GPIB?"() -> (w1713:bool)
                          n698 = case shown="False" w1713 {
                            tunnel: w1715 -> [w1717 _]
                            tunnel: w1714 -> [w1716 _]
                            frame False {
                              n699 = call "33120PRF.vi"("VISA session in"=w1716, "Prf (kHz)"=w1717) -> ()  [unwired: 1 in, 6 out]
                            }
                            frame True {
                            }
                          }
                        }
                      }
                    }
                    frame True {
                      n700 = case shown="True" TRUE {
                        tunnel: w1721 -> [_ w1724]
                        tunnel: w1720 -> [_ w1723]
                        tunnel: w1719 -> [_ w1722]
                        frame False {
                        }
                        frame True {
                          # "Original method of generating PRF. Source 0 is prf and source 1 is divide down. This is left in just in case there is a need to revert to it."
                          n701 = case shown="True" w1724 {
                            tunnel: w1723 -> [w1727 _]
                            tunnel: w1722 -> [w1725 w1728]
                            frame False {
                              # "set up counters for B scan prf derives from\nencoder pulses"
                              # "Set up to count DC motor pulses"
                              n702 = call "IntPRFCount.vi"("prf (kHz)"=w1725, "prf (f)/motor (t)"=TRUE ("prf (t)/count (f)"), "therapy divide by (T)"=w1727) -> ()  [unwired: 1 in, 12 out]
                            }
                            frame True {
                              w1733 = 10123 items=["Finite Samples"=10178, "Continuous Samples"=10123, "Hardware Timed Single Point"=12522] ("sample mode")
                              # "Change freq for prf originating from counters."
                              n703 = expression code="x*1000"(w1728) -> (w1734:dbl)
                              n704 = call-poly <vilib>:"DAQmx Create Virtual Channel.vi"("frequency"=w1734, "duty cycle"=0.2, "counter"=tag "Dev1/ctr1") -> ("task out"=w1731:refnum<k21>, "error out"=w1732:errorcluster)  [unwired: 6 in, 5 out]
                              n705 = call-poly <vilib>:"DAQmx Timing.vi"("task/channels in"=w1731, "sample mode"=w1733, "error in"=w1732) -> ("task out"=w1729:refnum<k21>)  [unwired: 11 in, 1 out]
                              n706 = global write "MotionGlobals.vi" "DAQmx Task 1"(w1729) -> ()
                            }
                          }
                        }
                      }
                    }
                  }
                  n707 = Unbundle By Name(w1685) -> ("scan pair"=w1698:T12)
                  n708 = call "GetScanAxis.vi"("scan pair"=w1698) -> ("Axis 1"=w1691:i32)  [unwired: 1 in, 2 out]
                  n709 = Unbundle By Name(w1685) -> ("Motor Parameters.velocity ct/s"=w1693:dbl[])
                  n710 = Index Array(array=w1693, index=w1691) -> (element=w1692:dbl)
                  n711 = call "Find_Count_Step_Interval.vi"("Motion Settings In"=w1685, "Axis"=w1691) -> ("Steps per mm"=w1689:i32)  [unwired: 8 in, 1 out]
                  n712 = Multiply(x=w1692, y=w1699) -> (x*y=w1690:dbl)
                  n713 = Divide(x=w1690, y=w1689) -> (x/y=→"Estimated Line spacing":dbl)
                }
                event "Transducer": Value Change {
                  n714 = event-data() -> ("OldVal"=w1737:u32, "NewVal"=w1739:u32)  [unwired: 1 out]
                  n715 = Not Equal?(x=w1737, y=w1739) -> (x != y?=w1743:bool)
                  n716 = case shown="\"NI Switch\"" w1741 {
                    tunnel: w1739 -> [w1752 w1755 w1759 _ w1776]
                    tunnel: w1747 -> [w1750 w1753 w1757 w1771 w1790]
                    tunnel: w1746 -> [w1751 w1754 w1758 w1772 w1789]
                    tunnel: [w1751 w1754 w1758 w1772 w1783] -> w1745
                    tunnel: [w1750 w1753 w1757 w1771 w1788] -> w1744
                    tunnel: w1743 -> [_ _ _ _ w1785]
                    tunnel: w1742 -> [_ _ _ _ w1774]
                    tunnel: w1736 -> [_ _ _ _ w1773]
                    frame "Cytex" {
                      n717 = call "Cytex.vi"("Xmit Ring"=w1752) -> ()  [unwired: 2 in, 3 out]
                    }
                    frame "Pickering" {
                      n718 = disable-structure shown="Disabled" {
                        disable-tunnel: w1755 -> [w1756 _]
                        frame Disabled {
                          n719 = call "PickeringBlank.vi"("Xmit Ring"=w1756) -> ()  [unwired: 5 out]
                        }
                        frame Enabled {
                        }
                      }
                    }
                    frame "NI Switch" {
                      n720 = disable-structure shown="Disabled" {
                        disable-tunnel: w1759 -> [w1760 _]
                        frame Disabled {
                          n721 = Decrement(x=w1760) -> (x-1=w1770:u32)
                          n722 = Number To Decimal String(number=w1770) -> (decimal integer string=w1769:string)  [unwired: 1 in]
                          n723 = global read "MotionGlobals.vi" "NI Switch"() -> (w1763:refnum<k15>)
                          n724 = Concatenate Strings("ch", w1769) -> (w1761:string)
                          n725 = call <instrlib>:"niSwitch Disconnect All Channels.vi"("instrument handle"=w1763) -> ("error out"=w1765:errorcluster, "instrument handle out"=w1764:refnum<k15>)  [unwired: 9 in]
                          n726 = call-poly <instrlib>:"niSwitch Connect Channels.vi"("error in (no error)"=w1765, "channel 2"="com0", "channel 1"=w1761, "instrument handle"=w1764) -> ("error out"=w1766:errorcluster, "instrument handle out"=w1767:refnum<k15>)  [unwired: 6 in]
                          n727 = call <instrlib>:"niSwitch Wait For Debounce.vi"("error in (no error)"=w1766, "instrument handle"=w1767) -> ()  [unwired: 8 in, 2 out]
                        }
                        frame Enabled {
                        }
                      }
                    }
                    frame "No Switch", Default {
                    }
                    frame "Riverside USB" {
                      n728 = Equal?(x=u32 1, y=w1776) -> (x = y?=w1780:bool)
                      n729 = Equal?(x=u32 2, y=w1776) -> (x = y?=w1779:bool)
                      n730 = Or(x=w1779, y=w1780) -> (x .or. y?=w1775:bool)
                      n731 = Compound Arithmetic op=AND(w1785, w1775) -> (w1781:bool)
                      n732 = case shown="True" w1781 {
                        tunnel: w1790 -> [w1792 w1805]
                        tunnel: w1776 -> [_ w1808]
                        tunnel: w1789 -> [w1791 w1807]
                        tunnel: [w1791 w1806] -> w1783
                        tunnel: [w1792 w1802] -> w1788
                        tunnel: w1774 -> [_ w1801]
                        tunnel: w1773 -> [_ w1793]
                        frame False {
                        }
                        frame True {
                          n733 = Unbundle By Name(w1801) -> ("XDCR Offset"=w1795:dbl[])
                          n734 = control-ref of="Filter Prams"() -> (w1797:refnum<vi>)
                          n735 = call "ChooseDualXDCRSettings.vi"("Digitizer Settings in"=w1807, "Switch T/R"=w1808, "Pulser"=w1793, "Motion Settings in"=w1805, "Dual XDCR Settings"=w1801, "Setup Time\nParameters (F)"=FALSE ("Setup Time\nParameters (F)"), "Filter Parameters Ref"=w1797) -> ("Digitizer Settings"=w1806:T13, "Change Polarity"=w1803:i32, "Motion Settings"=w1804:T10)  [unwired: 18 in]
                          n736 = Array Size(array=w1795) -> (size(s)=w1796:i32)
                          n737 = Not Equal To 0?(x=w1796) -> (x != 0?=w1794:bool)
                          n738 = case shown="True" w1794 {
                            tunnel: w1804 -> [w1809 w1815]
                            tunnel: w1803 -> [_ w1814]
                            tunnel: [w1809 w1813] -> w1802
                            tunnel: T49."Relative Position" ("Position Mode (Absolute)") -> [_ w1812]
                            tunnel: TRUE ("Find Location") -> [_ w1811]
                            tunnel: w1795 -> [_ w1810]
                            frame False {
                            }
                            frame True {
                              n739 = call "MultiAxisMove.vi"("Find Location"=w1811, "Position Mode (Rel)"=w1812, "Distance to move (mm)"=w1810, "Move Polarity"=w1814, "Motion Settings"=w1815) -> ("Motion Settings Out"=w1813:T10)  [unwired: 4 in, 2 out]
                            }
                          }
                        }
                      }
                      n740 = Unbundle By Name(w1788) -> ("number of scan planes"=w1784:i32, "Distance between\nscan lines (um)"=w1787:sgl, "Distance between\nscan planes (um)"=w1786:sgl)
                      n741 = Unbundle By Name(w1783) -> ("lines per plane"=w1782:i32)
                      n742 = property on="number of planes" class="DigNum (strict)"("Value"=w1784) -> ()  [unwired: 2 in, 2 out]
                      n743 = property on="Distance between\nscan lines (um)" class="DigNum (strict)"("Val(Sgnl)"=w1787) -> ()  [unwired: 2 in, 2 out]
                      n744 = property on="Distance between\nplanes (um)" class="DigNum (strict)"("Val(Sgnl)"=w1786) -> ()  [unwired: 2 in, 2 out]
                      n745 = property on="lines per plane" class="DigNum (strict)"("Value"=w1782) -> ()  [unwired: 2 in, 2 out]
                    }
                  }
                  n746 = Bundle By Name(cluster=w1740, "Switch T/R"=w1739) -> (w1738:T50)
                }
                event "Man Cont": Value Change {
                  n747 = event-data() -> ()  [unwired: 2 out]
                  n748 = call "MotionProfileChange.vi"("Motion Mode"=enum16{"Move Mode", "Scan Mode"}."Move Mode", "Location"=w1818, "Motion Settings In in"=w1820) -> ("Motion Settings In out"=w1819:T10)  [unwired: 8 in]
                  n749 = Unbundle By Name(w1819) -> ("Motion System"=w1823:T11)
                  n750 = case shown="\"NI 735x\", Default" w1823 {
                    tunnel: w1819 -> [w1828 w1834 w1837 w1838]
                    tunnel: [w1827 w1833 w1836 w1838] -> w1822
                    frame "NI 735x", Default {
                      n751 = disable-structure shown="Enabled" {
                        disable-tunnel: w1828 -> [w1830 w1832]
                        disable-tunnel: [w1829 w1832] -> w1827
                        frame Disabled {
                          n752 = call "NI_controller.VI"("Motion Settings"=w1830, "Initialize"=FALSE) -> ("Motion Settings Out"=w1829:T10)  [unwired: 3 in, 1 out]
                        }
                        frame Enabled {
                        }
                      }
                    }
                    frame "Galil" {
                      n753 = call "GL_controller.VI"("Motion Settings"=w1834, "Initialize"=FALSE) -> ("Motion Settings Out"=w1833:T10)  [unwired: 3 in, 1 out]
                    }
                    frame "Newport ESP" {
                      n754 = call "ESPControl.vi"("Motion Settings"=w1837) -> ("Motion Settings Out"=w1836:T10)  [unwired: 4 in, 1 out]
                    }
                    frame "MM3000", "No Motion Card" {
                    }
                  }
                }
                event "Set Pulser": Value Change {
                  n755 = event-data() -> ()  [unwired: 2 out]
                  n756 = Unbundle By Name(w1840) -> ("Switch T/R"=w1839:i16)
                  n757 = flat-sequence {
                    tunnel: w1841 -> [w1849]
                    tunnel: w1846 -> [w1855]
                    tunnel: w1845 -> [w1854]
                    tunnel: w1844 -> [w1853]
                    tunnel: w1843 -> [w1852]
                    tunnel: [w1851] -> w1842
                    tunnel: w1839 -> [w1850]
                    frame #0 {
                      n758 = call "SetAllPulsersGUI.vi"("Pulser"=w1849) -> ()  [unwired: 11 in]
                    }
                    frame #1 {
                      n759 = call "UpdateDualXDCRSettings.vi"("Digitizer Settings in"=w1855, "Motion Settings in"=w1854, "Switch T/R"=w1850, "Dual XDCR Settings In"=w1852, "Switch Unit"=w1853) -> ("Dual XDCR Settings"=w1851:T24)  [unwired: 3 in]
                    }
                  }
                }
                event "Focal Zones", "Xmt/Rcv": Value Change {
                  n760 = event-data() -> ()  [unwired: 7 out]
                  n761 = call "F-Zones.vi"("Trans Geometry (mm)"="Trans Geometry (mm)") -> ("Trans Geometry (mm) out"=w1859:T8)  [unwired: 7 in, 3 out]
                  n762 = Bundle By Name(cluster=w1858, "Focal Zones"="Focal Zones", "Trans Geometry (mm)"=w1859, "Xmt/Rcv"="Xmt/Rcv") -> (w1856:T50)
                  n763 = local write "Trans Geometry (mm)"(w1859) -> ()
                }
                event "Keep?": Value Change {
                  # "Update whether to save file"
                  n764 = event-data() -> ("NewVal"=w1872:bool)  [unwired: 1 out]
                  n765 = in-place {
                    in-place-border: w1872 -> [w1877]
                    n766 = in-place-array #1(w1874, w1873) -> (w1878:T55)
                    n767 = in-place {
                      in-place-border: w1877 -> [w1879]
                      n768 = in-place-cluster #2(w1878) -> ()  [unwired: 1 out]
                      n769 = in-place-cluster #2("Keep?"=w1879) -> (w1876:T55)
                    }
                    n770 = in-place-array #1(w1876) -> (w1871:T55[])  [unwired: 1 out]
                  }
                }
                event "RT fps": Value Change {
                  n771 = event-data() -> ("NewVal"=w1885:sgl)  [unwired: 1 out]
                  n772 = Bundle By Name(cluster=w1886, "RT fps"=w1885) -> (w1884:T10)
                  n773 = Unbundle By Name(w1884) -> ("overshoot cts"=w1887:i32, "Total steps in line"=w1883:i32, "Distance between\nscan lines (um)"=w1882:sgl)
                  n774 = expression code="x*2"(w1887) -> (w1892:i32)
                  n775 = Add(x=w1892, y=w1883) -> (x+y=w1891:i32)
                  n776 = call "CalcVandA.vi"("distance"=w1891, "fps"=w1885) -> ("Velocity"=w1890:dbl)  [unwired: 2 out]
                  "RT V" <- w1890
                  n777 = Divide(x=w1890, y=w1882) -> (x/y=→"Trig (Hz)":dbl)
                }
                event "TimeOut (s)": Value Change {
                  n778 = event-data() -> ("NewVal"=w1898:sgl)  [unwired: 1 out]
                  n779 = Bundle By Name(cluster=w1900, "DigTimeOut"=w1898) -> (w1899:T13)
                }
                event "Case Name": Value Change {
                  (unwired) "*"
                  # "Pull all named files"
                  n780 = event-data() -> ("NewVal"=w1917:string)  [unwired: 1 out]
                  n781 = global read "MotionGlobals.vi" "SavePath"() -> (w1905:path)
                  n782 = Concatenate Strings(w1917, "00*") -> (w1916:string)
                  n783 = List Folder(path=w1904, pattern=w1916) -> (filenames=w1914:string[])  [unwired: 1 in, 4 out]
                  n784 = List Folder(path=w1905, pattern=w1916) -> (filenames=w1915:string[])  [unwired: 1 in, 4 out]
                  n785 = Array Size(array=w1914) -> (size(s)=w1912:i32)
                  n786 = Array Size(array=w1915) -> (size(s)=w1913:i32)
                  n787 = Add(x=w1913, y=w1912) -> (x+y=w1911:i32)
                  n788 = case shown="1, Default" w1911 {
                    frame 0 {
                    }
                    frame 1, Default {
                      n789 = One Button Dialog(message="File has been used already. Select a new file name.") -> ()  [unwired: 1 in, 1 out]
                    }
                  }
                }
                event "Overshoot", "BKPT Shift": Value Change {
                  n790 = event-data() -> ()  [unwired: 2 out]
                  n791 = Bundle By Name(cluster=w1925, "overshoot cts"="Overshoot", "BKPT Shift"="BKPT Shift") -> (w1924:T10)
                }
                event "Bulk Acq", "Full Array Scan?", "Synth Foc?", "GPU?", "Save TIFF?", "DownFactor", "RCV 1CH": Value Change {
                  # "Turn off Bulk acq if any of the listed conditions are False"
                  n792 = event-data() -> ()  [unwired: 7 out]
                  n793 = Unbundle By Name(w1945) -> ("Avg Num"=w1948:i32, "Dig Config"=w1947:T15)
                  n794 = Equal?(x=w1947, y=4) -> (x = y?=w1950:bool)
                  n795 = Equal?(x=w1947, y=5) -> (x = y?=w1955:bool)
                  n796 = Equal To 0?(x=w1939) -> (x = 0?=w1952:bool)
                  n797 = Equal?(x=1, y=w1948) -> (x = y?=w1954:bool)
                  n798 = Compound Arithmetic op=AND("Full Array Scan?", w1954, w1955, w1952) -> (w1943:bool)
                  n799 = Compound Arithmetic op=AND("Full Array Scan?", w1950) -> (w1949:bool)
                  n800 = case shown="True" w1949 {
                    tunnel: [w1959 w1960] -> w1933
                    tunnel: "Full Array Scan?" -> [w1959 _]
                    frame False {
                    }
                    frame True {
                      w1960 = FALSE ("Full Array Scan?")
                      n801 = local write "Full Array Scan?"(w1960) -> ()
                    }
                  }
                  n802 = Select(t="Bulk Acq", s=w1943, f=FALSE) -> (s? t:f=w1940:bool)
                  n803 = Bundle By Name(cluster=w1937, "Synth Foc?"="Synth Foc?", "Full Array Scan?"=w1933, "GPU?"="GPU?", "Save TIFF?"="Save TIFF?", "downfactor"="DownFactor", "RCV 1CH"="RCV 1CH") -> (w1936:T50)
                  n804 = Bundle By Name(cluster=w1945, "Bulk Acq"=w1940) -> (w1944:T13)
                }
                event "Avg Num": Value Change {
                  n805 = event-data() -> ("NewVal"=w1966:i32, "OldVal"=w1972:i32)  [unwired: 1 out]
                  n806 = Unbundle By Name(w1968) -> ("lines per plane"=w1967:i32)
                  n807 = case shown="-1..1" w1966 {
                    tunnel: [0 ("Overshoot") w1975] -> w1963
                    frame 2, Default {
                    }
                    frame -1..1 {
                      n808 = local read "Overshoot"() -> (w1975:i32)
                    }
                  }
                  n809 = case shown="0" w1966 {
                    selector: w1966 -> [_ w1981]
                    tunnel: [w1976 w1981] -> w1970
                    tunnel: w1972 -> [w1980 _]
                    frame 0 {
                      w1977 = -1
                      n810 = Equal?(x=w1980, y=w1977) -> (x = y?=w1979:bool)
                      n811 = Select(t=1, s=w1979, f=w1977) -> (s? t:f=w1976:i32)
                      n812 = local write "Avg Num"(w1976) -> ()
                    }
                    frame 1, Default {
                    }
                  }
                  n813 = property on="lines per plane" class="DigNum (strict)"("Val(Sgnl)"=w1967) -> ()  [unwired: 2 in, 2 out]
                  n814 = Bundle By Name(cluster=w1965, "overshoot cts"=w1963) -> (w1964:T10)
                  n815 = Bundle By Name(cluster=w1968, "Avg Num"=w1970) -> (w1969:T13)
                }
                event "c mm/mics": Value Change {
                  n816 = event-data() -> ()  [unwired: 2 out]
                  n817 = global write "MotionGlobals.vi" "c mm/mics"("c mm/mics") -> ()
                }
                event "One Way Scan": Value Change {
                  n818 = event-data() -> ()  [unwired: 2 out]
                  n819 = property on="One Way Scan" class="Bool (strict)"() -> ("Visible"=w1990:bool)  [unwired: 2 in, 2 out]
                  n820 = And(x="One Way Scan", y=w1990) -> (x .and. y?=w1991:bool)
                  n821 = Bundle By Name(cluster=w1995, "One Way Scan"="One Way Scan") -> (w1994:T10)
                  n822 = property on="Reverse One \nWay Scan" class="Bool (strict)"("Visible"=w1991) -> ()  [unwired: 2 in, 2 out]
                }
                event "Reverse One \nWay Scan": Value Change {
                  n823 = event-data() -> ()  [unwired: 3 out]
                  n824 = Bundle By Name(cluster=w2003, "Reverse One Way Scan"="Reverse One \nWay Scan") -> (w2001:T10)
                }
                event "Multi Trig", "Multi Trig#", "Multi Time (us)", "USB Gate\nPer Sample": Value Change {
                  n825 = event-data() -> ()  [unwired: 2 out]
                  n826 = Unbundle By Name(w2013) -> ("lines per plane"=w2012:i32)
                  n827 = local read "USB Gate\nPer Sample"() -> (w2008:bool)
                  n828 = local read "Multi Trig"() -> (w2014:bool)
                  n829 = local read "Multi Trig#"() -> (w2015:i32)
                  n830 = global write "MotionGlobals.vi" "Multi Trig?"(w2014) -> ()
                  n831 = global write "SwitchGlobals.vi" "PulseSpacing (us)"("Multi Time (us)") -> ()
                  n832 = global write "MotionGlobals.vi" "Multi Trig#"(w2015) -> ()
                  n833 = global write "MotionGlobals.vi" "USB Gate Per Sample"(w2008) -> ()
                  n834 = property on="lines per plane" class="DigNum (strict)"("Val(Sgnl)"=w2012) -> ()  [unwired: 2 in, 2 out]
                }
                event "DAQ Range": Value Change {
                  n835 = event-data() -> ("NewVal"=w2023:cluster{"Max V":dbl, "Min V":dbl})  [unwired: 1 out]
                  n836 = global write "MotionGlobals.vi" "DAQ Range"(w2023) -> ()
                }
                event Value Change {
                  # "Erase data if using a new scan mode. Need to fix."
                  n837 = event-data() -> ("NewVal"=w2030:T21, "OldVal"=w2029:T21)  [unwired: 1 out]
                  n838 = Not Equal?(x=w2030, y=w2029) -> ()  [unwired: 1 out]
                  n839 = case shown="False" FALSE {
                    frame False {
                    }
                    frame True {
                      n840 = property on="Erase data" class="Bool (strict)"("Value (Signaling)"=FALSE) -> ()  [unwired: 2 in, 2 out]
                    }
                  }
                }
                event "Debug Mode?": Value Change {
                  n841 = event-data() -> ()  [unwired: 3 out]
                }
                event "Resp Divide": Value Change {
                  n842 = event-data() -> ("NewVal"=w2048:i32)  [unwired: 1 out]
                  n843 = global write "MotionGlobals.vi" "Breath Divide"(w2048) -> ()
                }
                event "LeCroy Channels": Value Change {
                  n844 = event-data() -> ("NewVal"=w2053:bool[])  [unwired: 1 out]
                  n845 = Bundle By Name(cluster=w2055, "LeCroyCluster.LeCroy Channels"=w2053) -> (w2054:T13)
                }
                event "Sweep\nAvg": Value Change {
                  n846 = event-data() -> ("NewVal"=w2061:bool)  [unwired: 1 out]
                  n847 = Bundle By Name(cluster=w2063, "LeCroyCluster.Sweep Avg"=w2061) -> (w2062:T13)
                }
                event "CTR PRF?": Value Change {
                  # "Select Internal CTR on Dev1 for PRF if Dev1."
                  n848 = event-data() -> ("NewVal"=w2071:bool)  [unwired: 1 out]
                  n849 = global write "MotionGlobals.vi" "CTR PRF?"(w2071) -> ()
                }
                event "Xtra delay (us)": Value Change {
                  n850 = event-data() -> ("NewVal"=w2073:dbl)  [unwired: 1 out]
                  n851 = Bundle By Name(cluster=w2075, "Xtra Ann Trig delay (us)"=w2073) -> (w2074:T13)
                }
                event "Save Temp": Value Change {
                  n852 = event-data() -> ()  [unwired: 2 out]
                  n853 = global write "MotionGlobals.vi" "Save Temp"("Save Temp") -> ()
                }
                event "Resp Wait (ms)": Value Change {
                  n854 = event-data() -> ("NewVal"=w2093:u32)  [unwired: 1 out]
                  n855 = global write "MotionGlobals.vi" "Resp Wait (ms)"(w2093) -> ()
                }
                event "Dopp\nGate?": Value Change {
                  n856 = event-data() -> ()  [unwired: 2 out]
                  n857 = global write "MotionGlobals.vi" "Dopp Gate?"("Dopp\nGate?") -> ()
                }
                event "Add Axis": Value Change {
                  n858 = event-data() -> ("NewVal"=w2102:bool)  [unwired: 1 out]
                  n859 = Bundle By Name(cluster=w2106, "Add Axis"=w2102) -> (w2105:T10)
                  n860 = property on="Xtra plane\ndistance  (um)" class="DigNum (strict)"("Visible"=w2102) -> ()  [unwired: 2 in, 2 out]
                  n861 = property on="Xtra planes" class="DigNum (strict)"("Visible"=w2102) -> ()  [unwired: 2 in, 2 out]
                  n862 = property on="3rd Axis" class="Ring (strict)"("Visible"=w2102) -> ()  [unwired: 2 in, 2 out]
                  n863 = property on="Cross plane\nlength (mm)" class="DigNum (strict)"("Visible"=w2102) -> ()  [unwired: 2 in, 2 out]
                  n864 = case shown="True" w2102 {
                    frame False {
                    }
                    frame True {
                      n865 = property on="scan pair" class="Enum (strict)"() -> ("Value"=w2116:T12)  [unwired: 2 in, 2 out]
                      n866 = call "GetScanAxis.vi"("scan pair"=w2116) -> ("Axis 1"=w2115:i32, "Axis 2"=w2114:i32, "Axis 3"=w2111:i32)  [unwired: 1 in]
                      n867 = Build Array(w2115, w2114) -> (w2113:i32[])
                      n868 = Decrement(x=w2111) -> (x-1=w2110:i32)
                      n869 = Decrement(x=w2113) -> (x-1=w2112:i32[])
                      n870 = property on="3rd Axis" class="Ring (strict)"("Value"=w2110) -> ()  [unwired: 2 in, 2 out]
                      n871 = property on="3rd Axis" class="Ring (strict)"("Disabled Items []"=w2112) -> ()  [unwired: 2 in, 2 out]
                    }
                  }
                }
                event Value Change {
                  n872 = event-data() -> ()  [unwired: 2 out]
                  n873 = Bundle By Name(cluster=w2118, "3rd Axis"="3rd Axis") -> (w2117:T10)
                }
                event "Microscopy Scan Mode": Value Change {
                  n874 = event-data() -> ()  [unwired: 2 out]
                  n875 = global read "MotionGlobals.vi" "Vz Counter"() -> (w2141:i16)
                  n876 = property on="Auto Vz?" class="Bool (strict)"() -> ("Value"=w2126:bool)  [unwired: 2 in, 2 out]
                  n877 = case shown="\"Acoustic Microscopy\", Default" w2129 {
                    tunnel: "HF XDCR" -> [w2161]
                    tunnel: "Microscopy Scan Mode" -> [w2160]
                    tunnel: w2143 -> [w2159]
                    tunnel: [w2158] -> w2142
                    tunnel: w2141 -> [w2157]
                    tunnel: [w2156] -> w2139
                    tunnel: [w2155] -> w2136
                    tunnel: [w2154] -> w2135
                    tunnel: [w2153] -> w2134
                    tunnel: [w2152] -> w2131
                    tunnel: w2128 -> [w2151]
                    tunnel: [w2151] -> w2127
                    tunnel: w2126 -> [w2150]
                    tunnel: w2125 -> [w2149]
                    frame "Acoustic Microscopy", Default {
                      n878 = case shown="\"V-Z Scan\"" w2160 {
                        tunnel: w2161 -> [w2168 w2189 w2216 w2250 w2308]
                        tunnel: [w2167 w2188 w2215 w2249 w2307] -> w2155
                        tunnel: [w2166 w2187 w2214 w2248 w2306] -> w2152
                        tunnel: [w2165 w2186 w2213 w2247 w2305] -> w2154
                        tunnel: [w2164 w2185 w2212 w2246 w2304] -> w2156
                        tunnel: [w2163 w2184 w2211 w2245 w2303] -> w2153
                        tunnel: w2159 -> [w2162 w2183 w2210 w2243 w2301]
                        tunnel: w2157 -> [_ _ w2209 w2244 w2302]
                        tunnel: [w2162 w2183 w2207 w2241 w2298] -> w2158
                        tunnel: w2150 -> [_ _ _ _ w2299]
                        tunnel: w2149 -> [_ _ w2205 _ _]
                        frame "Level X" {
                          n879 = case shown="\"500 MHz\"" w2168 {
                            tunnel: [ScanAxis."x-(y) scan" ("scan pair") ScanAxis."x-(y) scan" ("scan pair")] -> w2167
                            tunnel: [4001 8001] -> w2166
                            tunnel: [2.0 ("Length of\none plane (mm)") 1.0 ("Length of\none plane (mm)")] -> w2165
                            tunnel: [1 1] -> w2164
                            tunnel: [sgl 40.0 20] -> w2163
                            frame "250 MHz", Default {
                              n880 = property on="Length of\nall planes (mm)" class="DigNum (strict)"("Value"=0.0 ("Length of\nall planes (mm)")) -> ()  [unwired: 2 in, 2 out]
                              n881 = property on="Length of\none plane (mm)" class="DigNum (strict)"("Value"=8.0 ("Length of\none plane (mm)")) -> ()  [unwired: 2 in, 2 out]
                            }
                            frame "500 MHz" {
                              n882 = property on="Length of\nall planes (mm)" class="DigNum (strict)"("Value"=0.0 ("Length of\nall planes (mm)")) -> ()  [unwired: 2 in, 2 out]
                              n883 = property on="Length of\none plane (mm)" class="DigNum (strict)"("Value"=8.0 ("Length of\none plane (mm)")) -> ()  [unwired: 2 in, 2 out]
                            }
                          }
                        }
                        frame "Level Y" {
                          n884 = case shown="\"500 MHz\"" w2189 {
                            tunnel: [ScanAxis."y-(x) scan" ("scan pair") ScanAxis."y-(x) scan" ("scan pair")] -> w2188
                            tunnel: [4001 8001] -> w2187
                            tunnel: [2.0 ("Length of\none plane (mm)") 1.0 ("Length of\none plane (mm)")] -> w2186
                            tunnel: [1 1] -> w2185
                            tunnel: [sgl 40.0 sgl 20.0] -> w2184
                            frame "250 MHz", Default {
                              n885 = property on="Length of\nall planes (mm)" class="DigNum (strict)"("Value"=0.0 ("Length of\nall planes (mm)")) -> ()  [unwired: 2 in, 2 out]
                              n886 = property on="Length of\none plane (mm)" class="DigNum (strict)"("Value"=8.0 ("Length of\none plane (mm)")) -> ()  [unwired: 2 in, 2 out]
                            }
                            frame "500 MHz" {
                              n887 = property on="Length of\nall planes (mm)" class="DigNum (strict)"("Value"=0.0 ("Length of\nall planes (mm)")) -> ()  [unwired: 2 in, 2 out]
                              n888 = property on="Length of\none plane (mm)" class="DigNum (strict)"("Value"=8.0 ("Length of\none plane (mm)")) -> ()  [unwired: 2 in, 2 out]
                            }
                          }
                        }
                        frame "Overview Scan", Default {
                          n889 = Greater Or Equal To 0?(x=w2209) -> (x >= 0?=w2208:bool)
                          n890 = call "EraseLevelingScans.vi"("Array in"=w2205) -> ("All Leveling Scans?"=w2204:bool)  [unwired: 10 in]
                          n891 = case shown="False" w2208 {
                            tunnel: w2210 -> [w2217 w2223]
                            tunnel: [w2217 w2222] -> w2206
                            frame False {
                            }
                            frame True {
                              n892 = property on="Digitizer delay (us) (Temp)" class="DigNum (strict)"() -> ("Value"=w2219:dbl)  [unwired: 2 in, 2 out]
                              n893 = property on="Additional dig delay (us) Temp" class="DigNum (strict)"() -> ("Value"=w2220:dbl)  [unwired: 2 in, 2 out]
                              n894 = property on="rf points per line Temp" class="DigNum (strict)"() -> ("Value"=w2221:i32)  [unwired: 2 in, 2 out]
                              n895 = property on="LC read pt offset temp" class="DigNum (strict)"() -> ("Value"=w2218:dbl)  [unwired: 2 in, 2 out]
                              n896 = Bundle By Name(cluster=w2223, "Digitizer delay (us)"=w2219, "rf points per line"=w2221, "Additional dig delay (us)"=w2220, "LeCroyCluster.LC read pt offset"=w2218) -> (w2222:T13)
                            }
                          }
                          n897 = case shown="\"250 MHz\", Default" w2216 {
                            tunnel: [ScanAxis."x-(y) scan" ("scan pair") ScanAxis."x-(y) scan" ("scan pair")] -> w2215
                            tunnel: [1001 1001] -> w2214
                            tunnel: [2.0 ("Length of\none plane (mm)") 1.0 ("Length of\none plane (mm)")] -> w2213
                            tunnel: [51 51] -> w2212
                            tunnel: [sgl 40.0 sgl 20.0] -> w2211
                            tunnel: [w2224 w2232] -> w2207
                            tunnel: w2206 -> [w2224 w2232]
                            frame "250 MHz", Default {
                              n898 = property on="Length of\nall planes (mm)" class="DigNum (strict)"("Value"=2.0 ("Length of\nall planes (mm)")) -> ()  [unwired: 2 in, 2 out]
                              n899 = property on="Length of\none plane (mm)" class="DigNum (strict)"("Value"=2.0 ("Length of\none plane (mm)")) -> ()  [unwired: 2 in, 2 out]
                            }
                            frame "500 MHz" {
                              n900 = property on="Length of\nall planes (mm)" class="DigNum (strict)"("Value"=1.0 ("Length of\nall planes (mm)")) -> ()  [unwired: 2 in, 2 out]
                              n901 = property on="Length of\none plane (mm)" class="DigNum (strict)"("Value"=1.0 ("Length of\none plane (mm)")) -> ()  [unwired: 2 in, 2 out]
                            }
                          }
                          n902 = property on="Erase data" class="Bool (strict)"("Val(Sgnl)"=w2204) -> ()  [unwired: 2 in, 2 out]
                        }
                        frame "Detailed Scan" {
                          n903 = Greater Or Equal To 0?(x=w2244) -> (x >= 0?=w2242:bool)
                          n904 = case shown="True" w2242 {
                            tunnel: [w2251 w2258] -> w2240
                            tunnel: w2243 -> [w2251 w2257]
                            frame False {
                            }
                            frame True {
                              n905 = property on="Digitizer delay (us) (Temp)" class="DigNum (strict)"() -> ("Value"=w2253:dbl)  [unwired: 2 in, 2 out]
                              n906 = property on="rf points per line Temp" class="DigNum (strict)"() -> ("Value"=w2256:i32)  [unwired: 2 in, 2 out]
                              n907 = property on="Additional dig delay (us) Temp" class="DigNum (strict)"() -> ("Value"=w2255:dbl)  [unwired: 2 in, 2 out]
                              n908 = property on="LC read pt offset temp" class="DigNum (strict)"() -> ("Value"=w2254:dbl)  [unwired: 2 in, 2 out]
                              n909 = Bundle By Name(cluster=w2257, "Digitizer delay (us)"=w2253, "rf points per line"=w2256, "Additional dig delay (us)"=w2255, "LeCroyCluster.LC read pt offset"=w2254) -> (w2258:T13)
                              n910 = property on="Length of\nall planes (mm) Temp" class="DigNum (strict)"() -> ("Value"=w2252:dbl)  [unwired: 2 in, 2 out]
                              n911 = property on="Length of\nall planes (mm)" class="DigNum (strict)"("Value"=w2252) -> ()  [unwired: 2 in, 2 out]
                            }
                          }
                          n912 = case shown="\"250 MHz\"" w2250 {
                            tunnel: [ScanAxis."x-(y) scan" ("scan pair") ScanAxis."x-(y) scan" ("scan pair")] -> w2249
                            tunnel: [w2267 w2283] -> w2248
                            tunnel: [w2269 w2285] -> w2247
                            tunnel: [w2262 w2278] -> w2246
                            tunnel: [w2260 w2276] -> w2245
                            tunnel: [w2259 w2275] -> w2241
                            tunnel: w2240 -> [w2259 w2275]
                            frame "500 MHz" {
                              w2260 = sgl 1.0
                              w2269 = 1.0 ("Length of\none plane (mm)")
                              n913 = property on="Length of\nall planes (mm)" class="DigNum (strict)"() -> ("Value"=w2261:dbl)  [unwired: 2 in, 2 out]
                              n914 = To Double Precision Float(number=w2260) -> (double precision float=w2264:dbl)
                              n915 = property on="Length of\none plane (mm)" class="DigNum (strict)"() -> ("Value"=w2268:dbl)  [unwired: 2 in, 2 out]
                              n916 = expression code="x*1e-3"(w2264) -> (w2265:dbl)
                              n917 = To Double Precision Float(number=w2269) -> (double precision float=w2271:dbl)
                              n918 = Divide(x=w2261, y=w2265) -> (x/y=w2266:dbl)
                              n919 = expression code="x*1e-3"(w2271) -> (w2272:dbl)
                              n920 = Round To Nearest(number=w2266) -> (nearest integer value=w2263:dbl)
                              n921 = Increment(x=w2263) -> (x+1=w2262:dbl)
                              n922 = Divide(x=w2268, y=w2272) -> (x/y=w2273:dbl)
                              n923 = Round To Nearest(number=w2273) -> (nearest integer value=w2270:dbl)
                              n924 = Increment(x=w2270) -> (x+1=w2267:dbl)
                            }
                            frame "250 MHz" {
                              w2276 = sgl 2.0
                              w2285 = 2.0 ("Length of\none plane (mm)")
                              n925 = property on="Length of\nall planes (mm)" class="DigNum (strict)"() -> ("Value"=w2277:dbl)  [unwired: 2 in, 2 out]
                              n926 = To Double Precision Float(number=w2276) -> (double precision float=w2280:dbl)
                              n927 = property on="Length of\none plane (mm)" class="DigNum (strict)"() -> ("Value"=w2284:dbl)  [unwired: 2 in, 2 out]
                              n928 = expression code="x*1e-3"(w2280) -> (w2281:dbl)
                              n929 = To Double Precision Float(number=w2285) -> (double precision float=w2287:dbl)
                              n930 = Divide(x=w2277, y=w2281) -> (x/y=w2282:dbl)
                              n931 = expression code="x*1e-3"(w2287) -> (w2288:dbl)
                              n932 = Round To Nearest(number=w2282) -> (nearest integer value=w2279:dbl)
                              n933 = Increment(x=w2279) -> (x+1=w2278:dbl)
                              n934 = Divide(x=w2284, y=w2288) -> (x/y=w2289:dbl)
                              n935 = Round To Nearest(number=w2289) -> (nearest integer value=w2286:dbl)
                              n936 = Increment(x=w2286) -> (x+1=w2283:dbl)
                            }
                          }
                        }
                        frame "V-Z Scan" {
                          n937 = control-ref of="Length of\nall planes (mm)"() -> (w2296:refnum<vi>)
                          n938 = call "VzScanSettingsHandler.vi"("Vz Counter"=w2302, "Digitizer Settings in"=w2301, "Length of all Planes (mm)"=w2296) -> ("Digitizer Settings out"=w2297:T13, "rf points per line Temp"=→"rf points per line Temp":i32, "Additional dig delay (us) Temp"=→"Additional dig delay (us) Temp":dbl, "Length of\nall planes (mm) Temp"=→"Length of\nall planes (mm) Temp":dbl, "Digitizer delay (us) (Temp)"=→"Digitizer delay (us) (Temp)":dbl, "LC read pt offset temp"=→"LC read pt offset temp":dbl)  [unwired: 3 in]
                          n939 = case shown="\"500 MHz\"" w2308 {
                            tunnel: [ScanAxis."x-(z) scan" ("scan pair") ScanAxis."x-(z) scan" ("scan pair")] -> w2307
                            tunnel: [w2320 w2339] -> w2306
                            tunnel: [w2322 w2341] -> w2305
                            tunnel: [w2315 w2334] -> w2304
                            tunnel: [w2314 w2333] -> w2303
                            tunnel: w2299 -> [w2313 w2332]
                            tunnel: "Auto Vz Depth" -> [w2312 w2331]
                            tunnel: [w2309 w2328] -> w2298
                            tunnel: w2297 -> [w2309 w2328]
                            frame "500 MHz" {
                              w2314 = sgl 1.0
                              w2322 = 1.0 ("Length of\none plane (mm)")
                              n940 = Select(t=w2312, s=w2313, f=0.04 ("Length of\nall planes (mm)")) -> (s? t:f=w2310:dbl)
                              n941 = To Double Precision Float(number=w2314) -> (double precision float=w2317:dbl)
                              n942 = property on="Length of\none plane (mm)" class="DigNum (strict)"() -> ("Value"=w2321:dbl)  [unwired: 2 in, 2 out]
                              n943 = expression code="x*1e-3"(w2317) -> (w2318:dbl)
                              n944 = property on="Length of\nall planes (mm)" class="DigNum (strict)"("Value"=w2310) -> ()  [unwired: 2 in, 2 out]
                              n945 = To Double Precision Float(number=w2322) -> (double precision float=w2324:dbl)
                              n946 = Divide(x=w2310, y=w2318) -> (x/y=w2319:dbl)
                              n947 = expression code="x*1e-3"(w2324) -> (w2325:dbl)
                              n948 = Round To Nearest(number=w2319) -> (nearest integer value=w2316:dbl)
                              n949 = Increment(x=w2316) -> (x+1=w2315:dbl)
                              n950 = Divide(x=w2321, y=w2325) -> (x/y=w2326:dbl)
                              n951 = Round To Nearest(number=w2326) -> (nearest integer value=w2323:dbl)
                              n952 = Increment(x=w2323) -> (x+1=w2320:dbl)
                            }
                            frame "250 MHz" {
                              w2333 = sgl 1.0
                              w2341 = 2.0 ("Length of\none plane (mm)")
                              n953 = Select(t=w2331, s=w2332, f=0.04 ("Length of\nall planes (mm)")) -> (s? t:f=w2329:dbl)
                              n954 = To Double Precision Float(number=w2333) -> (double precision float=w2336:dbl)
                              n955 = property on="Length of\none plane (mm)" class="DigNum (strict)"() -> ("Value"=w2340:dbl)  [unwired: 2 in, 2 out]
                              n956 = property on="Length of\nall planes (mm)" class="DigNum (strict)"("Value"=w2329) -> ()  [unwired: 2 in, 2 out]
                              n957 = expression code="x*1e-3"(w2336) -> (w2337:dbl)
                              n958 = To Double Precision Float(number=w2341) -> (double precision float=w2343:dbl)
                              n959 = Divide(x=w2329, y=w2337) -> (x/y=w2338:dbl)
                              n960 = expression code="x*1e-3"(w2343) -> (w2344:dbl)
                              n961 = Round To Nearest(number=w2338) -> (nearest integer value=w2335:dbl)
                              n962 = Increment(x=w2335) -> (x+1=w2334:dbl)
                              n963 = Divide(x=w2340, y=w2344) -> (x/y=w2345:dbl)
                              n964 = Round To Nearest(number=w2345) -> (nearest integer value=w2342:dbl)
                              n965 = Increment(x=w2342) -> (x+1=w2339:dbl)
                            }
                          }
                        }
                      }
                    }
                  }
                  n966 = call "Force Odd or Even.vi"("Parity (odd)"=enum16{"Odd", "Even"}."Odd" ("Parity"), "input"=w2131) -> ("output"=w2130:i32)
                  n967 = Bundle By Name(cluster=w2142, "lines per plane"=w2130) -> (w2132:T13)
                  n968 = call "Force Odd or Even.vi"("Parity (odd)"=enum16{"Odd", "Even"}."Odd" ("Parity"), "input"=w2139) -> ("output"=w2133:i32)
                  n969 = Bundle By Name(cluster=w2147, "scan pair"=w2136, "Distance between\nscan lines (um)"=w2135, "Distance between\nscan planes (um)"=w2134, "number of scan planes"=w2133) -> (w2137:T10)
                  n970 = property on="lines per plane" class="DigNum (strict)"("Val(Sgnl)"=w2130) -> ()  [unwired: 2 in, 2 out]
                  n971 = property on="Distance between\nplanes (um)" class="DigNum (strict)"("Val(Sgnl)"=w2134) -> ()  [unwired: 2 in, 2 out]
                  n972 = property on="number of planes" class="DigNum (strict)"("Val(Sgnl)"=w2133) -> ()  [unwired: 2 in, 2 out]
                  n973 = property on="Distance between\nscan lines (um)" class="DigNum (strict)"("Val(Sgnl)"=w2135) -> ()  [unwired: 2 in, 2 out]
                  n974 = property on="scan pair" class="Enum (strict)"("Val(Sgnl)"=w2136) -> ()  [unwired: 2 in, 2 out]
                }
                event "Attenuation Scan", "Length of Z \nScan (mm)", "Distance between\nZ planes (um)": Value Change {
                  w2352 = ScanAxis."x-(z) scan"  # scan pair
                  n975 = event-data() -> ()  [unwired: 3 out]
                  n976 = Not(x="Attenuation Scan") -> (.not. x?=w2351:bool)
                  n977 = property on="Skip Real \nTime Setup" class="Bool (strict)"("Value"="Attenuation Scan", "Visible"=w2351) -> ()  [unwired: 2 in, 2 out]
                  n978 = property on="Fix Z \nDelay?" class="Bool (strict)"("Val(Sgnl)"="Attenuation Scan") -> ()  [unwired: 2 in, 2 out]
                  n979 = control-ref of="Length of\nall planes (mm)"() -> (w2360:refnum<vi>)
                  n980 = control-ref of="Length of\none plane (mm)"() -> (w2361:refnum<vi>)
                  n981 = control-ref of="Distance between\nscan lines (um)"() -> (w2359:refnum<vi>)
                  n982 = control-ref of="Case Name"() -> (w2358:refnum<vi>)
                  n983 = control-ref of="DBSP2"() -> (w2356:refnum<vi>)
                  n984 = control-ref of="DBSP1"() -> (w2357:refnum<vi>)
                  n985 = control-ref of="Scan Size"() -> (w2349:refnum<vi>)
                  n986 = control-ref of="Transducer"() -> (w2355:refnum<vi>)
                  n987 = call "Dual XDCR AttnScan.vi"("Length of\none plane (mm)"=w2361, "Distance between\nscan lines (um)"=w2359, "Case Name"=w2358, 4:"DBSP2"=w2357, 5:"DBSP1"=w2356, "Length of\nall planes (mm)"=w2360, "Scan Size"=w2349, "Length of Z Scan (mm)"="Length of Z \nScan (mm)", "Distance between\nZ planes (um)"="Distance between\nZ planes (um)", "scan pair"=w2352, "Transducer"=w2355, "Attenuation Scan"="Attenuation Scan", 15:"DBSP1"="DBSP1", 17:"DBSP2"="DBSP2", "Dual XDCR Settings in"=w2363) -> ("scan pair out"=w2370:T12, "lines per plane"=w2365:dbl, "Distance between\nscan lines (um)"=w2369:sgl, "number of planes"=w2374:dbl, "Distance between\nscan planes (um)"=w2368:sgl, "Dual XDCR Settings out"=w2362:T24)  [unwired: 7 in]
                  n988 = call "Force Odd or Even.vi"("Parity (odd)"=enum16{"Odd", "Even"}."Odd" ("Parity"), "input"=w2365) -> ("output"=w2364:i32)
                  n989 = Bundle By Name(cluster=w2376, "lines per plane"=w2364) -> (w2366:T13)
                  n990 = call "Force Odd or Even.vi"("Parity (odd)"=enum16{"Odd", "Even"}."Odd" ("Parity"), "input"=w2374) -> ("output"=w2367:i32)
                  n991 = Bundle By Name(cluster=w2378, "scan pair"=w2370, "Distance between\nscan lines (um)"=w2369, "Distance between\nscan planes (um)"=w2368, "number of scan planes"=w2367) -> (w2371:T10)
                  n992 = property on="lines per plane" class="DigNum (strict)"("Value"=w2364) -> ()  [unwired: 2 in, 2 out]
                  n993 = property on="Distance between\nplanes (um)" class="DigNum (strict)"("Value"=w2368) -> ()  [unwired: 2 in, 2 out]
                  n994 = property on="number of planes" class="DigNum (strict)"("Value"=w2367) -> ()  [unwired: 2 in, 2 out]
                  n995 = property on="Distance between\nscan lines (um)" class="DigNum (strict)"("Value"=w2369) -> ()  [unwired: 2 in, 2 out]
                  n996 = property on="scan pair" class="Enum (strict)"("Value"=w2370) -> ()  [unwired: 2 in, 2 out]
                }
                event "Next Scan": Value Change {
                  n997 = event-data() -> ()  [unwired: 2 out]
                  n998 = property on="Next Scan" class="Bool (strict)"("Value"=FALSE ("Next Scan")) -> ()  [unwired: 2 in, 2 out]
                  n999 = property on="Microscopy Scan Mode" class="RadioBtnsControl (strict)"() -> (error out=w2382:errorcluster, "Value"=w2381:T7)  [unwired: 2 in, 1 out]
                  n1000 = Increment(x=w2381) -> (x+1=w2380:T7)
                  n1001 = property on="Microscopy Scan Mode" class="RadioBtnsControl (strict)"(error in=w2382, "Val(Sgnl)"=w2380) -> ()  [unwired: 1 in, 2 out]
                }
                event "New Sample": Value Change {
                  n1002 = event-data() -> ()  [unwired: 3 out]
                  n1003 = property on="HF XDCR" class="Enum (strict)"() -> ("Value"=w2397:T6)  [unwired: 2 in, 2 out]
                  n1004 = property on="Case Name" class="Str"() -> ("Value"=w2400:string)  [unwired: 2 in, 2 out]
                  n1005 = call "GetSampleName.vi"("Transducer"=w2397, "Sanmple Name"=w2400) -> ("Canceled"=w2395:bool, "Transducer"=w2396:T6, "Name"=w2399:string)  [unwired: 1 in]
                  n1006 = Equal?(x=w2396, y=w2397) -> (x = y?=w2398:bool)
                  n1007 = property on="New Sample" class="Bool (strict)"("Value"=FALSE ("New Sample")) -> ()  [unwired: 2 in, 2 out]
                  n1008 = flat-sequence {
                    tunnel: w2399 -> [w2411]
                    tunnel: w2398 -> [w2410]
                    tunnel: w2396 -> [w2409]
                    tunnel: w2395 -> [w2408]
                    tunnel: [w2407] -> w2394
                    tunnel: [w2406] -> w2392
                    tunnel: w2391 -> [w2406]
                    tunnel: w2394 -> [w2418]
                    tunnel: [w2417] -> w2393
                    tunnel: w2392 -> [w2416]
                    frame #0 {
                      n1009 = case shown="False" w2408 {
                        selector: w2408 -> [w2412 w2414]
                        tunnel: [w2412 w2414] -> w2407
                        frame False {
                          n1010 = property on="Microscopy Scan Mode" class="RadioBtnsControl (strict)"("Val(Sgnl)"=T7."Level X" ("Value (Signaling)")) -> ()  [unwired: 2 in, 2 out]
                        }
                        frame True {
                        }
                      }
                      n1011 = case shown="False" w2410 {
                        tunnel: w2409 -> [w2415 _]
                        frame False {
                          n1012 = property on="HF XDCR" class="Enum (strict)"("Val(Sgnl)"=w2415) -> ()  [unwired: 2 in, 2 out]
                        }
                        frame True {
                        }
                      }
                      n1013 = property on="Case Name" class="Str"("Value"=w2411) -> ()  [unwired: 2 in, 2 out]
                    }
                    frame #1 {
                      n1014 = case shown="False" w2418 {
                        selector: w2418 -> [w2424 _]
                        tunnel: [w2420 w2425] -> w2417
                        tunnel: w2416 -> [w2421 w2425]
                        frame False {
                          w2423 = i16 0 ("Microscopy Overview Counter")
                          n1015 = Decrement(x=w2423) -> (x-1=w2422:i16)
                          n1016 = global write "MotionGlobals.vi" "2D Counter"(w2423) -> ()
                          n1017 = global write "MotionGlobals.vi" "Overview Counter"(w2423) -> ()
                          n1018 = global write "MotionGlobals.vi" "Vz Counter"(w2422) -> ()
                          n1019 = Bundle By Name(cluster=w2421, "rf points per line"=200) -> (w2420:T13)
                          n1020 = property on="SetDig" class="Bool (strict)"("Val(Sgnl)"=w2424) -> ()  [unwired: 2 in, 2 out]
                        }
                        frame True {
                        }
                      }
                    }
                  }
                }
                event "Pulse": Value Change {
                  n1021 = event-data() -> ()  [unwired: 2 out]
                  n1022 = case shown="True" "Pulse" {
                    tunnel: w2427 -> [w2435 w2442]
                    tunnel: w2426 -> [w2434 _]
                    frame False {
                      n1023 = flat-sequence {
                        tunnel: w2435 -> [w2437]
                        tunnel: w2434 -> [w2436]
                        frame #0 {
                          n1024 = call "PRF_Off.vi"("Location"=w2436, "Motion Settings In"=w2437) -> ()  [unwired: 9 in, 1 out]
                        }
                        frame #1 {
                          n1025 = Wait (ms)(milliseconds to wait=u32 50) -> ()  [unwired: 1 out]
                        }
                      }
                    }
                    frame True {
                      n1026 = global read "MotionGlobals.vi" "Multi Trig?"() -> (w2440:bool)
                      n1027 = global read "MotionGlobals.vi" "CTR PRF?"() -> (w2441:bool)
                      n1028 = global read "PulserGlobals.vi" "prf (kHz)"() -> (w2439:dbl)
                      n1029 = call "PRF_Set.vi"("Motion Settings In"=w2442, "prf (kHz)"=w2439, "Multi Trig?"=w2440, "CTR PRF?"=w2441) -> ()  [unwired: 8 in]
                    }
                  }
                }
                event "Auto Vz?": Value Change {
                  n1030 = event-data() -> ()  [unwired: 2 out]
                  n1031 = case shown="True" "Auto Vz?" {
                    tunnel: [T45."Enabled" ("Disabled") T45."Disabled and Grayed Out" ("Disabled")] -> w2444
                    frame False {
                    }
                    frame True {
                    }
                  }
                  n1032 = property on="Auto Vz Depth" class="DigNum (strict)"("Visible"="Auto Vz?") -> ()  [unwired: 2 in, 2 out]
                  n1033 = property on="V-Z Scan" class="Bool (strict)"("DisabledEnum"=w2444) -> ()  [unwired: 2 in, 2 out]
                }
                event "C MIP": Value Change {
                  n1034 = event-data() -> ()  [unwired: 2 out]
                  n1035 = local read "Case to View"() -> (w2475:u16)
                  n1036 = Index Array(array=w2459, index=w2475) -> (element=w2474:T55)
                  n1037 = Unbundle By Name(w2474) -> ("File Name"=w2472:string)
                  n1038 = Concatenate Strings(w2472, "*") -> (w2470:string)
                  n1039 = List Folder(path=w2456, pattern=w2470) -> (path out=w2468:path, filenames=w2467:string[], error out=w2469:errorcluster)  [unwired: 2 in, 1 out]
                  n1040 = case shown="No Error" w2469 {
                    tunnel: w2468 -> [w2483 _]
                    tunnel: w2467 -> [w2482 _]
                    tunnel: [w2481 _] -> w2466
                    tunnel: [w2480 _] -> w2464
                    tunnel: "MIP Thresh" -> [w2479 _]
                    tunnel: [w2477 _] -> w2458
                    frame No Error {
                      n1041 = for {
                        tunnel: w2483 -> [w2491]
                        tunnel: w2482 -> [w2490] mode=indexing
                        tunnel: [w2485] -> w2481 mode=indexing
                        tunnel: [w2487] -> w2480 mode=indexing
                        tunnel: w2479 -> [w2486]
                        tunnel: [w2484] -> w2478
                        n1042 = Build Path(base path=w2491, name or relative path=w2490) -> (appended path=w2489:path)
                        n1043 = call "ReadEyeFileFast.vi"("new file path"=w2489) -> ("2-D data array"=w2488:sgl[][], "Header In"=w2484:T59)  [unwired: 2 in, 15 out]
                        n1044 = for {
                          tunnel: w2488 -> [w2499] mode=indexing
                          tunnel: [w2492] -> w2487 mode=indexing
                          tunnel: w2486 -> [w2498]
                          tunnel: [w2496] -> w2485 mode=indexing
                          w2493 = 0 ("f")
                          n1045 = Array Max & Min(array=w2499) -> (max value=w2497:sgl, max index (indices)=w2494:i32)  [unwired: 2 out]
                          n1046 = Greater?(x=w2497, y=w2498) -> (0:w2495:bool)
                          n1047 = Select(t=w2494, s=w2495, f=w2493) -> (s? t:f=w2492:i32)
                          n1048 = Select(t=w2497, s=w2495, f=w2493) -> (s? t:f=w2496:sgl)
                        }
                      }
                      n1049 = Unbundle By Name(w2478) -> ("A/D info.# A/D bits"=w2477:i16)
                    }
                    frame Error {
                    }
                  }
                  n1050 = Unbundle By Name(w2454) -> ("bits A/D"=w2453:i8)
                  n1051 = case shown="\"dB Scale\"" ScaleMethod."Linear Abs Grey" ("Display mode") {
                    tunnel: w2466 -> [w2501 w2504 w2505 w2508]
                    tunnel: [w2500 w2503 w2505 w2507] -> w2473
                    tunnel: w2458 -> [_ w2502 _ _]
                    tunnel: w2453 -> [_ _ _ w2506]
                    frame "Linear Abs Grey", Default {
                      n1052 = Absolute Value(x=w2501) -> (abs(x)=w2500:sgl[][])
                    }
                    frame "Log Grey Scale" {
                      n1053 = call "LogScaleImage.vi"("A/D bits"=w2502, "input array"=w2504) -> ("log scale image"=w2503:dbl[][])  [unwired: 1 out]
                    }
                    frame "Linear Color Scale" {
                    }
                    frame "dB Scale" {
                      n1054 = call "dBScale.vi"("Bit Depth"=w2506, "Data In"=w2508) -> ("Data Out"=w2507:dbl[][])  [unwired: 3 in]
                    }
                  }
                  n1055 = Transpose 2D Array(2D array=w2473) -> (transposed array=w2463:dbl[][])
                  n1056 = Transpose 2D Array(2D array=w2464) -> (transposed array=w2462:i32[][])
                  n1057 = call "DisplayMAXandTOF.vi"("TOF"=w2462, "Max Value"=w2463) -> ()  [unwired: 10 in]
                }
                event "Set Spectrometer": Value Change {
                  n1058 = event-data() -> ()  [unwired: 2 out]
                  n1059 = global read "MotionGlobals.vi" "Main Spectrometer"() -> (w2514:T61)
                  n1060 = case shown="1" w2514 {
                    frame 0, Default {
                    }
                    frame 1 {
                      # "OceanSetUp_ViewLV"
                    }
                  }
                }
                event "Save Scan Settings", "Load Scan Settings": Value Change {
                  n1061 = event-data() -> ()  [unwired: 2 out]
                  n1062 = case shown="True" "Save Scan Settings" {
                    tunnel: w2552 -> [w2591 w2598]
                    tunnel: [w2591 w2597] -> w2558
                    tunnel: w2537 -> [w2590 w2596]
                    tunnel: [w2590 w2595] -> w2557
                    tunnel: w2555 -> [w2589 w2594]
                    tunnel: [w2589 w2593] -> w2554
                    frame False {
                    }
                    frame True {
                      n1063 = property on="Case Name" class="Str"() -> ("Value"=w2592:string)  [unwired: 2 in, 2 out]
                      n1064 = call "SaveScanSettings.vi"("Type of scan"=w2594, "Digitizer Settings"=w2596, "Motion Settings"=w2598, "Case Name Modifier"=w2592) -> ("Type of scan out"=w2593:T21, "Digitizer Settings out"=w2595:T13, "Motion Settings out"=w2597:T10)
                    }
                  }
                  n1065 = Unbundle By Name(w2552) -> ("Motion System"=w2539:T11, "Motion Bd ID"=w2540:u8, "Motion Profile"=w2541:string, "# Axis"=w2542:i8, "Reverse Z axis?"=w2543:bool, "SMAC Axis"=w2518:u16, "RT fps"=w2544:sgl, "Steps per mm"=w2545:i32[], "Motor Parameters"=w2546:T62, "Global Position (mm)"=w2547:dbl[], "Plane"=w2548:i32, "BKPT Shift"=w2549:i32, "Scan Start Time (ms)"=w2550:u32, "ESP VISA"=w2551:refnum<visa-resource-name>, "3rd Axis"=w2520:T5)
                  n1066 = case shown="True" "Load Scan Settings" {
                    tunnel: [w2571 w2581] -> w2538
                    tunnel: [w2570 w2580] -> w2556
                    tunnel: w2558 -> [w2571 w2574]
                    tunnel: w2557 -> [w2570 w2573]
                    tunnel: w2554 -> [w2569 _]
                    tunnel: [w2569 w2579] -> w2553
                    tunnel: w2527 -> [_ _]
                    tunnel: [FALSE ("Canceled") w2572] -> w2526
                    frame False {
                    }
                    frame True {
                      n1067 = call "LoadScanSettings.vi"("Digitizer Settings In"=w2573, "Motion Settings In"=w2574) -> ("Canceled"=w2572:bool, "Type of scan out"=w2579:T21, "Digitizer Settings out"=w2580:T13, "Motion Settings out"=w2581:T10, "Panametrics Settings Out"=w2576:T27, "Daxsonics Settings Out"=w2577:T26, "Case Name Modifier Out"=w2575:string, "Pulser Out"=w2578:T53)  [unwired: 2 in]
                      n1068 = case shown="False" w2572 {
                        tunnel: w2578 -> [w2585 _]
                        tunnel: w2577 -> [w2584 _]
                        tunnel: w2576 -> [w2583 _]
                        tunnel: w2575 -> [w2582 _]
                        frame False {
                          n1069 = case shown="\"Pan 5900\", Default" w2585 {
                            tunnel: w2584 -> [_ w2588]
                            tunnel: w2583 -> [w2586 _]
                            frame "Pan 5900", Default {
                              n1070 = global read "PulserGlobals.vi" "Panametrics"() -> (w2587:refnum<visa-resource-name>)
                              n1071 = call "5900PRQuickSet.vi"("VISA resource name"=w2587, "Panametrics Settings"=w2586) -> ()  [unwired: 2 in, 1 out]
                            }
                            frame "Daxsonics" {
                              n1072 = call "Set_Daxsonics_3Pulsers.vi"("Daxsonics Settings"=w2588) -> ()  [unwired: 9 in]
                            }
                          }
                          n1073 = global write "PulserGlobals.vi" "Pulser"(w2585) -> ()
                          n1074 = property on="Case Name" class="Str"("Value"=w2582) -> ()  [unwired: 2 in, 2 out]
                        }
                        frame True {
                        }
                      }
                    }
                  }
                  n1075 = Unbundle By Name(w2537) -> ("bits A/D"=w2521:i8, "Avg Num"=w2522:i32, "Dig Ch"=w2523:i32, "LeCroyCluster"=w2524:T63, "Main Digitizer"=w2525:T14, "Dig Config"=w2533:T15, "Digitizer ID Cluster"=w2532:T16, "Data Ref RF"=w2531:refnum<data-value>, "NI ID/Channel"=w2530:cluster{"NI ID":refnum<k15>, "NI CH":i32}[], "Total Dig CH"=w2529:i32, "Data Ref Log"=w2528:refnum<data-value>)
                  n1076 = Bundle By Name(cluster=w2538, "Motion System"=w2539, "Motion Bd ID"=w2540, "Motion Profile"=w2541, "# Axis"=w2542, "Reverse Z axis?"=w2543, "SMAC Axis"=w2518, "RT fps"=w2544, "Steps per mm"=w2545, "Motor Parameters"=w2546, "Global Position (mm)"=w2547, "Plane"=w2548, "BKPT Shift"=w2549, "Scan Start Time (ms)"=w2550, "ESP VISA"=w2551, "3rd Axis"=w2520) -> (w2519:T10)
                  n1077 = Bundle By Name(cluster=w2556, "bits A/D"=w2521, "Avg Num"=w2522, "Dig Ch"=w2523, "LeCroyCluster"=w2524, "Main Digitizer"=w2525, "Dig Config"=w2533, "Digitizer ID Cluster"=w2532, "Data Ref RF"=w2531, "NI ID/Channel"=w2530, "Total Dig CH"=w2529, "Data Ref Log"=w2528) -> (w2534:T13)
                  n1078 = flat-sequence {
                    tunnel: w2553 -> [w2564]
                    tunnel: w2526 -> [w2563]
                    tunnel: [w2567] -> w2536
                    tunnel: w2519 -> [w2567]
                    tunnel: [w2566] -> w2535
                    tunnel: w2534 -> [w2566]
                    frame #0 {
                      n1079 = case shown="False" w2563 {
                        tunnel: w2564 -> [w2565 _]
                        frame False {
                          n1080 = property on="Type of scan" class="Enum (strict)"("Val(Sgnl)"=w2565) -> ()  [unwired: 2 in, 2 out]
                        }
                        frame True {
                        }
                      }
                    }
                    frame #1 {
                    }
                  }
                }
                event "ExitSendCmd": Value Change {
                  n1081 = event-data() -> ()  [unwired: 7 out]
                  n1082 = Index Array(array=w2605) -> (element=w2602:T55)  [unwired: 1 in]
                  n1083 = Unbundle By Name(w2602) -> ("Keep?"=w2601:bool)
                  n1084 = case shown="True" w2601 {
                    tunnel: w2605 -> [w2612 w2620]
                    tunnel: [w2612 w2619] -> w2604
                    tunnel: w2603 -> [_ w2618]
                    tunnel: [TRUE w2614] -> w2600
                    tunnel: w2599 -> [_ w2613]
                    frame False {
                    }
                    frame True {
                      n1085 = call <vilib>:"Three Button Dialog.vi"("Right Button Text (\"Cancel\")"="Cancel" ("Right Button Text (\"Cancel\")"), "Center Button Text (\"No\")"="Exit Without Saving" ("F button name (\"Cancel\")"), "Left Button Text (\"Yes\")"="Save Now" ("T button name (\"OK\")"), "message"="Unsaved Data Exists") -> ("Which Button?"=w2621:T64)  [unwired: 7 in]
                      n1086 = case shown="\"Left Button\", Default" w2621 {
                        tunnel: w2620 -> [w2628 w2629 w2632]
                        tunnel: [w2625 w2629 w2632] -> w2619
                        tunnel: w2618 -> [w2626 _ _]
                        tunnel: [w2624 FALSE TRUE] -> w2614
                        tunnel: w2613 -> [w2627 _ _]
                        frame "Left Button", Default {
                          n1087 = control-ref of="Erase data"() -> (w2623:refnum<vi>)
                          n1088 = call "SaveDataAcqCont.vi"("Boolean in"=w2623, "Array in"=w2628, "Location"=w2627, "Type of scan"=w2626) -> ("Array out"=w2625:T55[], "Aborted"=w2624:bool)  [unwired: 6 in]
                        }
                        frame "Right Button", "Window Close" {
                        }
                        frame "Center Button" {
                        }
                      }
                    }
                  }
                }
              }
            }
          }
          frame #5 {
            n1089 = Request Deallocation(TRUE) -> ()
            n1090 = global read "MotionGlobals.vi" "No GPIB?"() -> (w2636:bool)
            n1091 = case shown="\"WCM Main\", Default" w2634 {
              frame "WCM Main", Default {
                n1092 = global read "MotionGlobals.vi" "DAQmx Task 1"() -> (w2639:refnum<k21>)
                n1093 = call <vilib>:"DAQmx Clear Task.vi"("task in"=w2639) -> ()  [unwired: 1 in, 14 out]
              }
              frame "Hawaii" {
              }
            }
            n1094 = case shown="False" w2636 {
              tunnel: w2638 -> [w2640 _]
              tunnel: w2637 -> [w2643 _]
              tunnel: w2633 -> [w2642 _]
              frame False {
                # "Shut off Agilent 33250A when done."
                n1095 = case shown="True" w2642 {
                  tunnel: [w2644 w2647] -> w2641
                  tunnel: w2643 -> [w2644 w2646]
                  frame False {
                  }
                  frame True {
                    (unwired) "OUTP OFF"
                    n1096 = VISA Write(VISA resource name=w2646, write buffer="") -> (VISA resource name out=w2647:refnum<visa-resource-name>)  [unwired: 1 in, 2 out]
                  }
                }
                n1097 = VISA Close(VISA resource name=w2640) -> ()  [unwired: 1 in, 1 out]
                n1098 = VISA Close(VISA resource name=w2641) -> ()  [unwired: 1 in, 1 out]
              }
              frame True {
              }
            }
          }
        }
      }
    }
  }
  "Digitizer Settings Out" <- w4
  "Motion Settings Out" <- w3
  n1099 = global write "MotionGlobals.vi" "Motion Settings"(w3) -> ()
  n1100 = global write "DigitizerGlobals.vi" "Digitizer Settings"(w4) -> ()
  n1101 = global write "SwitchGlobals.vi" "Dual XDCR Settings"(w5) -> ()
  n1102 = global write "AnnularArrayGlobal.vi" "Ann Array Params"(w2) -> ()
